vi "Run_old.vi"(8 "error in (no error)":errorcluster, 11 "Channel in":refnum<class "Channel.lvclass">) -> (0 "error out":errorcluster, 3 "Channel out":refnum<class "Channel.lvclass">)   [LabVIEW 2018, in "Channel.lvclass"]
uses:
  Channel.lvclass
  C:/Users/observer/Desktop/Sparc4GUI/SPARC4_GUI/Device/Device.lvclass
  Channel.lvclass/Channel.ctl
  Interface/Interface.lvclass/Interface.ctl
  Device/Device.lvclass/Device.ctl
  StateMachine/State Machine.lvclass
  Interface/Interface.lvclass
  Device/Device.lvclass
panel:
  out "resp RESUME":string
  out "resp PAUSE":string
  out "error out 2":errorcluster
  out "x = y?":T1
  out "resp ABORT":string
  out "resp STOP":string
  out "resposta do STATUS":string
  out "resp INIT":string
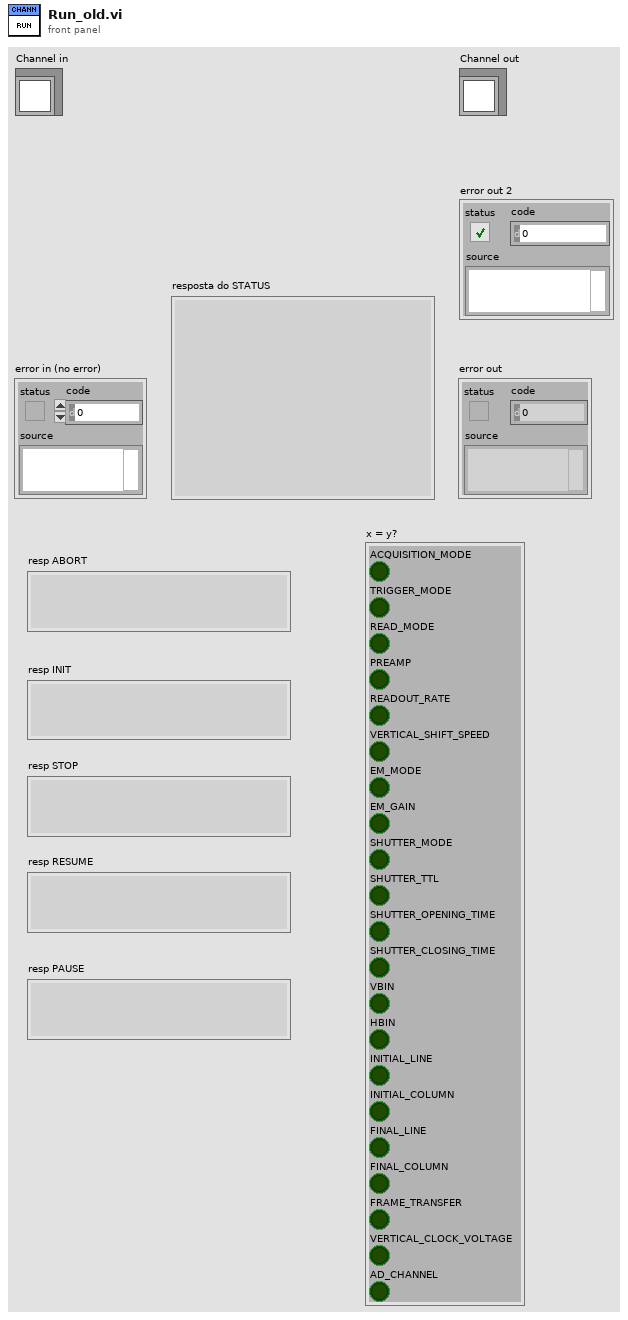
[diagram p1: front panel]
types:
  T1 = cluster{"ACQUISITION_MODE":bool, "TRIGGER_MODE":bool, "READ_MODE":bool, "PREAMP":bool, "READOUT_RATE":bool, "VERTICAL_SHIFT_SPEED":bool, "EM_MODE":bool, "EM_GAIN":bool, "SHUTTER_MODE":bool, "SHUTTER_TTL":bool, "SHUTTER_OPENING_TIME":bool, "SHUTTER_CLOSING_TIME":bool, "VBIN":bool, "HBIN":bool, "INITIAL_LINE":bool, "INITIAL_COLUMN":bool, "FINAL_LINE":bool, "FINAL_COLUMN":bool, "FRAME_TRANSFER":bool, "VERTICAL_CLOCK_VOLTAGE":bool, "AD_CHANNEL":bool}
  T2 = cluster{"ACQUISITION_MODE":u8, "TRIGGER_MODE":u8, "READ_MODE":u8, "PREAMP":u8, "READOUT_RATE":u8, "VERTICAL_SHIFT_SPEED":u8, "EM_MODE":u8, "EM_GAIN":u16, "SHUTTER_MODE":u8, "SHUTTER_TTL":u8, "SHUTTER_OPENING_TIME":u16, "SHUTTER_CLOSING_TIME":u16, "VBIN":u16, "HBIN":u16, "INITIAL_LINE":u16, "INITIAL_COLUMN":u16, "FINAL_LINE":u16, "FINAL_COLUMN":u16, "FRAME_TRANSFER":bool, "VERTICAL_CLOCK_VOLTAGE":u8, "AD_CHANNEL":u32}
  T3 = cluster{"Image Name":string, "Image Path":string, "#FRAMES":u32, "EXPTIME":dbl, "PREAMP":u8, "READOUT_RATE":u8, "VERTICAL_SHIFT_SPEED":u8, "ACQUISITION_MODE":u8, "READ_MODE":u8, "EM_MODE":u8, "EM_GAIN":u16, "SHUTTER_MODE":u8, "SHUTTER_TTL":u8, "SHUTTER_OPENNING_TIME":u16, "SHUTTER_CLOSING_TIME":u16, "VBIN":u16, "HBIN":u16, "INITIAL_LINE":u16, "INITIAL_COLUMN":u16, "FINAL_LINE":u16, "FINAL_COLUMN":u16, "Cooler ON/OFF":u16, "Set temperature":i8, "Exposições realizadas":u16, "Kinetic Serie Length":u32, "Number of Accumulations":u32, "Kinetic Cycle Time":u32, "FRAME_TRANSFER":bool, "VERTICAL_CLOCK_VOLTAGE":u8, "TRIGGER_MODE":u8, "Number of exp":u32, "AD_CHANNEL":u32}
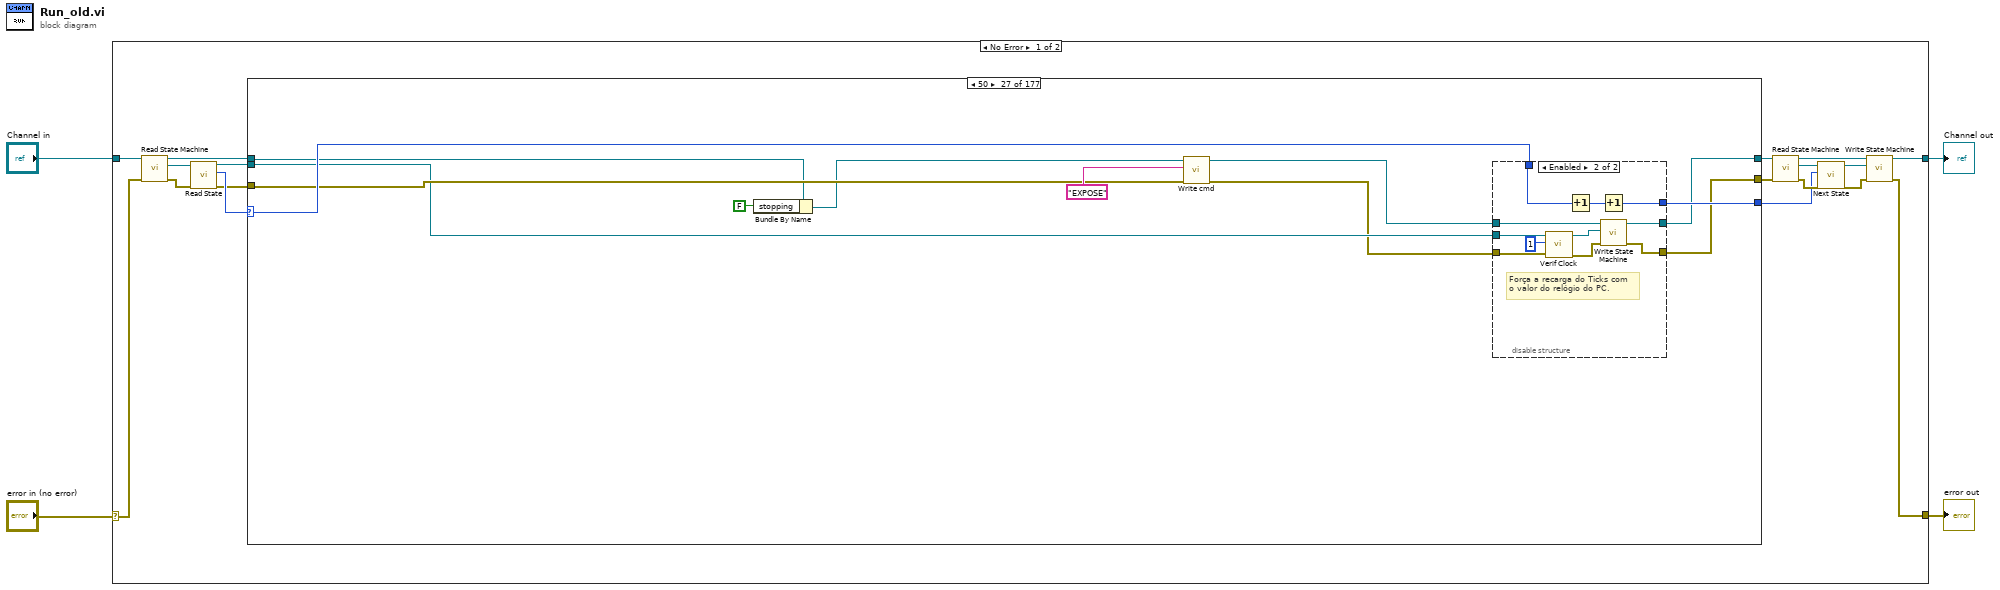
[diagram p0: block diagram]
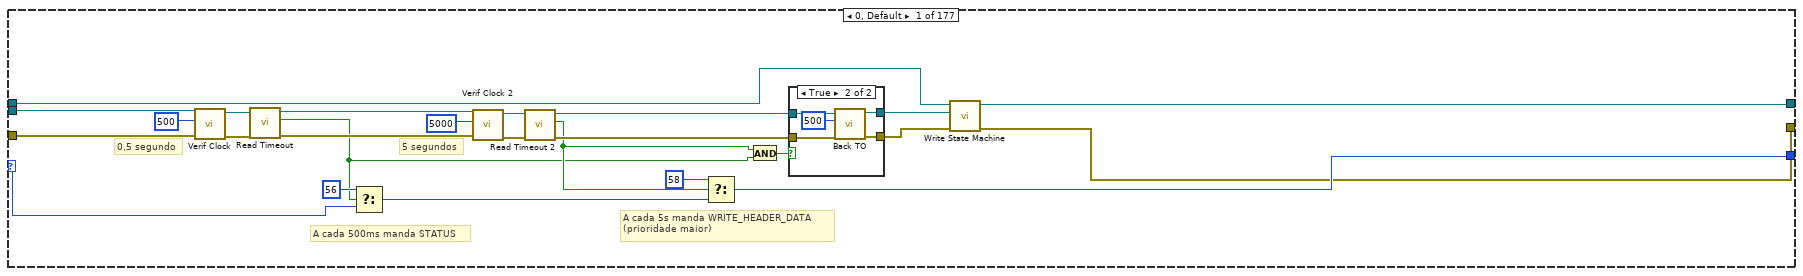
[diagram p2: hidden frame]
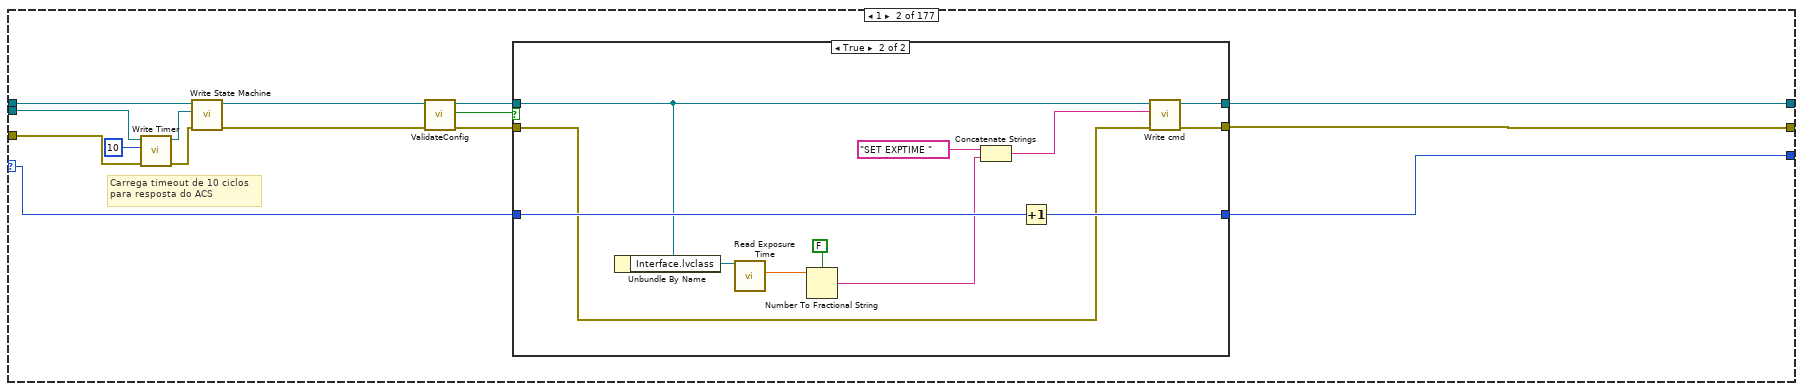
[diagram p4: hidden frame]
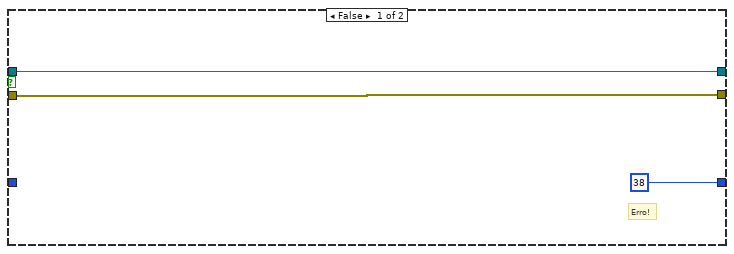
[diagram p5: hidden frame]
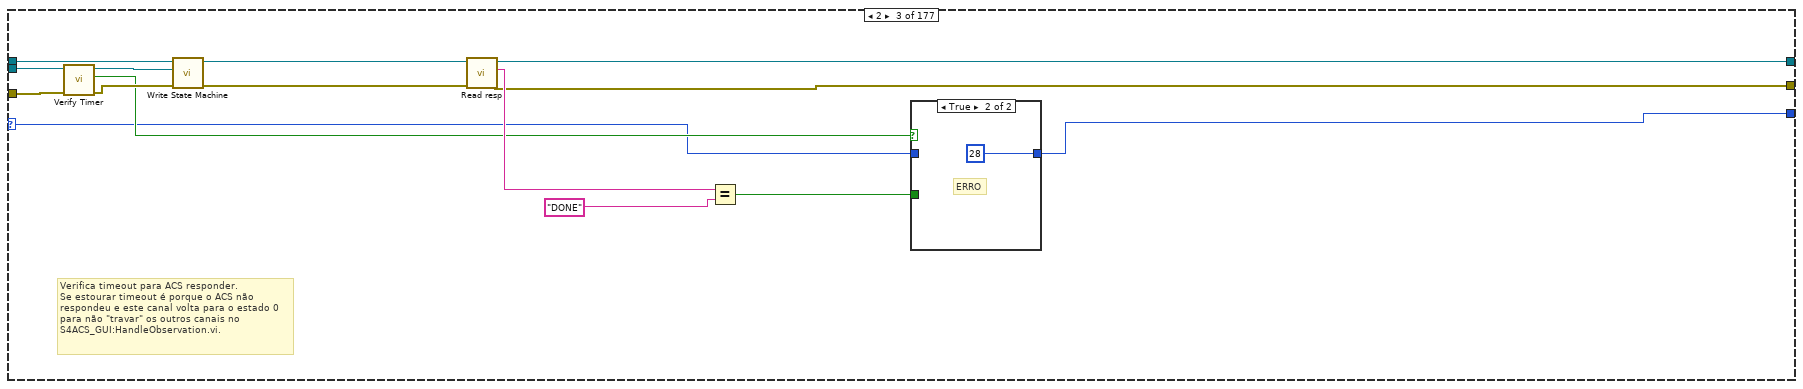
[diagram p6: hidden frame]
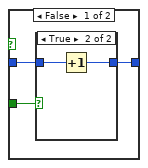
[diagram p7: hidden frame]
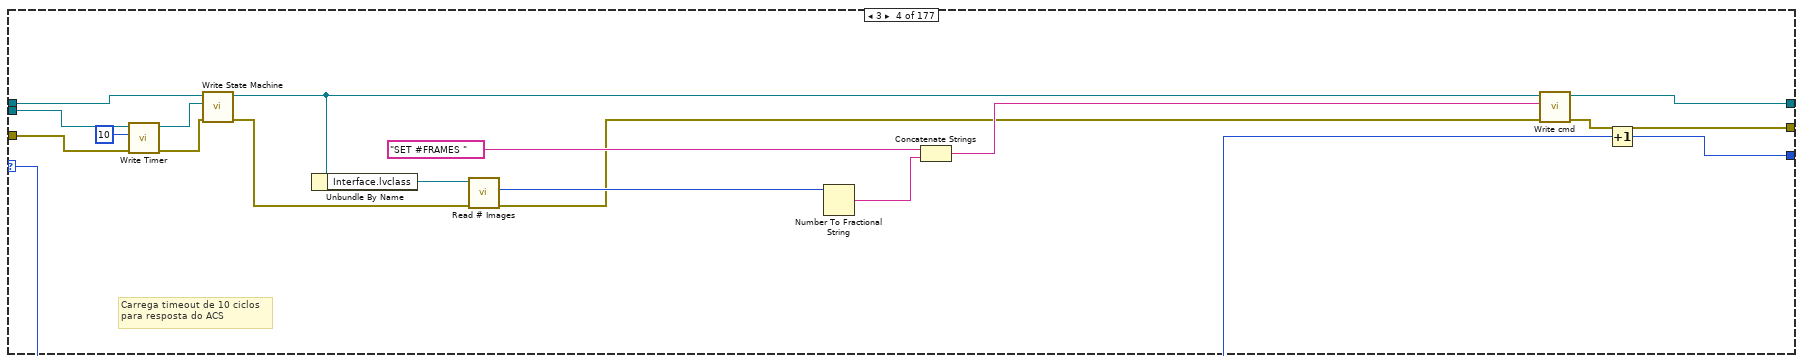
[diagram p9: hidden frame]
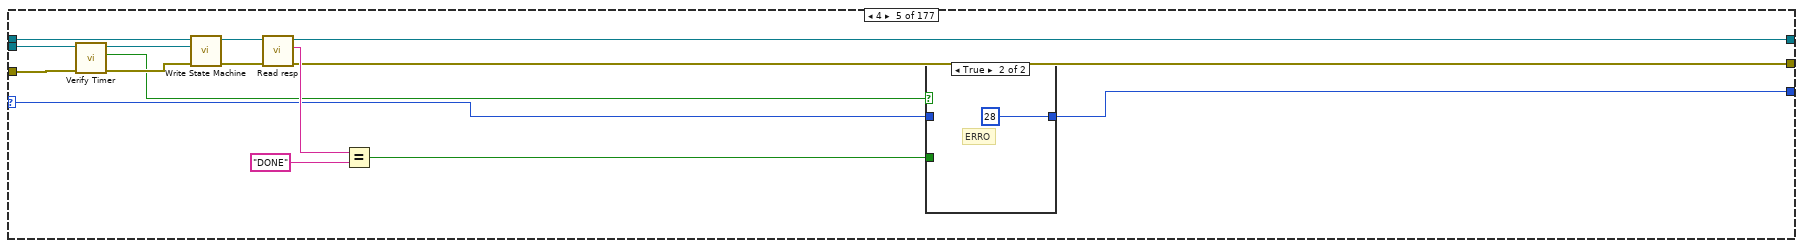
[diagram p10: hidden frame]
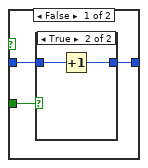
[diagram p11: hidden frame]
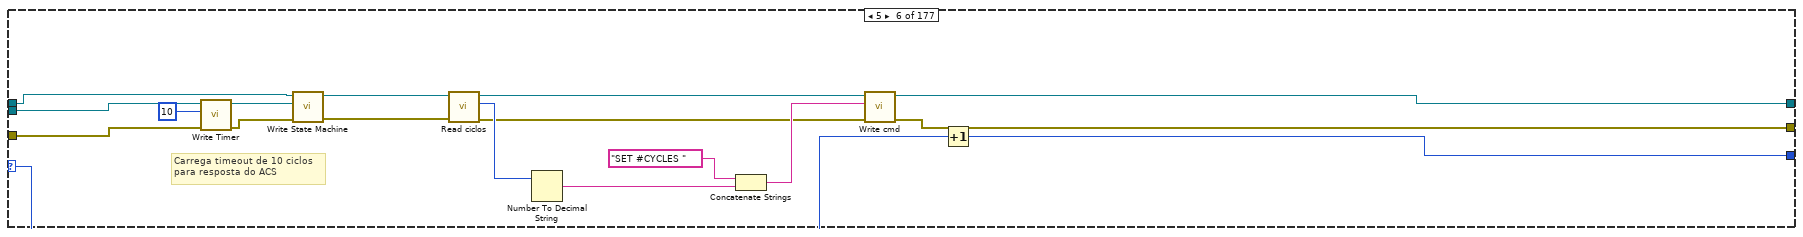
[diagram p13: hidden frame]
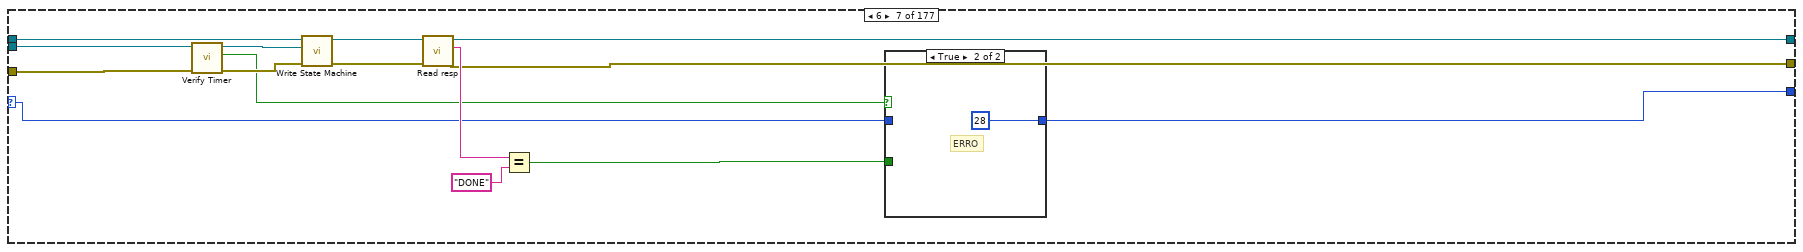
[diagram p14: hidden frame]
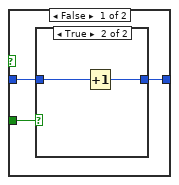
[diagram p15: hidden frame]
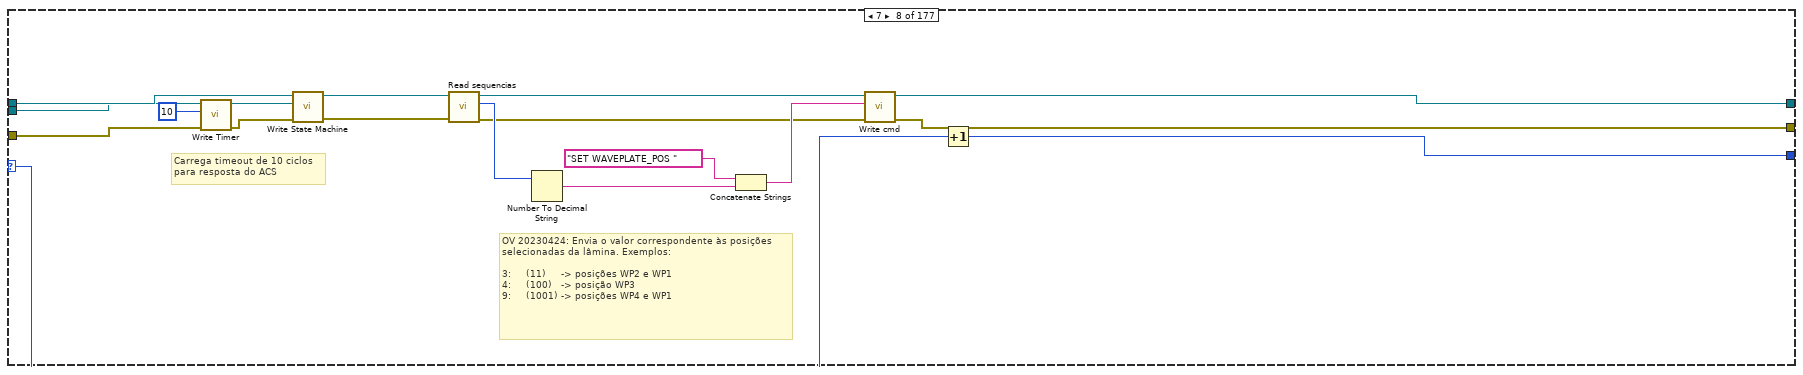
[diagram p17: hidden frame]
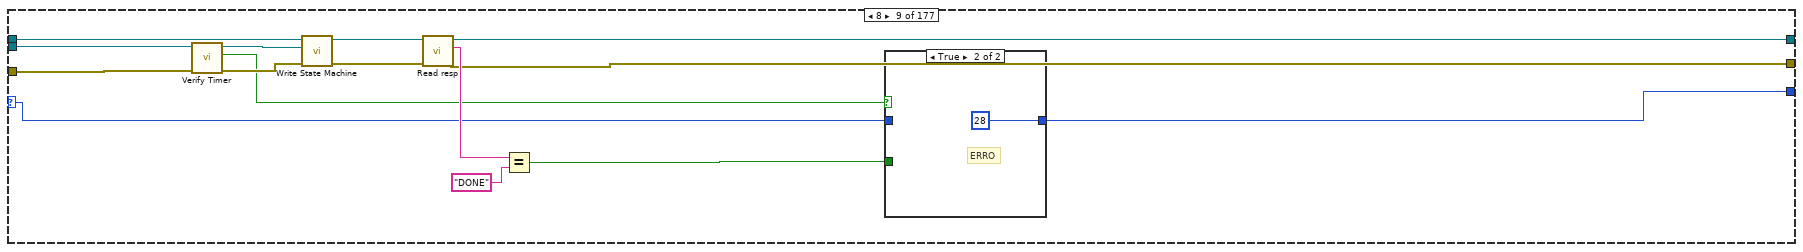
[diagram p18: hidden frame]
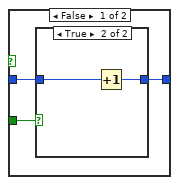
[diagram p19: hidden frame]
diagram:
  n1 = case shown="No Error" "error in (no error)" {
    selector: "error in (no error)" -> [w21 w2909]
    tunnel: [w6 w2909] -> w3
    tunnel: [w11 w2908] -> w1
    tunnel: "Channel in" -> [w22 w2908]
    frame No Error {
      n2 = call-dynamic "Read State Machine.vi"("error in (no error)"=w21, "Device in"=w22) -> ("error out"=w18:errorcluster, "State Machine.lvclass"=w20:refnum<class "State Machine.lvclass">, "Device out"=w16:refnum<class "Channel.lvclass">)  [unwired: 7 in]
      n3 = call-dynamic "Read State.vi"("error in (no error)"=w18, "State Machine in"=w20) -> ("error out"=w17:errorcluster, "State"=w19:i32, "State Machine out"=w5:refnum<class "State Machine.lvclass">)  [unwired: 7 in]
      n4 = case shown="50" w19 {
        selector: w19 -> [w43 w66 w86 w109 w126 w155 w167 w195 w207 w244 w252 w278 w290 w320 w334 w359 w365 w381 w397 w422 w435 w471 w490 _ w518 _ w555 w585 w597 w645 w665 w723 w789 w837 _ _ w928 w960 w989 w1001 w1015 w1020 w1080 w1102 w1140 w1146 w1160 w1168 w1182 w1189 w1200 _ w1215 w1226 w1246 w1266 w1286 w1306 w1326 w1346 w1366 w1386 _ w1406 w1414 w1427 w1440 w1456 w1464 w1477 w1491 w1503 w1511 w1524 w1537 w1549 w1557 w1570 w1583 w1595 w1603 w1616 w1629 w1641 w1649 w1662 w1675 w1687 w1695 w1708 w1721 w1733 w1741 w1754 w1767 w1779 w1787 w1800 w1813 w1829 w1837 w1850 w1863 w1875 w1883 w1896 w1909 w1921 w1929 w1942 w1955 w1967 w1975 w1988 w2001 w2013 w2021 w2034 w2047 w2059 w2067 w2080 w2093 w2105 w2113 w2126 w2139 w2151 w2159 w2172 w2185 w2197 w2205 w2218 w2231 w2243 w2251 w2264 w2277 w2289 w2297 w2310 w2323 w2339 w2347 w2360 w2373 w2385 w2395 w2408 w2421 w2435 w2443 w2456 w2469 w2487 w2502 w2526 w2534 w2565 w2573 w2604 w2612 w2643 w2651 w2682 w2690 w2725 w2738 w2767 w2773 w2799 w2811 w2836 w2848 w2873 w2885]
        tunnel: w17 -> [w41 w65 w92 w111 w130 w157 w169 w197 w209 w229 w254 w280 w292 w322 w336 w361 w363 w373 w396 w417 w429 w481 w489 w511 w520 w531 w552 w578 w594 w602 w662 w682 w781 w809 w871 w903 w936 w948 w983 w996 w1009 w1037 w1077 w1097 w1133 w1150 w1163 w1172 w1185 w1192 w1203 w1212 w1219 w1230 w1241 w1261 w1281 w1301 w1321 w1341 w1361 w1381 w1399 w1412 w1421 w1431 w1443 w1462 w1471 w1481 w1494 w1509 w1518 w1528 w1540 w1555 w1564 w1574 w1586 w1601 w1610 w1620 w1632 w1647 w1656 w1666 w1678 w1693 w1702 w1712 w1724 w1739 w1748 w1758 w1770 w1785 w1794 w1804 w1816 w1835 w1844 w1854 w1866 w1881 w1890 w1900 w1912 w1927 w1936 w1946 w1958 w1973 w1982 w1992 w2004 w2019 w2028 w2038 w2050 w2065 w2074 w2084 w2096 w2111 w2120 w2130 w2142 w2157 w2166 w2176 w2188 w2203 w2212 w2222 w2234 w2249 w2258 w2268 w2280 w2295 w2304 w2314 w2326 w2345 w2354 w2364 w2376 w2391 w2402 w2412 w2424 w2441 w2450 w2460 w2472 w2479 w2500 w2518 w2540 w2558 w2579 w2597 w2618 w2636 w2657 w2675 w2696 w2719 w2744 w2761 w2779 w2801 w2813 w2838 w2850 w2875 w2887]
        tunnel: [w23 w68 w96 w123 w136 w163 w176 w203 w216 w246 w261 w286 w299 w328 w343 w361 w363 w385 w398 w424 w437 w480 w491 w516 w520 w535 w547 w572 w599 w637 w667 w696 w776 w810 w883 w914 w935 w961 w991 w993 w1017 w1021 w1082 w1103 w1121 w1147 w1156 w1169 w1178 w1190 w1196 w1205 w1218 w1227 w1241 w1261 w1281 w1301 w1321 w1341 w1361 w1381 w1399 w1411 w1415 w1430 w1441 w1461 w1465 w1480 w1492 w1508 w1512 w1527 w1538 w1554 w1558 w1573 w1584 w1600 w1604 w1619 w1630 w1646 w1650 w1665 w1676 w1692 w1696 w1711 w1722 w1738 w1742 w1757 w1768 w1784 w1788 w1803 w1814 w1834 w1838 w1853 w1864 w1880 w1884 w1899 w1910 w1926 w1930 w1945 w1956 w1972 w1976 w1991 w2002 w2018 w2022 w2037 w2048 w2064 w2068 w2083 w2094 w2110 w2114 w2129 w2140 w2156 w2160 w2175 w2186 w2202 w2206 w2221 w2232 w2248 w2252 w2267 w2278 w2294 w2298 w2313 w2324 w2344 w2348 w2363 w2374 w2390 w2396 w2411 w2422 w2440 w2444 w2459 w2470 w2491 w2503 w2530 w2543 w2569 w2582 w2608 w2621 w2647 w2660 w2686 w2699 w2728 w2747 w2769 w2782 w2807 w2820 w2844 w2857 w2881 w2894] -> w7
        tunnel: w16 -> [w31 w63 w95 w112 w134 w158 w173 w198 w213 w231 w258 w281 w296 w323 w340 w360 w362 w376 w395 w419 w432 w479 w488 w514 w519 w532 w546 w584 w595 w617 w658 w695 w783 w803 w882 w913 w930 w952 w984 w997 w1010 w1038 w1076 w1100 w1134 w1151 w1162 w1173 w1184 w1193 w1202 w1213 w1217 w1231 w1239 w1259 w1279 w1299 w1319 w1339 w1359 w1379 w1401 w1410 w1422 w1429 w1444 w1460 w1472 w1479 w1495 w1507 w1519 w1526 w1541 w1553 w1565 w1572 w1587 w1599 w1611 w1618 w1633 w1645 w1657 w1664 w1679 w1691 w1703 w1710 w1725 w1737 w1749 w1756 w1771 w1783 w1795 w1802 w1817 w1833 w1845 w1852 w1867 w1879 w1891 w1898 w1913 w1925 w1937 w1944 w1959 w1971 w1983 w1990 w2005 w2017 w2029 w2036 w2051 w2063 w2075 w2082 w2097 w2109 w2121 w2128 w2143 w2155 w2167 w2174 w2189 w2201 w2213 w2220 w2235 w2247 w2259 w2266 w2281 w2293 w2305 w2312 w2327 w2343 w2355 w2362 w2377 w2389 w2403 w2410 w2425 w2439 w2451 w2458 w2473 w2481 w2499 w2520 w2541 w2560 w2580 w2599 w2619 w2638 w2658 w2677 w2697 w2721 w2745 w2763 w2780 w2802 w2817 w2839 w2854 w2876 w2891]
        tunnel: [w30 w69 w97 w124 w137 w164 w177 w204 w217 w247 w262 w287 w300 w329 w344 w360 w362 w386 w399 w425 w440 w472 w492 w517 w519 w536 w548 w573 w600 w644 w668 w722 w777 w836 w884 w915 w937 w962 w992 w994 w1018 w1033 w1083 w1104 w1127 w1148 w1155 w1170 w1177 w1191 w1195 w1211 w1220 w1223 w1243 w1263 w1283 w1303 w1323 w1343 w1363 w1383 w1401 w1413 w1416 w1432 w1439 w1463 w1466 w1482 w1490 w1510 w1513 w1529 w1536 w1556 w1559 w1575 w1582 w1602 w1605 w1621 w1628 w1648 w1651 w1667 w1674 w1694 w1697 w1713 w1720 w1740 w1743 w1759 w1766 w1786 w1789 w1805 w1812 w1836 w1839 w1855 w1862 w1882 w1885 w1901 w1908 w1928 w1931 w1947 w1954 w1974 w1977 w1993 w2000 w2020 w2023 w2039 w2046 w2066 w2069 w2085 w2092 w2112 w2115 w2131 w2138 w2158 w2161 w2177 w2184 w2204 w2207 w2223 w2230 w2250 w2253 w2269 w2276 w2296 w2299 w2315 w2322 w2346 w2349 w2365 w2372 w2392 w2397 w2413 w2420 w2442 w2445 w2461 w2468 w2492 w2504 w2531 w2544 w2570 w2583 w2609 w2622 w2648 w2661 w2687 w2700 w2729 w2748 w2770 w2783 w2808 w2821 w2845 w2858 w2882 w2895] -> w14
        tunnel: [w40 w67 w85 w118 w125 w162 w168 w202 w208 w245 w250 w285 w291 w327 w332 w359 w366 w382 w400 w423 w436 w473 w493 31 ("State") w518 0 ("State") w553 w586 w598 w646 w666 w724 w790 w838 0 ("State") 54 ("State") w927 w963 w990 w1002 w1016 w1019 w1081 w1105 w1141 w1149 w1161 w1171 w1183 w1189 w1201 w1204 w1216 w1228 w1238 w1258 w1278 w1298 w1318 w1338 w1358 w1378 u8 0 ("State") w1407 w1417 w1428 w1442 w1457 w1467 w1478 w1493 w1504 w1514 w1525 w1539 w1550 w1560 w1571 w1585 w1596 w1606 w1617 w1631 w1642 w1652 w1663 w1677 w1688 w1698 w1709 w1723 w1734 w1744 w1755 w1769 w1780 w1790 w1801 w1815 w1830 w1840 w1851 w1865 w1876 w1886 w1897 w1911 w1922 w1932 w1943 w1957 w1968 w1978 w1989 w2003 w2014 w2024 w2035 w2049 w2060 w2070 w2081 w2095 w2106 w2116 w2127 w2141 w2152 w2162 w2173 w2187 w2198 w2208 w2219 w2233 w2244 w2254 w2265 w2279 w2290 w2300 w2311 w2325 w2340 w2350 w2361 w2375 w2386 w2398 w2409 w2423 w2436 w2446 w2457 w2471 w2488 w2505 w2527 w2532 w2566 w2571 w2605 w2610 w2644 w2649 w2683 w2688 w2726 w2736 w2768 w2771 w2806 w2812 w2843 w2849 w2880 w2883] -> w8
        tunnel: w5 -> [w42 w64 w94 w113 w135 w156 w170 w196 w210 w227 w255 w279 w293 w321 w337 _ _ w375 w393 w418 w433 _ w486 w513 _ w533 w551 w582 _ w605 w663 w685 w785 w808 w872 w904 w932 w953 w986 w998 w1012 w1039 w1078 w1101 w1135 _ _ _ _ _ _ w1207 _ _ _ _ _ _ _ _ _ _ _ _ _ _ _ _ _ _ _ _ _ _ _ _ _ _ _ _ _ _ _ _ _ _ _ _ _ _ _ _ _ _ _ _ _ _ _ _ _ _ _ _ _ _ _ _ _ _ _ _ _ _ _ _ _ _ _ _ _ _ _ _ _ _ _ _ _ _ _ _ _ _ _ _ _ _ _ _ _ _ _ _ _ _ _ _ _ _ _ _ _ _ _ w2483 w2501 w2515 w2538 w2554 w2577 w2593 w2616 w2632 w2655 w2671 w2694 w2717 w2742 w2760 w2777 w2800 w2814 w2837 w2851 w2874 w2888]
        frame 0, Default {
          # "5 segundos"
          # "A cada 5s manda WRITE_HEADER_DATA\n(prioridade maior)"
          # "A cada 500ms manda STATUS"
          # "0,5 segundo"
          n5 = call-dynamic "Verif Clock.vi"("error in (no error)"=w41, "period (ms)"=u32 500 ("period"), "State Machine in"=w42) -> ("error out"=w46:errorcluster, "State Machine out"=w45:refnum<class "State Machine.lvclass">)  [unwired: 6 in, 1 out]
          n6 = call-dynamic "Read Timeout.vi"("error in (no error)"=w46, "State Machine in"=w45) -> ("error out"=w35:errorcluster, "Timeout"=w24:bool, "State Machine out"=w37:refnum<class "State Machine.lvclass">)  [unwired: 7 in]
          n7 = Select(t=56 ("State"), s=w24, f=w43) -> (s? t:f=w38:i32)
          n8 = call-dynamic "Verif Clock 2.vi"("error in (no error)"=w35, "period (ms)"=u32 5000 ("period"), "State Machine in"=w37) -> ("error out"=w34:errorcluster, "State Machine out"=w36:refnum<class "State Machine.lvclass">)  [unwired: 6 in, 1 out]
          n9 = call-dynamic "Read Timeout 2.vi"("error in (no error)"=w34, "State Machine in"=w36) -> ("error out"=w32:errorcluster, "Timeout 2"=w25:bool, "State Machine out"=w28:refnum<class "State Machine.lvclass">)  [unwired: 7 in]
          n10 = Select(t=58 ("f"), s=w25, f=w38) -> (s? t:f=w40:i32)
          n11 = And(x=w25, y=w24) -> (x .and. y?=w26:bool)
          n12 = case shown="True" w26 {
            tunnel: w32 -> [w48 w54]
            tunnel: [w48 w53] -> w29
            tunnel: w28 -> [w49 w52]
            tunnel: [w49 w51] -> w27
            frame False {
            }
            frame True {
              n13 = call-dynamic "Back TO.vi"("error in (no error)"=w54, "time back (ms)"=u32 500 ("time(ms)"), "State Machine in"=w52) -> ("error out"=w53:errorcluster, "State Machine out"=w51:refnum<class "State Machine.lvclass">)  [unwired: 7 in]
            }
          }
          n14 = call-dynamic "Write State Machine.vi"("error in (no error)"=w29, "State Machine.lvclass"=w27, "Device in"=w31) -> ("error out"=w23:errorcluster, "Device out"=w30:refnum<class "Channel.lvclass">)  [unwired: 7 in]
        }
        frame 1 {
          # "Carrega timeout de 10 ciclos\npara resposta do ACS"
          n15 = call-dynamic "Write Timer.vi"("error in (no error)"=w65, "Timer"=u32 10, "State Machine in"=w64) -> ("error out"=w60:errorcluster, "State Machine out"=w62:refnum<class "State Machine.lvclass">)  [unwired: 7 in]
          n16 = call-dynamic "Write State Machine.vi"("error in (no error)"=w60, "State Machine.lvclass"=w62, "Device in"=w63) -> ("error out"=w58:errorcluster, "Device out"=w59:refnum<class "Channel.lvclass">)  [unwired: 7 in]
          n17 = call-dynamic "ValidateConfig.vi"("error in (no error)"=w58, "Channel in"=w59) -> ("error out"=w56:errorcluster, "valid?"=w55:bool, "Channel out"=w57:refnum<class "Channel.lvclass">)  [unwired: 7 in]
          n18 = case shown="True" w55 {
            tunnel: [w72 w84] -> w69
            tunnel: [w71 w83] -> w68
            tunnel: [38 w82] -> w67
            tunnel: w66 -> [_ w81]
            tunnel: w57 -> [w72 w74]
            tunnel: w56 -> [w71 w73]
            frame False {
              # "Erro!"
            }
            frame True {
              n19 = Unbundle By Name(w74) -> ("Interface.lvclass"=w80:refnum<class "Interface.lvclass">)
              n20 = call "Read Exposure Time.vi"("Interface in"=w80) -> ("Exposure Time"=w79:dbl)  [unwired: 8 in, 2 out]
              n21 = Number To Fractional String(use system decimal point (T)=FALSE, number=w79) -> (F-format string=w78:string)  [unwired: 2 in]
              n22 = Concatenate Strings("SET EXPTIME " ("cmd"), w78) -> (w77:string)
              n23 = Increment(x=w81) -> (x+1=w82:i32)
              n24 = call-dynamic "Write cmd.vi"("error in (no error)"=w73, "cmd"=w77, "Device in"=w74) -> ("error out"=w83:errorcluster, "Device out"=w84:refnum<class "Channel.lvclass">)  [unwired: 7 in]
            }
          }
        }
        frame 2 {
          # "Verifica timeout para ACS responder.\nSe estourar timeout é porque o ACS não \nrespondeu e este canal volta para o estado 0\npara não \"travar\" os outros canais no \nS4ACS_GUI:HandleObservation.vi."
          n25 = call "Verify Timer.vi"("error in (no error)"=w92, "State Machine in"=w94) -> ("error out"=w91:errorcluster, "timeout"=w87:bool, "State Machine out"=w93:refnum<class "State Machine.lvclass">)  [unwired: 7 in]
          n26 = call-dynamic "Write State Machine.vi"("error in (no error)"=w91, "State Machine.lvclass"=w93, "Device in"=w95) -> ("error out"=w90:errorcluster, "Device out"=w89:refnum<class "Channel.lvclass">)  [unwired: 7 in]
          n27 = call-dynamic "Read resp.vi"("error in (no error)"=w90, "Device in"=w89) -> ("error out"=w96:errorcluster, "resp"=w99:string, "Device out"=w97:refnum<class "Channel.lvclass">)  [unwired: 7 in]
          n28 = Equal?(x=w99, y="DONE") -> (x = y?=w88:bool)
          n29 = case shown="True" w87 {
            tunnel: [w101 28] -> w85
            tunnel: w86 -> [w102 _]
            tunnel: w88 -> [w100 _]
            frame False {
              n30 = case shown="True" w100 {
                tunnel: [w103 w104] -> w101
                tunnel: w102 -> [w103 w105]
                frame False {
                }
                frame True {
                  n31 = Increment(x=w105) -> (x+1=w104:i32)
                }
              }
            }
            frame True {
              # "ERRO"
            }
          }
        }
        frame 3 {
          # "Carrega timeout de 10 ciclos\npara resposta do ACS"
          n32 = call-dynamic "Write Timer.vi"("error in (no error)"=w111, "Timer"=u32 10, "State Machine in"=w113) -> ("error out"=w114:errorcluster, "State Machine out"=w116:refnum<class "State Machine.lvclass">)  [unwired: 7 in]
          n33 = call-dynamic "Write State Machine.vi"("error in (no error)"=w114, "State Machine.lvclass"=w116, "Device in"=w112) -> ("error out"=w108:errorcluster, "Device out"=w110:refnum<class "Channel.lvclass">)  [unwired: 7 in]
          n34 = Unbundle By Name(w110) -> ("Interface.lvclass"=w122:refnum<class "Interface.lvclass">)
          n35 = call-dynamic "Read # Images.vi"("error in (no error)"=w108, "Interface in"=w122) -> ("error out"=w107:errorcluster, "# Images"=w121:u32)  [unwired: 7 in, 1 out]
          n36 = Number To Fractional String(number=w121) -> (F-format string=w120:string)  [unwired: 3 in]
          n37 = Concatenate Strings("SET #FRAMES " ("cmd"), w120) -> (w119:string)
          n38 = call-dynamic "Write cmd.vi"("error in (no error)"=w107, "cmd"=w119, "Device in"=w110) -> ("error out"=w123:errorcluster, "Device out"=w124:refnum<class "Channel.lvclass">)  [unwired: 7 in]
          n39 = Increment(x=w109) -> (x+1=w118:i32)
        }
        frame 4 {
          n40 = call "Verify Timer.vi"("error in (no error)"=w130, "State Machine in"=w135) -> ("error out"=w129:errorcluster, "timeout"=w128:bool, "State Machine out"=w131:refnum<class "State Machine.lvclass">)  [unwired: 7 in]
          n41 = call-dynamic "Write State Machine.vi"("error in (no error)"=w129, "State Machine.lvclass"=w131, "Device in"=w134) -> ("error out"=w132:errorcluster, "Device out"=w133:refnum<class "Channel.lvclass">)  [unwired: 7 in]
          n42 = call-dynamic "Read resp.vi"("error in (no error)"=w132, "Device in"=w133) -> ("error out"=w136:errorcluster, "resp"=w139:string, "Device out"=w137:refnum<class "Channel.lvclass">)  [unwired: 7 in]
          n43 = Equal?(x=w139, y="DONE") -> (x = y?=w127:bool)
          n44 = case shown="True" w128 {
            tunnel: [w141 28] -> w125
            tunnel: w126 -> [w142 _]
            tunnel: w127 -> [w140 _]
            frame False {
              n45 = case shown="True" w140 {
                tunnel: [w143 w144] -> w141
                tunnel: w142 -> [w143 w145]
                frame False {
                }
                frame True {
                  n46 = Increment(x=w145) -> (x+1=w144:i32)
                }
              }
            }
            frame True {
              # "ERRO"
            }
          }
        }
        frame 5 {
          # "Carrega timeout de 10 ciclos\npara resposta do ACS"
          n47 = call-dynamic "Write Timer.vi"("error in (no error)"=w157, "Timer"=u32 10, "State Machine in"=w156) -> ("error out"=w159:errorcluster, "State Machine out"=w161:refnum<class "State Machine.lvclass">)  [unwired: 7 in]
          n48 = call-dynamic "Write State Machine.vi"("error in (no error)"=w159, "State Machine.lvclass"=w161, "Device in"=w158) -> ("error out"=w153:errorcluster, "Device out"=w154:refnum<class "Channel.lvclass">)  [unwired: 7 in]
          n49 = call-dynamic "Read ciclos.vi"("error in (no error)"=w153, "Channel in"=w154) -> ("error out"=w147:errorcluster, "ciclos"=w151:u32, "Channel out"=w152:refnum<class "Channel.lvclass">)  [unwired: 7 in]
          n50 = Number To Decimal String(number=w151) -> (decimal integer string=w149:string)  [unwired: 1 in]
          n51 = Concatenate Strings("SET #CYCLES " ("cmd"), w149) -> (w148:string)
          n52 = call-dynamic "Write cmd.vi"("error in (no error)"=w147, "cmd"=w148, "Device in"=w152) -> ("error out"=w163:errorcluster, "Device out"=w164:refnum<class "Channel.lvclass">)  [unwired: 7 in]
          n53 = Increment(x=w155) -> (x+1=w162:i32)
        }
        frame 6 {
          n54 = call "Verify Timer.vi"("error in (no error)"=w169, "State Machine in"=w170) -> ("error out"=w174:errorcluster, "timeout"=w166:bool, "State Machine out"=w175:refnum<class "State Machine.lvclass">)  [unwired: 7 in]
          n55 = call-dynamic "Write State Machine.vi"("error in (no error)"=w174, "State Machine.lvclass"=w175, "Device in"=w173) -> ("error out"=w171:errorcluster, "Device out"=w172:refnum<class "Channel.lvclass">)  [unwired: 7 in]
          n56 = call-dynamic "Read resp.vi"("error in (no error)"=w171, "Device in"=w172) -> ("error out"=w176:errorcluster, "resp"=w179:string, "Device out"=w177:refnum<class "Channel.lvclass">)  [unwired: 7 in]
          n57 = Equal?(x=w179, y="DONE") -> (x = y?=w165:bool)
          n58 = case shown="True" w166 {
            tunnel: [w181 28] -> w168
            tunnel: w167 -> [w182 _]
            tunnel: w165 -> [w180 _]
            frame False {
              n59 = case shown="True" w180 {
                tunnel: [w183 w184] -> w181
                tunnel: w182 -> [w183 w185]
                frame False {
                }
                frame True {
                  n60 = Increment(x=w185) -> (x+1=w184:i32)
                }
              }
            }
            frame True {
              # "ERRO"
            }
          }
        }
        frame 7 {
          # "OV 20230424: Envia o valor correspondente às posições\nselecionadas da lâmina. Exemplos:\n\n3:     (11)     -> posições WP2 e WP1\n4:     (100)   -> posição WP3\n9:     (1001) -> posições WP4 e WP1"
          # "Carrega timeout de 10 ciclos\npara resposta do ACS"
          n61 = call-dynamic "Write Timer.vi"("error in (no error)"=w197, "Timer"=u32 10, "State Machine in"=w196) -> ("error out"=w199:errorcluster, "State Machine out"=w201:refnum<class "State Machine.lvclass">)  [unwired: 7 in]
          n62 = call-dynamic "Write State Machine.vi"("error in (no error)"=w199, "State Machine.lvclass"=w201, "Device in"=w198) -> ("error out"=w193:errorcluster, "Device out"=w194:refnum<class "Channel.lvclass">)  [unwired: 7 in]
          n63 = call-dynamic "Read sequencias.vi"("error in (no error)"=w193, "Channel in"=w194) -> ("error out"=w187:errorcluster, "sequencias"=w191:u32, "Channel out"=w192:refnum<class "Channel.lvclass">)  [unwired: 7 in]
          n64 = Number To Decimal String(number=w191) -> (decimal integer string=w189:string)  [unwired: 1 in]
          n65 = Concatenate Strings("SET WAVEPLATE_POS " ("cmd"), w189) -> (w188:string)
          n66 = call-dynamic "Write cmd.vi"("error in (no error)"=w187, "cmd"=w188, "Device in"=w192) -> ("error out"=w203:errorcluster, "Device out"=w204:refnum<class "Channel.lvclass">)  [unwired: 7 in]
          n67 = Increment(x=w195) -> (x+1=w202:i32)
        }
        frame 8 {
          n68 = call "Verify Timer.vi"("error in (no error)"=w209, "State Machine in"=w210) -> ("error out"=w214:errorcluster, "timeout"=w206:bool, "State Machine out"=w215:refnum<class "State Machine.lvclass">)  [unwired: 7 in]
          n69 = call-dynamic "Write State Machine.vi"("error in (no error)"=w214, "State Machine.lvclass"=w215, "Device in"=w213) -> ("error out"=w211:errorcluster, "Device out"=w212:refnum<class "Channel.lvclass">)  [unwired: 7 in]
          n70 = call-dynamic "Read resp.vi"("error in (no error)"=w211, "Device in"=w212) -> ("error out"=w216:errorcluster, "resp"=w219:string, "Device out"=w217:refnum<class "Channel.lvclass">)  [unwired: 7 in]
          n71 = Equal?(x=w219, y="DONE") -> (x = y?=w205:bool)
          n72 = case shown="True" w206 {
            tunnel: [w221 28] -> w208
            tunnel: w207 -> [w222 _]
            tunnel: w205 -> [w220 _]
            frame False {
              n73 = case shown="True" w220 {
                tunnel: [w223 w224] -> w221
                tunnel: w222 -> [w223 w225]
                frame False {
                }
                frame True {
                  n74 = Increment(x=w225) -> (x+1=w224:i32)
                }
              }
            }
            frame True {
              # "ERRO"
            }
          }
        }
        frame 9 {
          # "Verifica valor de ASEL:"
          n75 = call-dynamic "Write Timer.vi"("error in (no error)"=w229, "Timer"=u32 50, "State Machine in"=w227) -> ("error out"=w234:errorcluster, "State Machine out"=w232:refnum<class "State Machine.lvclass">)  [unwired: 7 in]
          n76 = call-dynamic "Write State Machine.vi"("error in (no error)"=w234, "State Machine.lvclass"=w232, "Device in"=w231) -> ("error out"=w228:errorcluster, "Device out"=w230:refnum<class "Channel.lvclass">)  [unwired: 7 in]
          n77 = Unbundle By Name(w230) -> ("TCS telemetry"=w243:string)
          n78 = Match Pattern(string=w243, regular expression="\"ASEL\":") -> (after substring=w241:string)  [unwired: 1 in, 3 out]
          n79 = Match Pattern(string=w241, regular expression=",\"CALW\"") -> (before substring=w239:string)  [unwired: 1 in, 3 out]
          n80 = call <vilib>:"Trim Whitespace.vi"("string"=w239) -> ("trimmed string"=w238:string)  [unwired: 1 in]
          n81 = case shown="\"true\"" w238 {
            tunnel: ["PHOT" ("regular expression") "POLAR" ("regular expression")] -> w236
            frame "false", Default {
            }
            frame "true" {
            }
          }
          n82 = Concatenate Strings("SET INSTMODE " ("cmd"), w236) -> (w235:string)
          n83 = call-dynamic "Write cmd.vi"("error in (no error)"=w228, "cmd"=w235, "Device in"=w230) -> ("error out"=w246:errorcluster, "Device out"=w247:refnum<class "Channel.lvclass">)  [unwired: 7 in]
          n84 = Increment(x=w244) -> (x+1=w245:i32)
        }
        frame 10 {
          n85 = call "Verify Timer.vi"("error in (no error)"=w254, "State Machine in"=w255) -> ("error out"=w259:errorcluster, "timeout"=w253:bool, "State Machine out"=w260:refnum<class "State Machine.lvclass">)  [unwired: 7 in]
          n86 = call-dynamic "Write State Machine.vi"("error in (no error)"=w259, "State Machine.lvclass"=w260, "Device in"=w258) -> ("error out"=w256:errorcluster, "Device out"=w257:refnum<class "Channel.lvclass">)  [unwired: 7 in]
          n87 = call-dynamic "Read resp.vi"("error in (no error)"=w256, "Device in"=w257) -> ("error out"=w261:errorcluster, "resp"=w264:string, "Device out"=w262:refnum<class "Channel.lvclass">)  [unwired: 7 in]
          n88 = Equal?(x=w264, y="DONE") -> (x = y?=w251:bool)
          n89 = case shown="False" w253 {
            tunnel: [w266 28] -> w250
            tunnel: w252 -> [w267 _]
            tunnel: w251 -> [w265 _]
            frame False {
              n90 = case shown="True" w265 {
                tunnel: [w268 w269] -> w266
                tunnel: w267 -> [w268 w270]
                frame False {
                }
                frame True {
                  n91 = Increment(x=w270) -> (x+1=w269:i32)
                }
              }
            }
            frame True {
              # "ERRO"
            }
          }
        }
        frame 11 {
          # "Carrega timeout de 50 ciclos\npara resposta do ACS"
          n92 = call-dynamic "Write Timer.vi"("error in (no error)"=w280, "Timer"=u32 50, "State Machine in"=w279) -> ("error out"=w282:errorcluster, "State Machine out"=w284:refnum<class "State Machine.lvclass">)  [unwired: 7 in]
          n93 = call-dynamic "Write State Machine.vi"("error in (no error)"=w282, "State Machine.lvclass"=w284, "Device in"=w281) -> ("error out"=w275:errorcluster, "Device out"=w274:refnum<class "Channel.lvclass">)  [unwired: 7 in]
          n94 = Unbundle By Name(w274) -> ("Channel Status"=w273:u32)
          n95 = Number To Decimal String(number=w273) -> (decimal integer string=w272:string)  [unwired: 1 in]
          n96 = Concatenate Strings("SET CHANNELSTATUS " ("cmd"), w272) -> (w276:string)
          n97 = call-dynamic "Write cmd.vi"("error in (no error)"=w275, "cmd"=w276, "Device in"=w274) -> ("error out"=w286:errorcluster, "Device out"=w287:refnum<class "Channel.lvclass">)  [unwired: 7 in]
          n98 = Increment(x=w278) -> (x+1=w285:i32)
        }
        frame 12 {
          n99 = call "Verify Timer.vi"("error in (no error)"=w292, "State Machine in"=w293) -> ("error out"=w297:errorcluster, "timeout"=w289:bool, "State Machine out"=w298:refnum<class "State Machine.lvclass">)  [unwired: 7 in]
          n100 = call-dynamic "Write State Machine.vi"("error in (no error)"=w297, "State Machine.lvclass"=w298, "Device in"=w296) -> ("error out"=w294:errorcluster, "Device out"=w295:refnum<class "Channel.lvclass">)  [unwired: 7 in]
          n101 = call-dynamic "Read resp.vi"("error in (no error)"=w294, "Device in"=w295) -> ("error out"=w299:errorcluster, "resp"=w302:string, "Device out"=w300:refnum<class "Channel.lvclass">)  [unwired: 7 in]
          n102 = Equal?(x=w302, y="DONE") -> (x = y?=w288:bool)
          n103 = case shown="False" w289 {
            tunnel: [w304 w310] -> w291
            tunnel: w290 -> [w305 w309]
            tunnel: w288 -> [w303 _]
            frame False {
              n104 = case shown="True" w303 {
                tunnel: [w306 w307] -> w304
                tunnel: w305 -> [w306 w308]
                frame False {
                }
                frame True {
                  n105 = Increment(x=w308) -> (x+1=w307:i32)
                }
              }
            }
            frame True {
              n106 = disable-structure shown="Enabled" {
                disable-tunnel: [28 w312] -> w310
                disable-tunnel: w309 -> [_ w313]
                frame Disabled {
                  # "ERRO"
                }
                frame Enabled {
                  # "Por enquanto, prossegue\nmesmo sem receber DONE."
                  n107 = Increment(x=w313) -> (x+1=w312:i32)
                }
              }
            }
          }
        }
        frame 13 {
          # "Carrega timeout de 50 ciclos\npara resposta do ACS"
          n108 = call-dynamic "Write Timer.vi"("error in (no error)"=w322, "Timer"=u32 50, "State Machine in"=w321) -> ("error out"=w324:errorcluster, "State Machine out"=w326:refnum<class "State Machine.lvclass">)  [unwired: 7 in]
          n109 = call-dynamic "Write State Machine.vi"("error in (no error)"=w324, "State Machine.lvclass"=w326, "Device in"=w323) -> ("error out"=w317:errorcluster, "Device out"=w316:refnum<class "Channel.lvclass">)  [unwired: 7 in]
          n110 = Unbundle By Name(w316) -> ("syncmode"=w315:bool)
          n111 = case shown="False" w315 {
            tunnel: ["0" "1"] -> w314
            frame False {
            }
            frame True {
            }
          }
          n112 = Concatenate Strings("SET SYNCMODE " ("cmd"), w314) -> (w318:string)
          n113 = call-dynamic "Write cmd.vi"("error in (no error)"=w317, "cmd"=w318, "Device in"=w316) -> ("error out"=w328:errorcluster, "Device out"=w329:refnum<class "Channel.lvclass">)  [unwired: 7 in]
          n114 = Increment(x=w320) -> (x+1=w327:i32)
        }
        frame 14 {
          n115 = call "Verify Timer.vi"("error in (no error)"=w336, "State Machine in"=w337) -> ("error out"=w341:errorcluster, "timeout"=w335:bool, "State Machine out"=w342:refnum<class "State Machine.lvclass">)  [unwired: 7 in]
          n116 = call-dynamic "Write State Machine.vi"("error in (no error)"=w341, "State Machine.lvclass"=w342, "Device in"=w340) -> ("error out"=w338:errorcluster, "Device out"=w339:refnum<class "Channel.lvclass">)  [unwired: 7 in]
          n117 = call-dynamic "Read resp.vi"("error in (no error)"=w338, "Device in"=w339) -> ("error out"=w343:errorcluster, "resp"=w346:string, "Device out"=w344:refnum<class "Channel.lvclass">)  [unwired: 7 in]
          n118 = Equal?(x=w346, y="DONE") -> (x = y?=w333:bool)
          n119 = case shown="True" w335 {
            tunnel: [w348 w356] -> w332
            tunnel: w334 -> [w349 _]
            tunnel: w333 -> [w347 _]
            frame False {
              n120 = case shown="True" w347 {
                tunnel: [w350 w351] -> w348
                tunnel: w349 -> [w350 w352]
                frame False {
                }
                frame True {
                  n121 = disable-structure shown="Enabled" {
                    disable-tunnel: w352 -> [w354 _]
                    disable-tunnel: [w353 29 ("State")] -> w351
                    frame Disabled {
                      n122 = Increment(x=w354) -> (x+1=w353:i32)
                    }
                    frame Enabled {
                    }
                  }
                }
              }
            }
            frame True {
              n123 = disable-structure shown="Enabled" {
                disable-tunnel: [28 29] -> w356
                frame Disabled {
                  # "ERRO"
                }
                frame Enabled {
                  # "Por enquanto, prossegue\nmesmo sem receber DONE."
                }
              }
            }
          }
        }
        frame 28 {
          # "ESTADO DE ERRO: Fica aqui até que S4GUI:HandleObservationSync.vi ou S4GUI:HandleObservationAsync.vi ou os botões START, STOP, ABORT mandem para outro estado."
        }
        frame 29 {
          n124 = Unbundle By Name(w362) -> ("expose"=w364:bool)
          n125 = case shown="True" w364 {
            tunnel: [u8 0 ("State") u8 50 ("State")] -> w366
            tunnel: w365 -> [_ _]
            frame False {
            }
            frame True {
            }
          }
        }
        frame 30 {
          n126 = call-dynamic "Write Timer.vi"("error in (no error)"=w373, "Timer"=u32 50, "State Machine in"=w375) -> ("error out"=w372:errorcluster, "State Machine out"=w374:refnum<class "State Machine.lvclass">)  [unwired: 7 in]
          n127 = call-dynamic "Write State Machine.vi"("error in (no error)"=w372, "State Machine.lvclass"=w374, "Device in"=w376) -> ("error out"=w370:errorcluster, "Device out"=w371:refnum<class "Channel.lvclass">)  [unwired: 7 in]
          n128 = Unbundle By Name(w371) -> ("Interface.lvclass"=w384:refnum<class "Interface.lvclass">)
          n129 = call-dynamic "Read Cooler ON_OFF.vi"("error in (no error)"=w370, "Interface in"=w384) -> ("error out"=w369:errorcluster, "Cooler ON/OFF"=w379:i16)  [unwired: 7 in, 1 out]
          n130 = case shown="0" w379 {
            tunnel: ["1" "0"] -> w378
            frame 0 {
              (unwired) "ON"
              # "Se COOLER desligado, manda ligar."
            }
            frame 1, Default {
              (unwired) "OFF"
              # "Se COOLER ligado, manda desligar."
            }
          }
          n131 = Concatenate Strings("SET COOLER_POWER_STATUS " ("cmd"), w378) -> (w383:string)
          n132 = call-dynamic "Write cmd.vi"("error in (no error)"=w369, "cmd"=w383, "Device in"=w371) -> ("error out"=w385:errorcluster, "Device out"=w386:refnum<class "Channel.lvclass">)  [unwired: 7 in]
          n133 = Increment(x=w381) -> (x+1=w382:i32)
        }
        frame 31 {
          n134 = call "Verify Timer.vi"("error in (no error)"=w396, "State Machine in"=w393) -> ("error out"=w391:errorcluster, "timeout"=w389:bool, "State Machine out"=w392:refnum<class "State Machine.lvclass">)  [unwired: 7 in]
          n135 = call-dynamic "Write State Machine.vi"("error in (no error)"=w391, "State Machine.lvclass"=w392, "Device in"=w395) -> ("error out"=w390:errorcluster, "Device out"=w394:refnum<class "Channel.lvclass">)  [unwired: 7 in]
          n136 = call-dynamic "Read resp.vi"("error in (no error)"=w390, "Device in"=w394) -> ("error out"=w398:errorcluster, "resp"=w403:string, "Device out"=w399:refnum<class "Channel.lvclass">)  [unwired: 7 in]
          n137 = Equal?(x=w403, y="DONE") -> (x = y?=w401:bool)
          n138 = case shown="True" w389 {
            tunnel: w401 -> [w406 _]
            tunnel: [w405 w410] -> w400
            tunnel: w397 -> [w404 _]
            frame False {
              n139 = case shown="True" w406 {
                tunnel: [w407 w408] -> w405
                tunnel: w404 -> [w407 w409]
                frame False {
                }
                frame True {
                  n140 = Increment(x=w409) -> (x+1=w408:i32)
                }
              }
            }
            frame True {
              n141 = disable-structure shown="Enabled" {
                disable-tunnel: [0 ("State") 300 ("State")] -> w410
                frame Disabled {
                }
                frame Enabled {
                  (unwired) 12 ("State")
                  # "300: configura os\nparametros por comando\nSET"
                }
              }
            }
          }
        }
        frame 32 {
          n142 = call-dynamic "Write Timer.vi"("error in (no error)"=w417, "Timer"=u32 50, "State Machine in"=w418) -> ("error out"=w420:errorcluster, "State Machine out"=w415:refnum<class "State Machine.lvclass">)  [unwired: 7 in]
          n143 = call-dynamic "Write State Machine.vi"("error in (no error)"=w420, "State Machine.lvclass"=w415, "Device in"=w419) -> ("error out"=w413:errorcluster, "Device out"=w414:refnum<class "Channel.lvclass">)  [unwired: 7 in]
          n144 = call-dynamic "Write cmd.vi"("error in (no error)"=w413, "cmd"="GET COOLER_POWER_STATUS ", "Device in"=w414) -> ("error out"=w424:errorcluster, "Device out"=w425:refnum<class "Channel.lvclass">)  [unwired: 7 in]
          n145 = Increment(x=w422) -> (x+1=w423:i32)
        }
        frame 33 {
          n146 = call "Verify Timer.vi"("error in (no error)"=w429, "State Machine in"=w433) -> ("error out"=w428:errorcluster, "timeout"=w427:bool, "State Machine out"=w430:refnum<class "State Machine.lvclass">)  [unwired: 7 in]
          n147 = call-dynamic "Write State Machine.vi"("error in (no error)"=w428, "State Machine.lvclass"=w430, "Device in"=w432) -> ("error out"=w426:errorcluster, "Device out"=w431:refnum<class "Channel.lvclass">)  [unwired: 7 in]
          n148 = call-dynamic "Read resp.vi"("error in (no error)"=w426, "Device in"=w431) -> ("error out"=w438:errorcluster, "resp"=w434:string, "Device out"=w439:refnum<class "Channel.lvclass">)  [unwired: 7 in]
          n149 = case shown="True" w427 {
            tunnel: [w447 w468] -> w440
            tunnel: w439 -> [w446 w468]
            tunnel: w438 -> [w445 w467]
            tunnel: [w444 w467] -> w437
            tunnel: [w443 w466] -> w436
            tunnel: w435 -> [w442 _]
            tunnel: w434 -> [w441 _]
            frame False {
              n150 = case shown="\"0\", \"1\"" w441 {
                selector: w441 -> [_ w459]
                tunnel: [w450 w455] -> w447
                tunnel: w446 -> [w450 w463]
                tunnel: w445 -> [w449 w461]
                tunnel: [w449 w453] -> w444
                tunnel: [w448 w460] -> w443
                tunnel: w442 -> [w448 _]
                frame Default {
                }
                frame "0", "1" {
                  n151 = Decimal String To Number(string=w459) -> (number=w458:i32)  [unwired: 2 in, 1 out]
                  n152 = Unbundle By Name(w463) -> ("Interface.lvclass"=w462:refnum<class "Interface.lvclass">)
                  n153 = To Word Integer(number=w458) -> (16bit integer=w457:i16)
                  n154 = call-dynamic "Write Cooler ON_OFF.vi"("error in (no error)"=w461, "Cooler ON/OFF"=w457, "Interface in"=w462) -> ("error out"=w454:errorcluster, "Interface out"=w452:refnum<class "Interface.lvclass">)  [unwired: 7 in]
                  n155 = Bundle By Name(cluster=w463, "Interface.lvclass"=w452) -> (w456:refnum<class "Channel.lvclass">)
                  n156 = disable-structure shown="Enabled" {
                    disable-tunnel: [0 ("State") 300 ("State")] -> w460
                    frame Disabled {
                    }
                    frame Enabled {
                      (unwired) 12 ("State")
                      # "300: configura os\nparametros por comando\nSET"
                    }
                  }
                  n157 = call-dynamic "Save Temp.vi"("error in (no error)"=w454, "temp file"="lasttemp.cfg", "Channel in"=w456) -> ("error out"=w453:errorcluster, "Channel out"=w455:refnum<class "Channel.lvclass">)  [unwired: 7 in]
                }
              }
            }
            frame True {
              n158 = disable-structure shown="Enabled" {
                disable-tunnel: [0 ("State") 300 ("State")] -> w466
                frame Disabled {
                }
                frame Enabled {
                  (unwired) 12 ("State")
                  # "300: configura os\nparametros por comando\nSET"
                }
              }
            }
          }
        }
        frame 35 {
          n159 = Unbundle By Name(w479) -> ("Interface.lvclass"=w478:refnum<class "Interface.lvclass">)
          n160 = call-dynamic "Read Temperature.vi"("Interface in"=w478) -> ("Temperature"=w475:i8)  [unwired: 8 in, 2 out]
          n161 = Number To Decimal String(number=w475) -> (decimal integer string=w474:string)  [unwired: 1 in]
          n162 = Concatenate Strings("SET TEMP " ("cmd"), w474) -> (w477:string)
          n163 = call-dynamic "Write cmd.vi"("error in (no error)"=w481, "cmd"=w477, "Device in"=w479) -> ("error out"=w480:errorcluster, "Device out"=w472:refnum<class "Channel.lvclass">)  [unwired: 7 in]
          n164 = Increment(x=w471) -> (x+1=w473:i32)
        }
        frame 36 {
          n165 = call "Verify Timer.vi"("error in (no error)"=w489, "State Machine in"=w486) -> ("error out"=w484:errorcluster, "timeout"=w482:bool, "State Machine out"=w485:refnum<class "State Machine.lvclass">)  [unwired: 7 in]
          n166 = call-dynamic "Write State Machine.vi"("error in (no error)"=w484, "State Machine.lvclass"=w485, "Device in"=w488) -> ("error out"=w483:errorcluster, "Device out"=w487:refnum<class "Channel.lvclass">)  [unwired: 7 in]
          n167 = call-dynamic "Read resp.vi"("error in (no error)"=w483, "Device in"=w487) -> ("error out"=w491:errorcluster, "resp"=w496:string, "Device out"=w492:refnum<class "Channel.lvclass">)  [unwired: 7 in]
          n168 = Equal?(x=w496, y="DONE") -> (x = y?=w494:bool)
          n169 = case shown="True" w482 {
            tunnel: w494 -> [w499 _]
            tunnel: [w498 w503] -> w493
            tunnel: w490 -> [w497 _]
            frame False {
              n170 = case shown="True" w499 {
                tunnel: [w500 w501] -> w498
                tunnel: w497 -> [w500 w502]
                frame False {
                }
                frame True {
                  # "OV 2022-11-16: Ao setar a temperatura, liga \nautomaticamente o COLLER."
                  n171 = Increment(x=w502) -> (x+1=w501:i32)
                }
              }
            }
            frame True {
              n172 = disable-structure shown="Enabled" {
                disable-tunnel: [0 ("State") 300 ("State")] -> w503
                frame Disabled {
                }
                frame Enabled {
                  (unwired) 12 ("State")
                  # "300: configura os\nparametros por comando\nSET"
                }
              }
            }
          }
        }
        frame 37 {
          # "Liga COOLER"
          n173 = call-dynamic "Write Timer.vi"("error in (no error)"=w511, "Timer"=u32 50, "State Machine in"=w513) -> ("error out"=w510:errorcluster, "State Machine out"=w512:refnum<class "State Machine.lvclass">)  [unwired: 7 in]
          n174 = call-dynamic "Write State Machine.vi"("error in (no error)"=w510, "State Machine.lvclass"=w512, "Device in"=w514) -> ("error out"=w508:errorcluster, "Device out"=w507:refnum<class "Channel.lvclass">)  [unwired: 7 in]
          n175 = call-dynamic "Write cmd.vi"("error in (no error)"=w508, "cmd"="SET COOLER_POWER_STATUS 1", "Device in"=w507) -> ("error out"=w516:errorcluster, "Device out"=w517:refnum<class "Channel.lvclass">)  [unwired: 7 in]
        }
        frame 38 {
          # "ESTADO DE ERRO: Texp incompativel com a configuração do CCD;\nFica aqui até que S4GUI:HandleObservationSync.vi ou S4GUI:HandleObservationAsync.vi ou os botões START, STOP, ABORT mandem para outro estado."
        }
        frame 40 {
          n176 = disable-structure shown="Disabled" {
            disable-tunnel: [w541 w543] -> w534
            disable-tunnel: w533 -> [w539 w543]
            disable-tunnel: w531 -> [w538 w542]
            disable-tunnel: [w537 w542] -> w530
            frame Disabled {
              # "Carrega timeout de 10 ciclos\npara resposta do ACS"
              n177 = call-dynamic "Write Timer.vi"("error in (no error)"=w538, "Timer"=u32 10, "State Machine in"=w539) -> ("error out"=w537:errorcluster, "State Machine out"=w541:refnum<class "State Machine.lvclass">)  [unwired: 7 in]
            }
            frame Enabled {
            }
          }
          n178 = call-dynamic "Write State Machine.vi"("error in (no error)"=w530, "State Machine.lvclass"=w534, "Device in"=w532) -> ("error out"=w529:errorcluster, "Device out"=w526:refnum<class "Channel.lvclass">)  [unwired: 7 in]
          n179 = Unbundle By Name(w526) -> ("wait_expose"=w525:bool)
          n180 = Select(t="ON", s=w525, f="OFF") -> (s? t:f=w522:string)
          n181 = Concatenate Strings("WAIT_EXPOSE_COMMAND " ("cmd"), w522) -> (w521:string)
          n182 = call-dynamic "Write cmd.vi"("error in (no error)"=w529, "cmd"=w521, "Device in"=w526) -> ("error out"=w535:errorcluster, "Device out"=w536:refnum<class "Channel.lvclass">)  [unwired: 7 in]
        }
        frame 50 {
          n183 = Bundle By Name(cluster=w546, "stopping"=FALSE) -> (w544:refnum<class "Channel.lvclass">)
          n184 = call-dynamic "Write cmd.vi"("error in (no error)"=w552, "cmd"="EXPOSE", "Device in"=w544) -> ("error out"=w549:errorcluster, "Device out"=w550:refnum<class "Channel.lvclass">)  [unwired: 7 in]
          n185 = disable-structure shown="Enabled" {
            disable-tunnel: w555 -> [w560 w571]
            disable-tunnel: [w558 w561] -> w553
            disable-tunnel: w551 -> [_ w568]
            disable-tunnel: w550 -> [w557 w566]
            disable-tunnel: w549 -> [w556 w564]
            disable-tunnel: [w557 w565] -> w548
            disable-tunnel: [w556 w562] -> w547
            frame Disabled {
              # "OV 2023-07-05:\nVai direto para o pedido\nde STATUS (sem a pausa \nde 200ms)"
              n186 = Increment(x=w560) -> (x+1=w559:i32)
              n187 = Increment(x=w559) -> (x+1=w558:i32)
            }
            frame Enabled {
              # "Força a recarga do Ticks com\no valor do relógio do PC."
              n188 = call-dynamic "Verif Clock.vi"("error in (no error)"=w564, "period (ms)"=u32 1 ("period"), "State Machine in"=w568) -> ("error out"=w563:errorcluster, "State Machine out"=w567:refnum<class "State Machine.lvclass">)  [unwired: 6 in, 1 out]
              n189 = Increment(x=w571) -> (x+1=w570:i32)
              n190 = call-dynamic "Write State Machine.vi"("error in (no error)"=w563, "State Machine.lvclass"=w567, "Device in"=w566) -> ("error out"=w562:errorcluster, "Device out"=w565:refnum<class "Channel.lvclass">)  [unwired: 7 in]
              n191 = Increment(x=w570) -> (x+1=w561:i32)
            }
          }
        }
        frame 51 {
          # "ESTADO OPCIONAL:\nEspera estourar o timeout (200ms) antes de verificar a resposta do ACS.\nApós o timeout vai para o próximo estado enviar STATUS para confirmar\nse o ACS  foi para ACTIVE."
          n192 = call-dynamic "Verif Clock.vi"("error in (no error)"=w578, "period (ms)"=u32 200 ("period"), "State Machine in"=w582) -> ("error out"=w577:errorcluster, "State Machine out"=w581:refnum<class "State Machine.lvclass">)  [unwired: 6 in, 1 out]
          n193 = call-dynamic "Read Timeout.vi"("error in (no error)"=w577, "State Machine in"=w581) -> ("error out"=w576:errorcluster, "Timeout"=w579:bool, "State Machine out"=w580:refnum<class "State Machine.lvclass">)  [unwired: 7 in]
          n194 = call-dynamic "Write State Machine.vi"("error in (no error)"=w576, "State Machine.lvclass"=w580, "Device in"=w584) -> ("error out"=w575:errorcluster, "Device out"=w574:refnum<class "Channel.lvclass">)  [unwired: 7 in]
          n195 = case shown="True" w579 {
            tunnel: [w589 w592] -> w586
            tunnel: w585 -> [w589 w593]
            tunnel: w575 -> [w587 w590]
            tunnel: w574 -> [w588 w591]
            tunnel: [w588 w591] -> w573
            tunnel: [w587 w590] -> w572
            frame False {
            }
            frame True {
              n196 = Increment(x=w593) -> (x+1=w592:i32)
            }
          }
        }
        frame 52 {
          n197 = call-dynamic "Write cmd.vi"("error in (no error)"=w594, "cmd"="STATUS", "Device in"=w595) -> ("error out"=w599:errorcluster, "Device out"=w600:refnum<class "Channel.lvclass">)  [unwired: 7 in]
          n198 = Increment(x=w597) -> (x+1=w598:i32)
        }
        frame 53 {
          # "Status.Texp = Current frame exptime\nlastStatus = cam status (acquiring, idle, writing, reading, ...)\nStatus.Nimages = frames done\nStatus.CubesDone = ciclos realizados pelo ACS\nStatus.SequesDone = sequencias realizadas pelo ACS."
          # "Verifica timeout para ACS iniciar exposição.\nSe estourar timeout é porque o ACS não \nrecebeu o EXPOSE e então volta para 50\npara enviar novo EXPOSE."
          # "Extrair todos os parametros da respsota de STATUS e\natualizar a informação na classe Channel."
          n199 = call-dynamic "Verif Clock.vi"("error in (no error)"=w602, "period (ms)"=u32 500 ("period"), "State Machine in"=w605) -> ("error out"=w603:errorcluster, "State Machine out"=w604:refnum<class "State Machine.lvclass">)  [unwired: 6 in, 1 out]
          n200 = call-dynamic "Read Timeout.vi"("error in (no error)"=w603, "State Machine in"=w604) -> ("error out"=w618:errorcluster, "Timeout"=w606:bool, "State Machine out"=w619:refnum<class "State Machine.lvclass">)  [unwired: 7 in]
          n201 = call-dynamic "Write State Machine.vi"("error in (no error)"=w618, "State Machine.lvclass"=w619, "Device in"=w617) -> ("error out"=w615:errorcluster, "Device out"=w616:refnum<class "Channel.lvclass">)  [unwired: 7 in]
          n202 = call-dynamic "Read resp.vi"("error in (no error)"=w615, "Device in"=w616) -> ("error out"=w639:errorcluster, "resp"=w640:string, "Device out"=w643:refnum<class "Channel.lvclass">)  [unwired: 7 in]
          "resposta do STATUS" <- w640
          n203 = call-dynamic "Read Interface.vi"("error in (no error)"=w639, "Channel in"=w643) -> ("error out"=w638:errorcluster, "Interface.lvclass"=w641:refnum<class "Interface.lvclass">, "Channel out"=w642:refnum<class "Channel.lvclass">)  [unwired: 7 in]
          n204 = call-dynamic "UpdateStatus.vi"("error in (no error)"=w638, "status"=w640, "Interface in"=w641) -> ("error out"=w625:errorcluster, "Interface out"=w628:refnum<class "Interface.lvclass">)  [unwired: 7 in]
          n205 = call-dynamic "Read Exposições realizadas.vi"("error in (no error)"=w625, "Interface in"=w628) -> ("error out"=w624:errorcluster, "Exposições realizadas"=w626:dbl, "Interface out"=w627:refnum<class "Interface.lvclass">)  [unwired: 7 in]
          n206 = call-dynamic "Read Cam_Status.vi"("error in (no error)"=w624, "Interface in"=w627) -> ("error out"=w634:errorcluster, "Cam_Status"=w620:string, "Interface out"=w635:refnum<class "Interface.lvclass">)  [unwired: 7 in]
          n207 = call-dynamic "Read %Acquired.vi"("error in (no error)"=w634, "Interface in"=w635) -> ("error out"=w613:errorcluster, "% Acquired"=w631:dbl, "Interface out"=w614:refnum<class "Interface.lvclass">)  [unwired: 7 in]
          n208 = call-dynamic "Read Number of Cycles.vi"("error in (no error)"=w613, "Interface in"=w614) -> ("error out"=w609:errorcluster, "Number of Cycles"=w612:u32, "Interface out"=w611:refnum<class "Interface.lvclass">)  [unwired: 7 in]
          n209 = call-dynamic "Read Number of Sequences.vi"("error in (no error)"=w609, "Interface in"=w611) -> ("error out"=w608:errorcluster, "Number of Sequences"=w607:u32, "Interface out"=w610:refnum<class "Interface.lvclass">)  [unwired: 7 in]
          n210 = call "Read Exposure Time.vi"("error in (no error)"=w608, "Interface in"=w610) -> ("error out"=w622:errorcluster, "Exposure Time"=w633:dbl, "Interface out"=w621:refnum<class "Interface.lvclass">)  [unwired: 7 in]
          n211 = call-dynamic "Write Interface.vi"("error in (no error)"=w622, "Interface.lvclass"=w621, "Channel in"=w642) -> ("error out"=w637:errorcluster, "Channel out"=w636:refnum<class "Channel.lvclass">)  [unwired: 7 in]
          n212 = case shown="\"ACTIVE\"" w620 {
            tunnel: [w647 w650] -> w646
            tunnel: w645 -> [w648 w651]
            tunnel: w606 -> [_ w649]
            frame "ACTIVE" {
              n213 = Increment(x=w648) -> (x+1=w647:i32)
            }
            frame Default {
              n214 = case shown="True" w649 {
                tunnel: w651 -> [w652 _]
                tunnel: [w652 0] -> w650
                frame False {
                }
                frame True {
                }
              }
            }
          }
          n215 = To Unsigned Long Integer(number=w626) -> (unsigned 32bit integer=w623:u32)
          n216 = Divide(x=w631, y=100.0) -> (x/y=w629:dbl)
          n217 = Multiply(x=w633, y=w629) -> (x*y=w632:dbl)
          n218 = Bundle By Name(cluster=w636, "Texp"=w632, "lastStatus"=w620, "Nimages"=w623, "CyclesDone"=w612, "SequesDone"=w607) -> (w644:refnum<class "Channel.lvclass">)
        }
        frame 54 {
          # "Verifica o timeout de 5s para enviar\ntelemetria para o ACS."
          n219 = call-dynamic "Verif Clock 2.vi"("error in (no error)"=w662, "period (ms)"=u32 5000 ("period"), "State Machine in"=w663) -> ("error out"=w660:errorcluster, "State Machine out"=w661:refnum<class "State Machine.lvclass">)  [unwired: 6 in, 1 out]
          n220 = call-dynamic "Read Timeout 2.vi"("error in (no error)"=w660, "State Machine in"=w661) -> ("error out"=w656:errorcluster, "Timeout 2"=w659:bool, "State Machine out"=w657:refnum<class "State Machine.lvclass">)  [unwired: 7 in]
          n221 = call-dynamic "Write State Machine.vi"("error in (no error)"=w656, "State Machine.lvclass"=w657, "Device in"=w658) -> ("error out"=w655:errorcluster, "Device out"=w654:refnum<class "Channel.lvclass">)  [unwired: 7 in]
          n222 = case shown="True" w659 {
            tunnel: [w675 w676] -> w668
            tunnel: [w674 w677] -> w667
            tunnel: [w673 59] -> w666
            tunnel: w665 -> [w672 _]
            tunnel: w654 -> [w670 w676]
            tunnel: w655 -> [w669 w677]
            frame False {
              n223 = call-dynamic "Write cmd.vi"("error in (no error)"=w669, "cmd"="STATUS", "Device in"=w670) -> ("error out"=w674:errorcluster, "Device out"=w675:refnum<class "Channel.lvclass">)  [unwired: 7 in]
              n224 = Increment(x=w672) -> (x+1=w673:i32)
            }
            frame True {
              # "Estourou timeout de 5s:\nDesvia para enviar dados de \nTELEMETRIA a cada 5s (estado 59)"
            }
          }
        }
        frame 55 {
          # "Status.Texp = Current frame exptime\nlastStatus = cam status (acquiring, idle, writing, reading, ...)\nStatus.Nimages = frames done\nStatus.CubesDone = ciclos realizados pelo ACS\nStatus.SequesDone = sequencias realizadas pelo ACS."
          # "Extrair todos os parametros da respsota de STATUS e\natualizar a informação na classe Channel."
          n225 = call-dynamic "Verif Clock.vi"("error in (no error)"=w682, "period (ms)"=u32 500 ("period"), "State Machine in"=w685) -> ("error out"=w681:errorcluster, "State Machine out"=w684:refnum<class "State Machine.lvclass">)  [unwired: 6 in, 1 out]
          n226 = call-dynamic "Read Timeout.vi"("error in (no error)"=w681, "State Machine in"=w684) -> ("error out"=w679:errorcluster, "Timeout"=w680:bool, "State Machine out"=w683:refnum<class "State Machine.lvclass">)  [unwired: 7 in]
          n227 = call-dynamic "Read resp.vi"("error in (no error)"=w679, "Device in"=w695) -> ("error out"=w717:errorcluster, "resp"=w718:string, "Device out"=w721:refnum<class "Channel.lvclass">)  [unwired: 7 in]
          n228 = call-dynamic "Read Interface.vi"("error in (no error)"=w717, "Channel in"=w721) -> ("error out"=w716:errorcluster, "Interface.lvclass"=w719:refnum<class "Interface.lvclass">, "Channel out"=w720:refnum<class "Channel.lvclass">)  [unwired: 7 in]
          n229 = call-dynamic "UpdateStatus.vi"("error in (no error)"=w716, "status"=w718, "Interface in"=w719) -> ("error out"=w703:errorcluster, "Interface out"=w706:refnum<class "Interface.lvclass">)  [unwired: 7 in]
          n230 = call-dynamic "Read Exposições realizadas.vi"("error in (no error)"=w703, "Interface in"=w706) -> ("error out"=w702:errorcluster, "Exposições realizadas"=w704:dbl, "Interface out"=w705:refnum<class "Interface.lvclass">)  [unwired: 7 in]
          n231 = call-dynamic "Read Cam_Status.vi"("error in (no error)"=w702, "Interface in"=w705) -> ("error out"=w713:errorcluster, "Cam_Status"=w700:string, "Interface out"=w715:refnum<class "Interface.lvclass">)  [unwired: 7 in]
          n232 = call-dynamic "Read %Acquired.vi"("error in (no error)"=w713, "Interface in"=w715) -> ("error out"=w712:errorcluster, "% Acquired"=w709:dbl, "Interface out"=w714:refnum<class "Interface.lvclass">)  [unwired: 7 in]
          n233 = call "Read Exposure Time.vi"("error in (no error)"=w712, "Interface in"=w714) -> ("error out"=w693:errorcluster, "Exposure Time"=w711:dbl, "Interface out"=w694:refnum<class "Interface.lvclass">)  [unwired: 7 in]
          n234 = call-dynamic "Read Number of Cycles.vi"("error in (no error)"=w693, "Interface in"=w694) -> ("error out"=w690:errorcluster, "Number of Cycles"=w692:u32, "Interface out"=w691:refnum<class "Interface.lvclass">)  [unwired: 7 in]
          n235 = call-dynamic "Read Number of Sequences.vi"("error in (no error)"=w690, "Interface in"=w691) -> ("error out"=w689:errorcluster, "Number of Sequences"=w687:u32, "Interface out"=w688:refnum<class "Interface.lvclass">)  [unwired: 7 in]
          n236 = call-dynamic "Write Interface.vi"("error in (no error)"=w689, "Interface.lvclass"=w688, "Channel in"=w720) -> ("error out"=w699:errorcluster, "Channel out"=w698:refnum<class "Channel.lvclass">)  [unwired: 7 in]
          n237 = case shown="\"ACQUISITION ABORTED\", \"IDLE\"" w700 {
            tunnel: [w733 w741 w748 w762] -> w724
            tunnel: w723 -> [_ w741 w749 w763]
            tunnel: w699 -> [w731 w737 w744 w760]
            tunnel: [w728 w739 w746 w757] -> w697
            tunnel: w698 -> [w729 w740 w747 w761]
            tunnel: [w725 w736 w743 w754] -> w696
            tunnel: w683 -> [w732 w738 w745 w759]
            tunnel: w680 -> [_ _ w742 w753]
            frame "ACQUISITION ABORTED", "IDLE" {
              # "250x20ms=5s"
              n238 = call-dynamic "Write Timer.vi"("error in (no error)"=w731, "Timer"=u32 250, "State Machine in"=w732) -> ("error out"=w726:errorcluster, "State Machine out"=w727:refnum<class "State Machine.lvclass">)  [unwired: 7 in]
              n239 = call-dynamic "Write State Machine.vi"("error in (no error)"=w726, "State Machine.lvclass"=w727, "Device in"=w729) -> ("error out"=w725:errorcluster, "Device out"=w728:refnum<class "Channel.lvclass">)  [unwired: 7 in]
              n240 = disable-structure shown="Enabled" {
                disable-tunnel: [32 ("State") 0 ("State")] -> w733
                frame Disabled {
                }
                frame Enabled {
                  # "OVJ 20230704"
                }
              }
            }
            frame Default {
              # "STATUS DETECTOR = desconhecido"
              n241 = call-dynamic "Write State Machine.vi"("error in (no error)"=w737, "State Machine.lvclass"=w738, "Device in"=w740) -> ("error out"=w736:errorcluster, "Device out"=w739:refnum<class "Channel.lvclass">)  [unwired: 7 in]
            }
            frame "ACTIVE", "WAITING EXPOSE COMMAND" {
              # "STATUS DETECTOR = ACTIVE or WAITING EXPOSE COMMAND"
              n242 = case shown="True" w742 {
                tunnel: w749 -> [w750 w752]
                tunnel: [w750 w751] -> w748
                frame False {
                }
                frame True {
                  n243 = Decrement(x=w752) -> (x-1=w751:i32)
                }
              }
              n244 = call-dynamic "Write State Machine.vi"("error in (no error)"=w744, "State Machine.lvclass"=w745, "Device in"=w747) -> ("error out"=w743:errorcluster, "Device out"=w746:refnum<class "Channel.lvclass">)  [unwired: 7 in]
            }
            frame "" {
              # "STATUS=\"\"\nACS parado"
              n245 = case shown="True" w753 {
                tunnel: w763 -> [w764 _]
                tunnel: [w764 0] -> w762
                tunnel: w761 -> [w767 w770]
                tunnel: [w767 w770] -> w758
                tunnel: w760 -> [w766 w771]
                tunnel: [w766 w768] -> w755
                tunnel: w759 -> [w765 w773]
                tunnel: [w765 w769] -> w756
                frame False {
                }
                frame True {
                  n246 = call-dynamic "Write Timer.vi"("error in (no error)"=w771, "Timer"=u32 250, "State Machine in"=w773) -> ("error out"=w768:errorcluster, "State Machine out"=w769:refnum<class "State Machine.lvclass">)  [unwired: 7 in]
                }
              }
              n247 = call-dynamic "Write State Machine.vi"("error in (no error)"=w755, "State Machine.lvclass"=w756, "Device in"=w758) -> ("error out"=w754:errorcluster, "Device out"=w757:refnum<class "Channel.lvclass">)  [unwired: 7 in]
            }
          }
          n248 = To Unsigned Long Integer(number=w704) -> (unsigned 32bit integer=w701:u32)
          n249 = Divide(x=w709, y=100.0) -> (x/y=w707:dbl)
          n250 = Multiply(x=w711, y=w707) -> (x*y=w710:dbl)
          n251 = Bundle By Name(cluster=w697, "Texp"=w710, "lastStatus"=w700, "Nimages"=w701, "CyclesDone"=w692, "SequesDone"=w687) -> (w722:refnum<class "Channel.lvclass">)
        }
        frame 56 {
          # "Pedido de STATUS para verificar conexão com ACS"
          # "Carrega timeout de 10 ciclos \n(20 x 20ms = 0.4s) \npara resposta do ACS"
          n252 = call-dynamic "Write Timer.vi"("error in (no error)"=w781, "Timer"=u32 20, "State Machine in"=w785) -> ("error out"=w786:errorcluster, "State Machine out"=w787:refnum<class "State Machine.lvclass">)  [unwired: 7 in]
          n253 = call-dynamic "Write State Machine.vi"("error in (no error)"=w786, "State Machine.lvclass"=w787, "Device in"=w783) -> ("error out"=w780:errorcluster, "Device out"=w782:refnum<class "Channel.lvclass">)  [unwired: 7 in]
          n254 = call-dynamic "Write cmd.vi"("error in (no error)"=w780, "cmd"="STATUS", "Device in"=w782) -> ("error out"=w778:errorcluster, "Device out"=w779:refnum<class "Channel.lvclass">)  [unwired: 7 in]
          n255 = Increment(x=w789) -> (x+1=w790:i32)
          n256 = call "Write connected.vi"("error in (no error)"=w778, "connected"=FALSE, "Device in"=w779) -> ("error out"=w776:errorcluster, "Device out"=w777:refnum<class "Channel.lvclass">)  [unwired: 7 in]
        }
        frame 57 {
          # "Status.Texp = Current frame exptime\nlastStatus = cam status (acquiring, idle, writing, reading, ...)\nStatus.Nimages = frames done\nStatus.CubesDone = ciclos realizados pelo ACS\nStatus.SequesDone = sequencias realizadas pelo ACS."
          # "Extrair todos os parametros da respsota de STATUS e\natualizar a informação na classe Channel."
          n257 = call "Verify Timer.vi"("error in (no error)"=w809, "State Machine in"=w808) -> ("error out"=w805:errorcluster, "State Machine out"=w807:refnum<class "State Machine.lvclass">)  [unwired: 7 in, 1 out]
          n258 = call-dynamic "Read Timeout.vi"("error in (no error)"=w805, "State Machine in"=w807) -> ("error out"=w800:errorcluster, "Timeout"=w804:bool, "State Machine out"=w806:refnum<class "State Machine.lvclass">)  [unwired: 7 in]
          n259 = call "Read connected.vi"("error in (no error)"=w800, "Device in"=w803) -> ("error out"=w801:errorcluster, "connected"=w799:bool, "Device out"=w802:refnum<class "Channel.lvclass">)  [unwired: 7 in]
          n260 = call-dynamic "Read resp.vi"("error in (no error)"=w801, "Device in"=w802) -> ("error out"=w831:errorcluster, "resp"=w832:string, "Device out"=w835:refnum<class "Channel.lvclass">)  [unwired: 7 in]
          n261 = call-dynamic "Read Interface.vi"("error in (no error)"=w831, "Channel in"=w835) -> ("error out"=w830:errorcluster, "Interface.lvclass"=w833:refnum<class "Interface.lvclass">, "Channel out"=w834:refnum<class "Channel.lvclass">)  [unwired: 7 in]
          n262 = call-dynamic "UpdateStatus.vi"("error in (no error)"=w830, "status"=w832, "Interface in"=w833) -> ("error out"=w817:errorcluster, "Interface out"=w820:refnum<class "Interface.lvclass">)  [unwired: 7 in]
          n263 = call-dynamic "Read Exposições realizadas.vi"("error in (no error)"=w817, "Interface in"=w820) -> ("error out"=w816:errorcluster, "Exposições realizadas"=w818:dbl, "Interface out"=w819:refnum<class "Interface.lvclass">)  [unwired: 7 in]
          n264 = call-dynamic "Read Cam_Status.vi"("error in (no error)"=w816, "Interface in"=w819) -> ("error out"=w827:errorcluster, "Cam_Status"=w814:string, "Interface out"=w829:refnum<class "Interface.lvclass">)  [unwired: 7 in]
          n265 = call-dynamic "Read %Acquired.vi"("error in (no error)"=w827, "Interface in"=w829) -> ("error out"=w826:errorcluster, "% Acquired"=w823:dbl, "Interface out"=w828:refnum<class "Interface.lvclass">)  [unwired: 7 in]
          n266 = call "Read Exposure Time.vi"("error in (no error)"=w826, "Interface in"=w828) -> ("error out"=w797:errorcluster, "Exposure Time"=w825:dbl, "Interface out"=w798:refnum<class "Interface.lvclass">)  [unwired: 7 in]
          n267 = call-dynamic "Read Number of Cycles.vi"("error in (no error)"=w797, "Interface in"=w798) -> ("error out"=w793:errorcluster, "Number of Cycles"=w796:u32, "Interface out"=w795:refnum<class "Interface.lvclass">)  [unwired: 7 in]
          n268 = call-dynamic "Read Number of Sequences.vi"("error in (no error)"=w793, "Interface in"=w795) -> ("error out"=w792:errorcluster, "Number of Sequences"=w791:u32, "Interface out"=w794:refnum<class "Interface.lvclass">)  [unwired: 7 in]
          n269 = call-dynamic "Write Interface.vi"("error in (no error)"=w792, "Interface.lvclass"=w794, "Channel in"=w834) -> ("error out"=w813:errorcluster, "Channel out"=w812:refnum<class "Channel.lvclass">)  [unwired: 7 in]
          n270 = case shown="False" w799 {
            tunnel: [w841 w858] -> w838
            tunnel: w837 -> [w842 w859]
            tunnel: w813 -> [w839 w856]
            tunnel: [w844 w853] -> w811
            tunnel: w812 -> [w845 w857]
            tunnel: [w843 w850] -> w810
            tunnel: w806 -> [w840 w855]
            tunnel: w804 -> [_ w849]
            frame True {
              # "Conneted=T\nACS respondeu"
              n271 = disable-structure shown="Enabled" {
                disable-tunnel: w842 -> [w847 _]
                disable-tunnel: [w846 0] -> w841
                frame Disabled {
                  n272 = Increment(x=w847) -> (x+1=w846:i32)
                }
                frame Enabled {
                }
              }
              n273 = call-dynamic "Write State Machine.vi"("error in (no error)"=w839, "State Machine.lvclass"=w840, "Device in"=w845) -> ("error out"=w843:errorcluster, "Device out"=w844:refnum<class "Channel.lvclass">)  [unwired: 7 in]
            }
            frame False {
              # "Conneted=F\nACS não resp."
              n274 = case shown="True" w849 {
                tunnel: w859 -> [w860 _]
                tunnel: [w860 0] -> w858
                tunnel: w857 -> [w863 w866]
                tunnel: [w863 w866] -> w854
                tunnel: w856 -> [w862 w867]
                tunnel: [w862 w864] -> w851
                tunnel: w855 -> [w861 w869]
                tunnel: [w861 w865] -> w852
                frame False {
                }
                frame True {
                  n275 = call-dynamic "Write Timer.vi"("error in (no error)"=w867, "Timer"=u32 250, "State Machine in"=w869) -> ("error out"=w864:errorcluster, "State Machine out"=w865:refnum<class "State Machine.lvclass">)  [unwired: 7 in]
                }
              }
              n276 = call-dynamic "Write State Machine.vi"("error in (no error)"=w851, "State Machine.lvclass"=w852, "Device in"=w854) -> ("error out"=w850:errorcluster, "Device out"=w853:refnum<class "Channel.lvclass">)  [unwired: 7 in]
            }
          }
          n277 = Divide(x=w823, y=100.0) -> (x/y=w821:dbl)
          n278 = To Unsigned Long Integer(number=w818) -> (unsigned 32bit integer=w815:u32)
          n279 = Multiply(x=w825, y=w821) -> (x*y=w824:dbl)
          n280 = Bundle By Name(cluster=w811, "Texp"=w824, "lastStatus"=w814, "Nimages"=w815, "CyclesDone"=w796, "SequesDone"=w791) -> (w836:refnum<class "Channel.lvclass">)
        }
        frame 58 {
          w875 = "}" ("regular expression")
          # "Passa valores da telemetria adquiridos do TCS"
          n281 = call-dynamic "Write State Machine.vi"("error in (no error)"=w871, "State Machine.lvclass"=w872, "Device in"=w882) -> ("error out"=w879:errorcluster, "Device out"=w881:refnum<class "Channel.lvclass">)  [unwired: 7 in]
          n282 = Unbundle By Name(w881) -> ("TCS telemetry"=w876:string, "Filter"=w878:u8)
          n283 = Match Pattern(string=w876, regular expression=w875) -> (before substring=w874:string, match substring=w873:string)  [unwired: 1 in, 2 out]
          n284 = Equal?(x=w873, y=w875) -> (x = y?=w877:bool)
          n285 = case shown="True" w877 {
            tunnel: [w886 w896] -> w884
            tunnel: [w885 w895] -> w883
            tunnel: w881 -> [w886 w894]
            tunnel: w879 -> [w885 w891]
            tunnel: w878 -> [_ w890]
            tunnel: w874 -> [_ w889]
            tunnel: w873 -> [_ w888]
            frame False {
            }
            frame True {
              (unwired) "\"CTRLINTE\":\"S4GUI\"}" ("string")
              (unwired) "\"FILTER\":\"" ("string")
              n286 = case shown="5" w890 {
                tunnel: ["CLEAR\"," ("string") "U\"," ("string") "B\"," ("string") "V\"," ("string") "R\"," ("string") "S\"," ("string")] -> _
                frame 0, Default {
                }
                frame 1 {
                }
                frame 2 {
                }
                frame 3 {
                }
                frame 4 {
                }
                frame 5 {
                }
              }
              n287 = Concatenate Strings(w889, w888) -> (w887:string)
              n288 = Concatenate Strings("WRITE_HEADER_DATA " ("cmd"), w887) -> (w892:string)
              n289 = call-dynamic "Write cmd.vi"("error in (no error)"=w891, "cmd"=w892, "Device in"=w894) -> ("error out"=w895:errorcluster, "Device out"=w896:refnum<class "Channel.lvclass">)  [unwired: 7 in]
            }
          }
        }
        frame 59 {
          w907 = "}" ("regular expression")
          # "Passa valores da telemetria adquiridos do TCS durante a aquisição do canal (estados 54 e 55)"
          n290 = call-dynamic "Write State Machine.vi"("error in (no error)"=w903, "State Machine.lvclass"=w904, "Device in"=w913) -> ("error out"=w910:errorcluster, "Device out"=w912:refnum<class "Channel.lvclass">)  [unwired: 7 in]
          n291 = Unbundle By Name(w912) -> ("TCS telemetry"=w908:string)
          n292 = Match Pattern(string=w908, regular expression=w907) -> (before substring=w906:string, match substring=w905:string)  [unwired: 1 in, 2 out]
          n293 = Equal?(x=w905, y=w907) -> (x = y?=w909:bool)
          n294 = case shown="True" w909 {
            tunnel: [w917 w926] -> w915
            tunnel: [w916 w925] -> w914
            tunnel: w912 -> [w917 w924]
            tunnel: w910 -> [w916 w921]
            tunnel: w906 -> [_ w920]
            tunnel: w905 -> [_ w919]
            frame False {
            }
            frame True {
              n295 = Concatenate Strings(w920, w919) -> (w918:string)
              n296 = Concatenate Strings("WRITE_HEADER_DATA " ("cmd"), w918) -> (w922:string)
              n297 = call-dynamic "Write cmd.vi"("error in (no error)"=w921, "cmd"=w922, "Device in"=w924) -> ("error out"=w925:errorcluster, "Device out"=w926:refnum<class "Channel.lvclass">)  [unwired: 7 in]
            }
          }
        }
        frame 60 {
          # "Carrega timeout de 5 ciclos\npara resposta do ACS"
          n298 = call-dynamic "Write Timer.vi"("Timer"=u32 5, "State Machine in"=w932) -> ("error out"=w933:errorcluster, "State Machine out"=w931:refnum<class "State Machine.lvclass">)  [unwired: 8 in]
          n299 = call-dynamic "Write State Machine.vi"("error in (no error)"=w933, "State Machine.lvclass"=w931, "Device in"=w930) -> ("Device out"=w929:refnum<class "Channel.lvclass">)  [unwired: 7 in, 1 out]
          n300 = disable-structure shown="Enabled" {
            disable-tunnel: [w944 w946] -> w937
            disable-tunnel: w936 -> [w943 w945]
            disable-tunnel: [w942 w945] -> w935
            disable-tunnel: w929 -> [w940 w946]
            disable-tunnel: w928 -> [w939 _]
            disable-tunnel: [w938 62] -> w927
            frame Disabled {
              n301 = Increment(x=w939) -> (x+1=w938:i32)
              n302 = call-dynamic "Write cmd.vi"("error in (no error)"=w943, "cmd"="INIT", "Device in"=w940) -> ("error out"=w942:errorcluster, "Device out"=w944:refnum<class "Channel.lvclass">)  [unwired: 7 in]
            }
            frame Enabled {
            }
          }
        }
        frame 61 {
          w957 = "INITIALIZATION"
          # "Verifica timeout para ACS responder.\nSe estourar timeout é porque o ACS não \nrespondeu e este canal volta para o estado 0\npara não \"travar\" os outros canais no \nS4ACS_GUI:HandleObservation.vi."
          n303 = call "Verify Timer.vi"("error in (no error)"=w948, "State Machine in"=w953) -> ("error out"=w954:errorcluster, "timeout"=w949:bool, "State Machine out"=w955:refnum<class "State Machine.lvclass">)  [unwired: 7 in]
          n304 = call-dynamic "Write State Machine.vi"("error in (no error)"=w954, "State Machine.lvclass"=w955, "Device in"=w952) -> ("error out"=w950:errorcluster, "Device out"=w951:refnum<class "Channel.lvclass">)  [unwired: 7 in]
          n305 = call-dynamic "Read resp.vi"("error in (no error)"=w950, "Device in"=w951) -> ("error out"=w961:errorcluster, "resp"=w959:string, "Device out"=w962:refnum<class "Channel.lvclass">)  [unwired: 7 in]
          "resp INIT" <- w959
          n306 = Match Pattern(string=w959, regular expression=w957) -> (match substring=w958:string)  [unwired: 1 in, 3 out]
          n307 = Equal?(x=w958, y=w957) -> (x = y?=w956:bool)
          n308 = case shown="True" w956 {
            tunnel: [w964 w969] -> w963
            tunnel: w960 -> [w965 w970]
            tunnel: w949 -> [w966 _]
            frame False {
              n309 = case shown="False" w966 {
                tunnel: [w967 0 ("State")] -> w964
                tunnel: w965 -> [w967 _]
                frame False {
                }
                frame True {
                }
              }
            }
            frame True {
              n310 = disable-structure shown="Enabled" {
                disable-tunnel: w970 -> [w972 _]
                disable-tunnel: [w971 54] -> w969
                frame Disabled {
                  n311 = Increment(x=w972) -> (x+1=w971:i32)
                }
                frame Enabled {
                  # "debug:\nNão deve enviar\n WRITE_SETUP para o \nACS antigo"
                }
              }
            }
          }
        }
        frame 62 {
          # "Carrega timeout de 50 ciclos\npara resposta do ACS"
          n312 = call-dynamic "Write Timer.vi"("error in (no error)"=w983, "Timer"=u32 50, "State Machine in"=w986) -> ("error out"=w987:errorcluster, "State Machine out"=w985:refnum<class "State Machine.lvclass">)  [unwired: 7 in]
          n313 = call-dynamic "Write State Machine.vi"("error in (no error)"=w987, "State Machine.lvclass"=w985, "Device in"=w984) -> ("error out"=w980:errorcluster, "Device out"=w982:refnum<class "Channel.lvclass">)  [unwired: 7 in]
          n314 = Unbundle By Name(w982) -> ("Interface.lvclass"=w981:refnum<class "Interface.lvclass">)
          n315 = call-dynamic "Get CCD_Config.vi"("error in (no error)"=w980, "Interface in"=w981) -> ("error out"=w975:errorcluster, "output cluster"=w977:T2)  [unwired: 7 in, 1 out]
          n316 = Flatten To JSON(anything=w977, error in (no error)=w975) -> (JSON string=w976:string, 11:w974:errorcluster)  [unwired: 1 in]
          n317 = Concatenate Strings("WRITE_SETUP " ("cmd"), w976) -> (w978:string)
          n318 = call-dynamic "Write cmd.vi"("error in (no error)"=w974, "cmd"=w978, "Device in"=w982) -> ("error out"=w991:errorcluster, "Device out"=w992:refnum<class "Channel.lvclass">)  [unwired: 7 in]
          n319 = Increment(x=w989) -> (x+1=w990:i32)
        }
        frame 63 {
          # "Não há resposta para o comando WRTITE_SETUP\nQuando estourar timeout vai para o estado 64 para \nobter o STATUS do ACS."
          n320 = call "Verify Timer.vi"("error in (no error)"=w996, "State Machine in"=w998) -> ("error out"=w999:errorcluster, "timeout"=w995:bool, "State Machine out"=w1000:refnum<class "State Machine.lvclass">)  [unwired: 7 in]
          n321 = call-dynamic "Write State Machine.vi"("error in (no error)"=w999, "State Machine.lvclass"=w1000, "Device in"=w997) -> ("error out"=w993:errorcluster, "Device out"=w994:refnum<class "Channel.lvclass">)  [unwired: 7 in]
          n322 = case shown="True" w995 {
            tunnel: [w1003 w1004] -> w1002
            tunnel: w1001 -> [w1003 w1005]
            frame False {
            }
            frame True {
              n323 = Increment(x=w1005) -> (x+1=w1004:i32)
            }
          }
        }
        frame 64 {
          # "Carrega timeout de 50 ciclos\npara resposta do ACS"
          n324 = call-dynamic "Write Timer.vi"("error in (no error)"=w1009, "Timer"=u32 50, "State Machine in"=w1012) -> ("error out"=w1013:errorcluster, "State Machine out"=w1011:refnum<class "State Machine.lvclass">)  [unwired: 7 in]
          n325 = call-dynamic "Write State Machine.vi"("error in (no error)"=w1013, "State Machine.lvclass"=w1011, "Device in"=w1010) -> ("error out"=w1006:errorcluster, "Device out"=w1008:refnum<class "Channel.lvclass">)  [unwired: 7 in]
          n326 = call-dynamic "Write cmd.vi"("error in (no error)"=w1006, "cmd"="READ_SETUP ", "Device in"=w1008) -> ("error out"=w1017:errorcluster, "Device out"=w1018:refnum<class "Channel.lvclass">)  [unwired: 7 in]
          n327 = Increment(x=w1015) -> (x+1=w1016:i32)
        }
        frame 65 {
          n328 = call "Verify Timer.vi"("error in (no error)"=w1037, "State Machine in"=w1039) -> ("error out"=w1040:errorcluster, "timeout"=w1023:bool, "State Machine out"=w1041:refnum<class "State Machine.lvclass">)  [unwired: 7 in]
          n329 = call-dynamic "Write State Machine.vi"("error in (no error)"=w1040, "State Machine.lvclass"=w1041, "Device in"=w1038) -> ("error out"=w1035:errorcluster, "Device out"=w1036:refnum<class "Channel.lvclass">)  [unwired: 7 in]
          n330 = call-dynamic "Read resp.vi"("error in (no error)"=w1035, "Device in"=w1036) -> ("error out"=w1029:errorcluster, "resp"=w1027:string, "Device out"=w1034:refnum<class "Channel.lvclass">)  [unwired: 7 in]
          n331 = Unbundle By Name(w1034) -> ("Interface.lvclass"=w1030:refnum<class "Interface.lvclass">)
          n332 = call-dynamic "Get CCD_Config.vi"("error in (no error)"=w1029, "Interface in"=w1030) -> ("error out"=w1031:errorcluster, "output cluster"=w1028:T2, "Interface out"=w1032:refnum<class "Interface.lvclass">)  [unwired: 7 in]
          n333 = case shown="True" w1023 {
            tunnel: w1032 -> [w1044 w1055]
            tunnel: w1031 -> [w1043 w1054]
            tunnel: w1028 -> [_ w1057]
            tunnel: w1027 -> [_ w1048]
            tunnel: [w1044 w1053] -> w1025
            tunnel: [w1043 w1052] -> w1026
            tunnel: [T1 {"ACQUISITION_MODE"=FALSE, "TRIGGER_MODE"=FALSE, "READ_MODE"=FALSE, "PREAMP"=FALSE, "READOUT_RATE"=FALSE, "VERTICAL_SHIFT_SPEED"=FALSE, "EM_MODE"=FALSE, "EM_GAIN"=FALSE, "SHUTTER_MODE"=FALSE, "SHUTTER_TTL"=FALSE, "SHUTTER_OPENING_TIME"=FALSE, "SHUTTER_CLOSING_TIME"=FALSE, "VBIN"=FALSE, "HBIN"=FALSE, "INITIAL_LINE"=FALSE, "INITIAL_COLUMN"=FALSE, "FINAL_LINE"=FALSE, "FINAL_COLUMN"=FALSE, "FRAME_TRANSFER"=FALSE, "VERTICAL_CLOCK_VOLTAGE"=FALSE, "AD_CHANNEL"=FALSE} ("x = y?") w1056] -> w1024
            tunnel: w1020 -> [w1042 w1047]
            tunnel: [w1042 w1046] -> w1019
            frame False {
            }
            frame True {
              w1049 = "\"HBIN\"" ("regular expression")
              n334 = Match Pattern(string=w1048, regular expression=w1049) -> (match substring=w1050:string)  [unwired: 1 in, 3 out]
              n335 = Equal?(x=w1049, y=w1050) -> (x = y?=w1051:bool)
              n336 = case shown="True" w1051 {
                tunnel: w1057 -> [_ w1069]
                tunnel: [T1 {"ACQUISITION_MODE"=FALSE, "TRIGGER_MODE"=FALSE, "READ_MODE"=FALSE, "PREAMP"=FALSE, "READOUT_RATE"=FALSE, "VERTICAL_SHIFT_SPEED"=FALSE, "EM_MODE"=FALSE, "EM_GAIN"=FALSE, "SHUTTER_MODE"=FALSE, "SHUTTER_TTL"=FALSE, "SHUTTER_OPENING_TIME"=FALSE, "SHUTTER_CLOSING_TIME"=FALSE, "VBIN"=FALSE, "HBIN"=FALSE, "INITIAL_LINE"=FALSE, "INITIAL_COLUMN"=FALSE, "FINAL_LINE"=FALSE, "FINAL_COLUMN"=FALSE, "FRAME_TRANSFER"=FALSE, "VERTICAL_CLOCK_VOLTAGE"=FALSE, "AD_CHANNEL"=FALSE} ("x = y?") w1068] -> w1056
                tunnel: w1055 -> [w1060 w1067]
                tunnel: w1054 -> [w1059 w1066]
                tunnel: [w1060 w1065] -> w1053
                tunnel: [w1059 w1064] -> w1052
                tunnel: w1048 -> [_ w1061]
                frame False {
                }
                frame True {
                  n337 = Unflatten From JSON(JSON string=w1061, type and defaults=w1069) -> (value=w1063:T2, error out=→"error out 2":errorcluster)  [unwired: 5 in]
                  n338 = call-dynamic "Set CCD_Config.vi"("error in (no error)"=w1066, "input cluster"=w1063, "Interface in"=w1067) -> ("error out"=w1064:errorcluster, "Interface out"=w1065:refnum<class "Interface.lvclass">)  [unwired: 7 in]
                  n339 = Equal?(x=w1063, y=w1069) -> (x = y?=w1068:T1)
                }
              }
              n340 = Increment(x=w1047) -> (x+1=w1046:i32)
            }
          }
          "x = y?" <- w1024
          n341 = call "Write Checked Params.vi"("error in (no error)"=w1026, "Checked Params"=w1024, "Interface in"=w1025) -> ("error out"=w1021:errorcluster, "Interface out"=w1022:refnum<class "Interface.lvclass">)  [unwired: 7 in]
          n342 = Bundle By Name(cluster=w1034, "Interface.lvclass"=w1022) -> (w1033:refnum<class "Channel.lvclass">)
        }
        frame 66 {
          # "O valor do COOLER aqui\nfoi carregado no Acquistion:Init.vi"
          # "Se COOLER=0\n        SET COLLERPOWER_STATUS 0\n        AVANÇA ESTADO\n        VAI PRA 0\nSe COOLER=1:\n      DESVIA PARA Estado 35"
          # "Carrega timeout de 50 ciclos\npara resposta do ACS"
          n343 = call-dynamic "Write Timer.vi"("error in (no error)"=w1077, "Timer"=u32 50, "State Machine in"=w1078) -> ("error out"=w1075:errorcluster, "State Machine out"=w1074:refnum<class "State Machine.lvclass">)  [unwired: 7 in]
          n344 = call-dynamic "Write State Machine.vi"("error in (no error)"=w1075, "State Machine.lvclass"=w1074, "Device in"=w1076) -> ("error out"=w1073:errorcluster, "Device out"=w1072:refnum<class "Channel.lvclass">)  [unwired: 7 in]
          n345 = Unbundle By Name(w1072) -> ("Interface.lvclass"=w1071:refnum<class "Interface.lvclass">)
          n346 = call-dynamic "Read Cooler ON_OFF.vi"("Interface in"=w1071) -> ("Cooler ON/OFF"=w1070:i16)  [unwired: 8 in, 2 out]
          n347 = case shown="1" w1070 {
            tunnel: [w1086 w1093] -> w1083
            tunnel: [w1085 w1092] -> w1082
            tunnel: [35 w1091] -> w1081
            tunnel: w1080 -> [_ w1090]
            tunnel: w1073 -> [w1085 w1088]
            tunnel: w1072 -> [w1086 w1087]
            frame 1 {
              # "Se COOLER foi carregado com 1 na inicialização.\ndesvia para 35 para setar a temperatura e ligar o COOLER."
            }
            frame 0, Default {
              n348 = Increment(x=w1090) -> (x+1=w1091:i32)
              n349 = call-dynamic "Write cmd.vi"("error in (no error)"=w1088, "cmd"="SET COOLER_POWER_STATUS 0", "Device in"=w1087) -> ("error out"=w1092:errorcluster, "Device out"=w1093:refnum<class "Channel.lvclass">)  [unwired: 7 in]
            }
          }
        }
        frame 67 {
          n350 = call "Verify Timer.vi"("error in (no error)"=w1097, "State Machine in"=w1101) -> ("error out"=w1096:errorcluster, "timeout"=w1094:bool, "State Machine out"=w1098:refnum<class "State Machine.lvclass">)  [unwired: 7 in]
          n351 = call-dynamic "Write State Machine.vi"("error in (no error)"=w1096, "State Machine.lvclass"=w1098, "Device in"=w1100) -> ("error out"=w1095:errorcluster, "Device out"=w1099:refnum<class "Channel.lvclass">)  [unwired: 7 in]
          n352 = call-dynamic "Read resp.vi"("error in (no error)"=w1095, "Device in"=w1099) -> ("error out"=w1103:errorcluster, "resp"=w1108:string, "Device out"=w1104:refnum<class "Channel.lvclass">)  [unwired: 7 in]
          n353 = Equal?(x=w1108, y="DONE") -> (x = y?=w1106:bool)
          n354 = case shown="True" w1106 {
            tunnel: [w1109 w1114] -> w1105
            tunnel: w1102 -> [w1110 _]
            tunnel: w1094 -> [w1111 _]
            frame False {
              n355 = case shown="True" w1111 {
                tunnel: [w1112 40 ("State")] -> w1109
                tunnel: w1110 -> [w1112 _]
                frame False {
                }
                frame True {
                  # "configura \nExp mode"
                }
              }
            }
            frame True {
              n356 = disable-structure shown="Enabled" {
                disable-tunnel: [54 ("State") 32 ("State")] -> w1114
                frame Disabled {
                }
                frame Enabled {
                  # "Lê COOLER e \nvai pra 0."
                }
              }
            }
          }
        }
        frame 70 {
          w1120 = "" ("resp")
          # "Carrega timeout de 5 ciclos\npara resposta do ACS"
          n357 = call-dynamic "Write Timer.vi"("error in (no error)"=w1133, "Timer"=u32 5, "State Machine in"=w1135) -> ("error out"=w1137:errorcluster, "State Machine out"=w1136:refnum<class "State Machine.lvclass">)  [unwired: 7 in]
          n358 = call-dynamic "Write State Machine.vi"("error in (no error)"=w1137, "State Machine.lvclass"=w1136, "Device in"=w1134) -> ("error out"=w1132:errorcluster, "Device out"=w1119:refnum<class "Channel.lvclass">)  [unwired: 7 in]
          n359 = Bundle By Name(cluster=w1119, "stopping"=TRUE) -> (w1117:refnum<class "Channel.lvclass">)
          n360 = call-dynamic "Write cmd.vi"("error in (no error)"=w1132, "cmd"="STOP_ACQUISITION", "Device in"=w1117) -> ("error out"=w1130:errorcluster, "Device out"=w1131:refnum<class "Channel.lvclass">)  [unwired: 7 in]
          n361 = call-dynamic "Write resp.vi"("error in (no error)"=w1130, "resp"=w1120, "Device in"=w1131) -> ("error out"=w1126:errorcluster, "Device out"=w1129:refnum<class "Channel.lvclass">)  [unwired: 7 in]
          n362 = call-dynamic "Read Interface.vi"("error in (no error)"=w1126, "Channel in"=w1129) -> ("error out"=w1125:errorcluster, "Interface.lvclass"=w1124:refnum<class "Interface.lvclass">, "Channel out"=w1128:refnum<class "Channel.lvclass">)  [unwired: 7 in]
          n363 = call-dynamic "UpdateStatus.vi"("error in (no error)"=w1125, "status"=w1120, "Interface in"=w1124) -> ("error out"=w1122:errorcluster, "Interface out"=w1123:refnum<class "Interface.lvclass">)  [unwired: 7 in]
          n364 = call-dynamic "Write Interface.vi"("error in (no error)"=w1122, "Interface.lvclass"=w1123, "Channel in"=w1128) -> ("error out"=w1121:errorcluster, "Channel out"=w1127:refnum<class "Channel.lvclass">)  [unwired: 7 in]
          n365 = Increment(x=w1140) -> (x+1=w1141:i32)
        }
        frame 71 {
          w1143 = "DONE"
          n366 = call-dynamic "Read resp.vi"("error in (no error)"=w1150, "Device in"=w1151) -> ("error out"=w1147:errorcluster, "resp"=w1145:string, "Device out"=w1148:refnum<class "Channel.lvclass">)  [unwired: 7 in]
          "resp STOP" <- w1145
          n367 = Match Pattern(string=w1145, regular expression=w1143) -> (match substring=w1144:string)  [unwired: 1 in, 3 out]
          n368 = Equal?(x=w1144, y=w1143) -> ()  [unwired: 1 out]
          n369 = case shown="True" TRUE {
            tunnel: [w1152 0 ("State")] -> w1149
            tunnel: w1146 -> [w1152 _]
            frame False {
            }
            frame True {
            }
          }
        }
        frame 80 {
          n370 = call-dynamic "Write cmd.vi"("error in (no error)"=w1163, "cmd"="ABORT_ACQUISITION", "Device in"=w1162) -> ("error out"=w1157:errorcluster, "Device out"=w1158:refnum<class "Channel.lvclass">)  [unwired: 7 in]
          n371 = call-dynamic "Write resp.vi"("error in (no error)"=w1157, "resp"="", "Device in"=w1158) -> ("error out"=w1156:errorcluster, "Device out"=w1155:refnum<class "Channel.lvclass">)  [unwired: 7 in]
          n372 = Increment(x=w1160) -> (x+1=w1161:i32)
        }
        frame 81 {
          w1165 = "DONE"
          n373 = call-dynamic "Read resp.vi"("error in (no error)"=w1172, "Device in"=w1173) -> ("error out"=w1169:errorcluster, "resp"=w1167:string, "Device out"=w1170:refnum<class "Channel.lvclass">)  [unwired: 7 in]
          "resp ABORT" <- w1167
          n374 = Match Pattern(string=w1167, regular expression=w1165) -> (match substring=w1166:string)  [unwired: 1 in, 3 out]
          n375 = Equal?(x=w1166, y=w1165) -> ()  [unwired: 1 out]
          n376 = case shown="True" TRUE {
            tunnel: [w1174 0 ("State")] -> w1171
            tunnel: w1168 -> [w1174 _]
            frame False {
            }
            frame True {
            }
          }
        }
        frame 90 {
          n377 = call-dynamic "Write cmd.vi"("error in (no error)"=w1185, "cmd"="PAUSE_ACQUISITION", "Device in"=w1184) -> ("error out"=w1179:errorcluster, "Device out"=w1180:refnum<class "Channel.lvclass">)  [unwired: 7 in]
          n378 = call-dynamic "Write resp.vi"("error in (no error)"=w1179, "resp"="", "Device in"=w1180) -> ("error out"=w1178:errorcluster, "Device out"=w1177:refnum<class "Channel.lvclass">)  [unwired: 7 in]
          n379 = Increment(x=w1182) -> (x+1=w1183:i32)
        }
        frame 91 {
          w1186 = "DONE"
          n380 = call-dynamic "Read resp.vi"("error in (no error)"=w1192, "Device in"=w1193) -> ("error out"=w1190:errorcluster, "resp"=w1188:string, "Device out"=w1191:refnum<class "Channel.lvclass">)  [unwired: 7 in]
          "resp PAUSE" <- w1188
          n381 = Match Pattern(string=w1188, regular expression=w1186) -> (match substring=w1187:string)  [unwired: 1 in, 3 out]
          n382 = Equal?(x=w1187, y=w1186) -> ()  [unwired: 1 out]
        }
        frame 96 {
          n383 = call-dynamic "Write cmd.vi"("error in (no error)"=w1203, "cmd"="RESUME_ACQUISITION", "Device in"=w1202) -> ("error out"=w1197:errorcluster, "Device out"=w1198:refnum<class "Channel.lvclass">)  [unwired: 7 in]
          n384 = call-dynamic "Write resp.vi"("error in (no error)"=w1197, "resp"="", "Device in"=w1198) -> ("error out"=w1196:errorcluster, "Device out"=w1195:refnum<class "Channel.lvclass">)  [unwired: 7 in]
          n385 = Increment(x=w1200) -> (x+1=w1201:i32)
        }
        frame 97 {
          w1208 = "DONE"
          n386 = call-dynamic "Read resp.vi"("error in (no error)"=w1212, "Device in"=w1213) -> ("error out"=w1206:errorcluster, "resp"=w1210:string, "Device out"=w1211:refnum<class "Channel.lvclass">)  [unwired: 7 in]
          "resp RESUME" <- w1210
          n387 = Match Pattern(string=w1210, regular expression=w1208) -> (match substring=w1209:string)  [unwired: 1 in, 3 out]
          n388 = Equal?(x=w1209, y=w1208) -> ()  [unwired: 1 out]
          n389 = call-dynamic "Read Return State.vi"("error in (no error)"=w1206, "State Machine in"=w1207) -> ("error out"=w1205:errorcluster, "Return State"=w1204:i32)  [unwired: 7 in, 1 out]
        }
        frame 100 {
          (unwired) "S4ACS C1/C2/C3/C4 NIMAGES " ("cmd")
          n390 = call-dynamic "Write cmd.vi"("error in (no error)"=w1219, "cmd"="INIT", "Device in"=w1217) -> ("error out"=w1218:errorcluster, "Device out"=w1220:refnum<class "Channel.lvclass">)  [unwired: 7 in]
          n391 = Increment(x=w1215) -> (x+1=w1216:i32)
        }
        frame 101 {
          w1222 = "\r\n"
          n392 = call-dynamic "Read resp.vi"("error in (no error)"=w1230, "Device in"=w1231) -> ("error out"=w1227:errorcluster, "resp"=w1221:string, "Device out"=w1224:refnum<class "Channel.lvclass">)  [unwired: 7 in]
          n393 = Match Pattern(string=w1221, regular expression=w1222) -> (match substring=w1225:string)  [unwired: 1 in, 3 out]
          n394 = Equal?(x=w1225, y=w1222) -> (x = y?=w1229:bool)
          n395 = case shown="False" w1229 {
            tunnel: [w1232 u8 0] -> w1228
            tunnel: w1226 -> [w1232 _]
            tunnel: w1224 -> [w1233 w1237]
            tunnel: [w1233 w1236] -> w1223
            tunnel: w1221 -> [_ w1235]
            frame False {
            }
            frame True {
              n396 = Bundle By Name(cluster=w1237, "lastStatus"=w1235) -> (w1236:refnum<class "Channel.lvclass">)
            }
          }
        }
        frame 102 {
          w1245 = "EXPTIME "
          n397 = Unbundle By Name(w1239) -> ("lastStatus"=w1240:string)
          n398 = Match Pattern(string=w1240, regular expression=w1245) -> (match substring=w1244:string, after substring=w1242:string)  [unwired: 1 in, 2 out]
          n399 = Equal?(x=w1244, y=w1245) -> (x = y?=w1248:bool)
          n400 = case shown="True" w1248 {
            tunnel: [w1249 w1251] -> w1247
            tunnel: w1246 -> [w1249 w1251]
            tunnel: w1239 -> [w1250 w1257]
            tunnel: [w1250 w1255] -> w1243
            tunnel: w1242 -> [_ w1253]
            frame False {
            }
            frame True {
              n401 = call <vilib>:"Space Constant.vi"() -> ("String"=w1254:string)
              n402 = Match Pattern(string=w1253, regular expression=w1254) -> (before substring=w1252:string)  [unwired: 1 in, 3 out]
              n403 = Fract/Exp String To Number(string=w1252) -> (number=w1256:dbl)  [unwired: 3 in, 1 out]
              n404 = Bundle By Name(cluster=w1257, "Texp"=w1256) -> (w1255:refnum<class "Channel.lvclass">)
            }
          }
          n405 = Increment(x=w1247) -> (x+1=w1238:i32)
        }
        frame 103 {
          w1265 = "NIMAGES "
          n406 = Unbundle By Name(w1259) -> ("lastStatus"=w1260:string)
          n407 = Match Pattern(string=w1260, regular expression=w1265) -> (match substring=w1264:string, after substring=w1262:string)  [unwired: 1 in, 2 out]
          n408 = Equal?(x=w1264, y=w1265) -> (x = y?=w1268:bool)
          n409 = case shown="True" w1268 {
            tunnel: [w1269 w1271] -> w1267
            tunnel: w1266 -> [w1269 w1271]
            tunnel: w1259 -> [w1270 w1277]
            tunnel: [w1270 w1275] -> w1263
            tunnel: w1262 -> [_ w1273]
            frame False {
            }
            frame True {
              n410 = call <vilib>:"Space Constant.vi"() -> ("String"=w1274:string)
              n411 = Match Pattern(string=w1273, regular expression=w1274) -> (before substring=w1272:string)  [unwired: 1 in, 3 out]
              n412 = Fract/Exp String To Number(string=w1272) -> (number=w1276:dbl)  [unwired: 3 in, 1 out]
              n413 = Bundle By Name(cluster=w1277, "Nimages"=w1276) -> (w1275:refnum<class "Channel.lvclass">)
            }
          }
          n414 = Increment(x=w1267) -> (x+1=w1258:i32)
        }
        frame 104 {
          w1285 = "INITIAL_LINE "
          n415 = Unbundle By Name(w1279) -> ("lastStatus"=w1280:string)
          n416 = Match Pattern(string=w1280, regular expression=w1285) -> (match substring=w1284:string, after substring=w1282:string)  [unwired: 1 in, 2 out]
          n417 = Equal?(x=w1284, y=w1285) -> (x = y?=w1288:bool)
          n418 = case shown="True" w1288 {
            tunnel: [w1289 w1291] -> w1287
            tunnel: w1286 -> [w1289 w1291]
            tunnel: w1279 -> [w1290 w1297]
            tunnel: [w1290 w1295] -> w1283
            tunnel: w1282 -> [_ w1293]
            frame False {
            }
            frame True {
              n419 = call <vilib>:"Space Constant.vi"() -> ("String"=w1294:string)
              n420 = Match Pattern(string=w1293, regular expression=w1294) -> (before substring=w1292:string)  [unwired: 1 in, 3 out]
              n421 = Fract/Exp String To Number(string=w1292) -> (number=w1296:dbl)  [unwired: 3 in, 1 out]
              n422 = Bundle By Name(cluster=w1297, "InitialLine"=w1296) -> (w1295:refnum<class "Channel.lvclass">)
            }
          }
          n423 = Increment(x=w1287) -> (x+1=w1278:i32)
        }
        frame 105 {
          w1305 = "FINAL_LINE "
          n424 = Unbundle By Name(w1299) -> ("lastStatus"=w1300:string)
          n425 = Match Pattern(string=w1300, regular expression=w1305) -> (match substring=w1304:string, after substring=w1302:string)  [unwired: 1 in, 2 out]
          n426 = Equal?(x=w1304, y=w1305) -> (x = y?=w1308:bool)
          n427 = case shown="True" w1308 {
            tunnel: [w1309 w1311] -> w1307
            tunnel: w1306 -> [w1309 w1311]
            tunnel: w1299 -> [w1310 w1317]
            tunnel: [w1310 w1315] -> w1303
            tunnel: w1302 -> [_ w1313]
            frame False {
            }
            frame True {
              n428 = call <vilib>:"Space Constant.vi"() -> ("String"=w1314:string)
              n429 = Match Pattern(string=w1313, regular expression=w1314) -> (before substring=w1312:string)  [unwired: 1 in, 3 out]
              n430 = Fract/Exp String To Number(string=w1312) -> (number=w1316:dbl)  [unwired: 3 in, 1 out]
              n431 = Bundle By Name(cluster=w1317, "FinalLine"=w1316) -> (w1315:refnum<class "Channel.lvclass">)
            }
          }
          n432 = Increment(x=w1307) -> (x+1=w1298:i32)
        }
        frame 106 {
          w1325 = "INITIAL_COLUMN "
          n433 = Unbundle By Name(w1319) -> ("lastStatus"=w1320:string)
          n434 = Match Pattern(string=w1320, regular expression=w1325) -> (match substring=w1324:string, after substring=w1322:string)  [unwired: 1 in, 2 out]
          n435 = Equal?(x=w1324, y=w1325) -> (x = y?=w1328:bool)
          n436 = case shown="True" w1328 {
            tunnel: [w1329 w1331] -> w1327
            tunnel: w1326 -> [w1329 w1331]
            tunnel: w1319 -> [w1330 w1337]
            tunnel: [w1330 w1335] -> w1323
            tunnel: w1322 -> [_ w1333]
            frame False {
            }
            frame True {
              n437 = call <vilib>:"Space Constant.vi"() -> ("String"=w1334:string)
              n438 = Match Pattern(string=w1333, regular expression=w1334) -> (before substring=w1332:string)  [unwired: 1 in, 3 out]
              n439 = Fract/Exp String To Number(string=w1332) -> (number=w1336:dbl)  [unwired: 3 in, 1 out]
              n440 = Bundle By Name(cluster=w1337, "InitialColumn"=w1336) -> (w1335:refnum<class "Channel.lvclass">)
            }
          }
          n441 = Increment(x=w1327) -> (x+1=w1318:i32)
        }
        frame 107 {
          w1345 = "FINAL_COLUMN "
          n442 = Unbundle By Name(w1339) -> ("lastStatus"=w1340:string)
          n443 = Match Pattern(string=w1340, regular expression=w1345) -> (match substring=w1344:string, after substring=w1342:string)  [unwired: 1 in, 2 out]
          n444 = Equal?(x=w1344, y=w1345) -> (x = y?=w1348:bool)
          n445 = case shown="True" w1348 {
            tunnel: [w1349 w1351] -> w1347
            tunnel: w1346 -> [w1349 w1351]
            tunnel: w1339 -> [w1350 w1357]
            tunnel: [w1350 w1355] -> w1343
            tunnel: w1342 -> [_ w1353]
            frame False {
            }
            frame True {
              n446 = call <vilib>:"Space Constant.vi"() -> ("String"=w1354:string)
              n447 = Match Pattern(string=w1353, regular expression=w1354) -> (before substring=w1352:string)  [unwired: 1 in, 3 out]
              n448 = Fract/Exp String To Number(string=w1352) -> (number=w1356:dbl)  [unwired: 3 in, 1 out]
              n449 = Bundle By Name(cluster=w1357, "FinalColumn"=w1356) -> (w1355:refnum<class "Channel.lvclass">)
            }
          }
          n450 = Increment(x=w1347) -> (x+1=w1338:i32)
        }
        frame 108 {
          w1365 = "EM_GAIN "
          n451 = Unbundle By Name(w1359) -> ("lastStatus"=w1360:string)
          n452 = Match Pattern(string=w1360, regular expression=w1365) -> (match substring=w1364:string, after substring=w1362:string)  [unwired: 1 in, 2 out]
          n453 = Equal?(x=w1364, y=w1365) -> (x = y?=w1368:bool)
          n454 = case shown="True" w1368 {
            tunnel: [w1369 w1371] -> w1367
            tunnel: w1366 -> [w1369 w1371]
            tunnel: w1359 -> [w1370 w1377]
            tunnel: [w1370 w1375] -> w1363
            tunnel: w1362 -> [_ w1373]
            frame False {
            }
            frame True {
              n455 = call <vilib>:"Space Constant.vi"() -> ("String"=w1374:string)
              n456 = Match Pattern(string=w1373, regular expression=w1374) -> (before substring=w1372:string)  [unwired: 1 in, 3 out]
              n457 = Fract/Exp String To Number(string=w1372) -> (number=w1376:dbl)  [unwired: 3 in, 1 out]
              n458 = Bundle By Name(cluster=w1377, "EmGain"=w1376) -> (w1375:refnum<class "Channel.lvclass">)
            }
          }
          n459 = Increment(x=w1367) -> (x+1=w1358:i32)
        }
        frame 109 {
          w1385 = "COOLER "
          n460 = Unbundle By Name(w1379) -> ("lastStatus"=w1380:string)
          n461 = Match Pattern(string=w1380, regular expression=w1385) -> (match substring=w1384:string, after substring=w1382:string)  [unwired: 1 in, 2 out]
          n462 = Equal?(x=w1384, y=w1385) -> (x = y?=w1388:bool)
          n463 = case shown="True" w1388 {
            tunnel: [w1389 w1391] -> w1387
            tunnel: w1386 -> [w1389 w1391]
            tunnel: w1379 -> [w1390 w1398]
            tunnel: [w1390 w1397] -> w1383
            tunnel: w1382 -> [_ w1395]
            frame False {
            }
            frame True {
              n464 = call <vilib>:"Space Constant.vi"() -> ("String"=w1396:string)
              n465 = Match Pattern(string=w1395, regular expression=w1396) -> (before substring=w1394:string)  [unwired: 1 in, 3 out]
              n466 = Equal?(x=w1394, y="ON") -> (x = y?=w1392:bool)
              n467 = Bundle By Name(cluster=w1398, "Cooler Off"=w1392) -> (w1397:refnum<class "Channel.lvclass">)
            }
          }
          n468 = Increment(x=w1387) -> (x+1=w1378:i32)
        }
        frame 110 {
        }
        frame 200 {
          n469 = Unbundle By Name(w1410) -> ("Interface.lvclass"=w1409:refnum<class "Interface.lvclass">)
          n470 = call "Read Camera Setup.vi"("Interface in"=w1409) -> ("Camera Setup"=w1403:T3)  [unwired: 8 in, 2 out]
          n471 = Unbundle By Name(w1403) -> ("EXPTIME"=w1402:dbl)
          n472 = Number To Fractional String(number=w1402) -> (F-format string=w1404:string)  [unwired: 3 in]
          n473 = Concatenate Strings("SET EXPTIME " ("cmd"), w1404) -> (w1408:string)
          n474 = call-dynamic "Write cmd.vi"("error in (no error)"=w1412, "cmd"=w1408, "Device in"=w1410) -> ("error out"=w1411:errorcluster, "Device out"=w1413:refnum<class "Channel.lvclass">)  [unwired: 7 in]
          n475 = Increment(x=w1406) -> (x+1=w1407:i32)
        }
        frame 201 {
          n476 = call-dynamic "Read resp.vi"("error in (no error)"=w1421, "Device in"=w1422) -> ("error out"=w1415:errorcluster, "resp"=w1420:string, "Device out"=w1416:refnum<class "Channel.lvclass">)  [unwired: 7 in]
          n477 = Equal?(x=w1420, y="DONE") -> (x = y?=w1418:bool)
          n478 = case shown="True" w1418 {
            tunnel: [w1423 w1424] -> w1417
            tunnel: w1414 -> [w1423 w1425]
            frame False {
            }
            frame True {
              n479 = Increment(x=w1425) -> (x+1=w1424:i32)
            }
          }
        }
        frame 202 {
          n480 = call-dynamic "Write cmd.vi"("error in (no error)"=w1431, "cmd"="GET EXPTIME", "Device in"=w1429) -> ("error out"=w1430:errorcluster, "Device out"=w1432:refnum<class "Channel.lvclass">)  [unwired: 7 in]
          n481 = Increment(x=w1427) -> (x+1=w1428:i32)
        }
        frame 203 {
          n482 = call-dynamic "Read resp.vi"("error in (no error)"=w1443, "Device in"=w1444) -> ("error out"=w1441:errorcluster, "resp"=w1436:string, "Device out"=w1439:refnum<class "Channel.lvclass">)  [unwired: 7 in]
          n483 = Fract/Exp String To Number(string=w1436) -> (number=w1433:dbl)  [unwired: 3 in, 1 out]
          n484 = Unbundle By Name(w1439) -> ("Interface.lvclass"=w1438:refnum<class "Interface.lvclass">)
          n485 = call "Read Camera Setup.vi"("Interface in"=w1438) -> ("Camera Setup"=w1437:T3)  [unwired: 8 in, 2 out]
          n486 = Unbundle By Name(w1437) -> ("EXPTIME"=w1434:dbl)
          n487 = Equal?(x=w1434, y=w1433) -> (x = y?=w1435:bool)
          n488 = disable-structure shown="Enabled" {
            disable-tunnel: [w1447 224 ("State")] -> w1442
            disable-tunnel: w1440 -> [w1446 _]
            disable-tunnel: w1435 -> [w1445 _]
            frame Disabled {
              n489 = case shown="True" w1445 {
                tunnel: [w1448 w1449] -> w1447
                tunnel: w1446 -> [w1448 w1450]
                frame False {
                }
                frame True {
                  n490 = Increment(x=w1450) -> (x+1=w1449:i32)
                }
              }
            }
            frame Enabled {
            }
          }
        }
        frame 204 {
          n491 = Unbundle By Name(w1460) -> ("Interface.lvclass"=w1459:refnum<class "Interface.lvclass">)
          n492 = call "Read Camera Setup.vi"("Interface in"=w1459) -> ("Camera Setup"=w1453:T3)  [unwired: 8 in, 2 out]
          n493 = Unbundle By Name(w1453) -> ("#FRAMES"=w1452:u32)
          n494 = Number To Fractional String(number=w1452) -> (F-format string=w1454:string)  [unwired: 3 in]
          n495 = Concatenate Strings("SET #FRAMES " ("cmd"), w1454) -> (w1458:string)
          n496 = call-dynamic "Write cmd.vi"("error in (no error)"=w1462, "cmd"=w1458, "Device in"=w1460) -> ("error out"=w1461:errorcluster, "Device out"=w1463:refnum<class "Channel.lvclass">)  [unwired: 7 in]
          n497 = Increment(x=w1456) -> (x+1=w1457:i32)
        }
        frame 205 {
          n498 = call-dynamic "Read resp.vi"("error in (no error)"=w1471, "Device in"=w1472) -> ("error out"=w1465:errorcluster, "resp"=w1470:string, "Device out"=w1466:refnum<class "Channel.lvclass">)  [unwired: 7 in]
          n499 = Equal?(x=w1470, y="DONE") -> (x = y?=w1468:bool)
          n500 = case shown="True" w1468 {
            tunnel: [w1473 w1474] -> w1467
            tunnel: w1464 -> [w1473 w1475]
            frame False {
            }
            frame True {
              n501 = Increment(x=w1475) -> (x+1=w1474:i32)
            }
          }
        }
        frame 206 {
          n502 = call-dynamic "Write cmd.vi"("error in (no error)"=w1481, "cmd"="GET #FRAMES", "Device in"=w1479) -> ("error out"=w1480:errorcluster, "Device out"=w1482:refnum<class "Channel.lvclass">)  [unwired: 7 in]
          n503 = Increment(x=w1477) -> (x+1=w1478:i32)
        }
        frame 207 {
          n504 = call-dynamic "Read resp.vi"("error in (no error)"=w1494, "Device in"=w1495) -> ("error out"=w1492:errorcluster, "resp"=w1487:string, "Device out"=w1490:refnum<class "Channel.lvclass">)  [unwired: 7 in]
          n505 = Decimal String To Number(string=w1487) -> (number=w1485:i32)  [unwired: 2 in, 1 out]
          n506 = Unbundle By Name(w1490) -> ("Interface.lvclass"=w1489:refnum<class "Interface.lvclass">)
          n507 = call "Read Camera Setup.vi"("Interface in"=w1489) -> ("Camera Setup"=w1488:T3)  [unwired: 8 in, 2 out]
          n508 = To Unsigned Long Integer(number=w1485) -> (unsigned 32bit integer=w1483:u32)
          n509 = Unbundle By Name(w1488) -> ("#FRAMES"=w1484:u32)
          n510 = Equal?(x=w1484, y=w1483) -> (x = y?=w1486:bool)
          n511 = case shown="True" w1486 {
            tunnel: [w1496 w1497] -> w1493
            tunnel: w1491 -> [w1496 w1498]
            frame False {
            }
            frame True {
              n512 = Increment(x=w1498) -> (x+1=w1497:i32)
            }
          }
        }
        frame 208 {
          n513 = Unbundle By Name(w1507) -> ("Interface.lvclass"=w1506:refnum<class "Interface.lvclass">)
          n514 = call "Read Camera Setup.vi"("Interface in"=w1506) -> ("Camera Setup"=w1500:T3)  [unwired: 8 in, 2 out]
          n515 = Unbundle By Name(w1500) -> ("TRIGGER_MODE"=w1499:u8)
          n516 = Number To Fractional String(number=w1499) -> (F-format string=w1501:string)  [unwired: 3 in]
          n517 = Concatenate Strings("SET TRIGGER_MODE " ("cmd"), w1501) -> (w1505:string)
          n518 = call-dynamic "Write cmd.vi"("error in (no error)"=w1509, "cmd"=w1505, "Device in"=w1507) -> ("error out"=w1508:errorcluster, "Device out"=w1510:refnum<class "Channel.lvclass">)  [unwired: 7 in]
          n519 = Increment(x=w1503) -> (x+1=w1504:i32)
        }
        frame 209 {
          n520 = call-dynamic "Read resp.vi"("error in (no error)"=w1518, "Device in"=w1519) -> ("error out"=w1512:errorcluster, "resp"=w1517:string, "Device out"=w1513:refnum<class "Channel.lvclass">)  [unwired: 7 in]
          n521 = Equal?(x=w1517, y="DONE") -> (x = y?=w1515:bool)
          n522 = case shown="True" w1515 {
            tunnel: [w1520 w1521] -> w1514
            tunnel: w1511 -> [w1520 w1522]
            frame False {
            }
            frame True {
              n523 = Increment(x=w1522) -> (x+1=w1521:i32)
            }
          }
        }
        frame 210 {
          n524 = call-dynamic "Write cmd.vi"("error in (no error)"=w1528, "cmd"="GET TRIGGER_MODE", "Device in"=w1526) -> ("error out"=w1527:errorcluster, "Device out"=w1529:refnum<class "Channel.lvclass">)  [unwired: 7 in]
          n525 = Increment(x=w1524) -> (x+1=w1525:i32)
        }
        frame 211 {
          n526 = call-dynamic "Read resp.vi"("error in (no error)"=w1540, "Device in"=w1541) -> ("error out"=w1538:errorcluster, "resp"=w1533:string, "Device out"=w1536:refnum<class "Channel.lvclass">)  [unwired: 7 in]
          n527 = Fract/Exp String To Number(string=w1533) -> (number=w1531:dbl)  [unwired: 3 in, 1 out]
          n528 = Unbundle By Name(w1536) -> ("Interface.lvclass"=w1535:refnum<class "Interface.lvclass">)
          n529 = call "Read Camera Setup.vi"("Interface in"=w1535) -> ("Camera Setup"=w1534:T3)  [unwired: 8 in, 2 out]
          n530 = Unbundle By Name(w1534) -> ("TRIGGER_MODE"=w1530:u8)
          n531 = Equal?(x=w1530, y=w1531) -> (x = y?=w1532:bool)
          n532 = case shown="False" w1532 {
            tunnel: [w1542 w1543] -> w1539
            tunnel: w1537 -> [w1542 w1544]
            frame False {
            }
            frame True {
              n533 = Increment(x=w1544) -> (x+1=w1543:i32)
            }
          }
        }
        frame 212 {
          n534 = Unbundle By Name(w1553) -> ("Interface.lvclass"=w1552:refnum<class "Interface.lvclass">)
          n535 = call "Read Camera Setup.vi"("Interface in"=w1552) -> ("Camera Setup"=w1546:T3)  [unwired: 8 in, 2 out]
          n536 = Unbundle By Name(w1546) -> ("READ_MODE"=w1545:u8)
          n537 = Number To Fractional String(number=w1545) -> (F-format string=w1547:string)  [unwired: 3 in]
          n538 = Concatenate Strings("SET READ_MODE " ("cmd"), w1547) -> (w1551:string)
          n539 = call-dynamic "Write cmd.vi"("error in (no error)"=w1555, "cmd"=w1551, "Device in"=w1553) -> ("error out"=w1554:errorcluster, "Device out"=w1556:refnum<class "Channel.lvclass">)  [unwired: 7 in]
          n540 = Increment(x=w1549) -> (x+1=w1550:i32)
        }
        frame 213 {
          n541 = call-dynamic "Read resp.vi"("error in (no error)"=w1564, "Device in"=w1565) -> ("error out"=w1558:errorcluster, "resp"=w1563:string, "Device out"=w1559:refnum<class "Channel.lvclass">)  [unwired: 7 in]
          n542 = Equal?(x=w1563, y="DONE") -> (x = y?=w1561:bool)
          n543 = case shown="True" w1561 {
            tunnel: [w1566 w1567] -> w1560
            tunnel: w1557 -> [w1566 w1568]
            frame False {
            }
            frame True {
              n544 = Increment(x=w1568) -> (x+1=w1567:i32)
            }
          }
        }
        frame 214 {
          n545 = call-dynamic "Write cmd.vi"("error in (no error)"=w1574, "cmd"="GET READ_MODE", "Device in"=w1572) -> ("error out"=w1573:errorcluster, "Device out"=w1575:refnum<class "Channel.lvclass">)  [unwired: 7 in]
          n546 = Increment(x=w1570) -> (x+1=w1571:i32)
        }
        frame 215 {
          n547 = call-dynamic "Read resp.vi"("error in (no error)"=w1586, "Device in"=w1587) -> ("error out"=w1584:errorcluster, "resp"=w1579:string, "Device out"=w1582:refnum<class "Channel.lvclass">)  [unwired: 7 in]
          n548 = Fract/Exp String To Number(string=w1579) -> (number=w1577:dbl)  [unwired: 3 in, 1 out]
          n549 = Unbundle By Name(w1582) -> ("Interface.lvclass"=w1581:refnum<class "Interface.lvclass">)
          n550 = call "Read Camera Setup.vi"("Interface in"=w1581) -> ("Camera Setup"=w1580:T3)  [unwired: 8 in, 2 out]
          n551 = Unbundle By Name(w1580) -> ("READ_MODE"=w1576:u8)
          n552 = Equal?(x=w1576, y=w1577) -> (x = y?=w1578:bool)
          n553 = case shown="True" w1578 {
            tunnel: [w1588 w1589] -> w1585
            tunnel: w1583 -> [w1588 w1590]
            frame False {
            }
            frame True {
              n554 = Increment(x=w1590) -> (x+1=w1589:i32)
            }
          }
        }
        frame 216 {
          n555 = Unbundle By Name(w1599) -> ("Interface.lvclass"=w1598:refnum<class "Interface.lvclass">)
          n556 = call "Read Camera Setup.vi"("Interface in"=w1598) -> ("Camera Setup"=w1592:T3)  [unwired: 8 in, 2 out]
          n557 = Unbundle By Name(w1592) -> ("READOUT_RATE"=w1591:u8)
          n558 = Number To Fractional String(number=w1591) -> (F-format string=w1593:string)  [unwired: 3 in]
          n559 = Concatenate Strings("SET READOUT_RATE " ("cmd"), w1593) -> (w1597:string)
          n560 = call-dynamic "Write cmd.vi"("error in (no error)"=w1601, "cmd"=w1597, "Device in"=w1599) -> ("error out"=w1600:errorcluster, "Device out"=w1602:refnum<class "Channel.lvclass">)  [unwired: 7 in]
          n561 = Increment(x=w1595) -> (x+1=w1596:i32)
        }
        frame 217 {
          n562 = call-dynamic "Read resp.vi"("error in (no error)"=w1610, "Device in"=w1611) -> ("error out"=w1604:errorcluster, "resp"=w1609:string, "Device out"=w1605:refnum<class "Channel.lvclass">)  [unwired: 7 in]
          n563 = Equal?(x=w1609, y="DONE") -> (x = y?=w1607:bool)
          n564 = case shown="True" w1607 {
            tunnel: [w1612 w1613] -> w1606
            tunnel: w1603 -> [w1612 w1614]
            frame False {
            }
            frame True {
              n565 = Increment(x=w1614) -> (x+1=w1613:i32)
            }
          }
        }
        frame 218 {
          n566 = call-dynamic "Write cmd.vi"("error in (no error)"=w1620, "cmd"="GET READOUT_RATE", "Device in"=w1618) -> ("error out"=w1619:errorcluster, "Device out"=w1621:refnum<class "Channel.lvclass">)  [unwired: 7 in]
          n567 = Increment(x=w1616) -> (x+1=w1617:i32)
        }
        frame 219 {
          n568 = call-dynamic "Read resp.vi"("error in (no error)"=w1632, "Device in"=w1633) -> ("error out"=w1630:errorcluster, "resp"=w1625:string, "Device out"=w1628:refnum<class "Channel.lvclass">)  [unwired: 7 in]
          n569 = Fract/Exp String To Number(string=w1625) -> (number=w1623:dbl)  [unwired: 3 in, 1 out]
          n570 = Unbundle By Name(w1628) -> ("Interface.lvclass"=w1627:refnum<class "Interface.lvclass">)
          n571 = call "Read Camera Setup.vi"("Interface in"=w1627) -> ("Camera Setup"=w1626:T3)  [unwired: 8 in, 2 out]
          n572 = Unbundle By Name(w1626) -> ("READOUT_RATE"=w1622:u8)
          n573 = Equal?(x=w1622, y=w1623) -> (x = y?=w1624:bool)
          n574 = case shown="True" w1624 {
            tunnel: [w1634 w1635] -> w1631
            tunnel: w1629 -> [w1634 w1636]
            frame False {
            }
            frame True {
              n575 = Increment(x=w1636) -> (x+1=w1635:i32)
            }
          }
        }
        frame 220 {
          n576 = Unbundle By Name(w1645) -> ("Interface.lvclass"=w1644:refnum<class "Interface.lvclass">)
          n577 = call "Read Camera Setup.vi"("Interface in"=w1644) -> ("Camera Setup"=w1638:T3)  [unwired: 8 in, 2 out]
          n578 = Unbundle By Name(w1638) -> ("VERTICAL_SHIFT_SPEED"=w1637:u8)
          n579 = Number To Fractional String(number=w1637) -> (F-format string=w1639:string)  [unwired: 3 in]
          n580 = Concatenate Strings("SET VERTICAL_SHIFT_SPEED " ("cmd"), w1639) -> (w1643:string)
          n581 = call-dynamic "Write cmd.vi"("error in (no error)"=w1647, "cmd"=w1643, "Device in"=w1645) -> ("error out"=w1646:errorcluster, "Device out"=w1648:refnum<class "Channel.lvclass">)  [unwired: 7 in]
          n582 = Increment(x=w1641) -> (x+1=w1642:i32)
        }
        frame 221 {
          n583 = call-dynamic "Read resp.vi"("error in (no error)"=w1656, "Device in"=w1657) -> ("error out"=w1650:errorcluster, "resp"=w1655:string, "Device out"=w1651:refnum<class "Channel.lvclass">)  [unwired: 7 in]
          n584 = Equal?(x=w1655, y="DONE") -> (x = y?=w1653:bool)
          n585 = case shown="True" w1653 {
            tunnel: [w1658 w1659] -> w1652
            tunnel: w1649 -> [w1658 w1660]
            frame False {
            }
            frame True {
              n586 = Increment(x=w1660) -> (x+1=w1659:i32)
            }
          }
        }
        frame 222 {
          n587 = call-dynamic "Write cmd.vi"("error in (no error)"=w1666, "cmd"="GET VERTICAL_SHIFT_SPEED", "Device in"=w1664) -> ("error out"=w1665:errorcluster, "Device out"=w1667:refnum<class "Channel.lvclass">)  [unwired: 7 in]
          n588 = Increment(x=w1662) -> (x+1=w1663:i32)
        }
        frame 223 {
          n589 = call-dynamic "Read resp.vi"("error in (no error)"=w1678, "Device in"=w1679) -> ("error out"=w1676:errorcluster, "resp"=w1671:string, "Device out"=w1674:refnum<class "Channel.lvclass">)  [unwired: 7 in]
          n590 = Fract/Exp String To Number(string=w1671) -> (number=w1669:dbl)  [unwired: 3 in, 1 out]
          n591 = Unbundle By Name(w1674) -> ("Interface.lvclass"=w1673:refnum<class "Interface.lvclass">)
          n592 = call "Read Camera Setup.vi"("Interface in"=w1673) -> ("Camera Setup"=w1672:T3)  [unwired: 8 in, 2 out]
          n593 = Unbundle By Name(w1672) -> ("VERTICAL_SHIFT_SPEED"=w1668:u8)
          n594 = Equal?(x=w1668, y=w1669) -> (x = y?=w1670:bool)
          n595 = case shown="True" w1670 {
            tunnel: [w1680 w1681] -> w1677
            tunnel: w1675 -> [w1680 w1682]
            frame False {
            }
            frame True {
              n596 = Increment(x=w1682) -> (x+1=w1681:i32)
            }
          }
        }
        frame 224 {
          n597 = Unbundle By Name(w1691) -> ("Interface.lvclass"=w1690:refnum<class "Interface.lvclass">)
          n598 = call "Read Camera Setup.vi"("Interface in"=w1690) -> ("Camera Setup"=w1684:T3)  [unwired: 8 in, 2 out]
          n599 = Unbundle By Name(w1684) -> ("PREAMP"=w1683:u8)
          n600 = Number To Fractional String(number=w1683) -> (F-format string=w1685:string)  [unwired: 3 in]
          n601 = Concatenate Strings("SET PREAMP " ("cmd"), w1685) -> (w1689:string)
          n602 = call-dynamic "Write cmd.vi"("error in (no error)"=w1693, "cmd"=w1689, "Device in"=w1691) -> ("error out"=w1692:errorcluster, "Device out"=w1694:refnum<class "Channel.lvclass">)  [unwired: 7 in]
          n603 = Increment(x=w1687) -> (x+1=w1688:i32)
        }
        frame 225 {
          n604 = call-dynamic "Read resp.vi"("error in (no error)"=w1702, "Device in"=w1703) -> ("error out"=w1696:errorcluster, "resp"=w1701:string, "Device out"=w1697:refnum<class "Channel.lvclass">)  [unwired: 7 in]
          n605 = Equal?(x=w1701, y="DONE") -> (x = y?=w1699:bool)
          n606 = case shown="True" w1699 {
            tunnel: [w1704 w1705] -> w1698
            tunnel: w1695 -> [w1704 w1706]
            frame False {
            }
            frame True {
              n607 = Increment(x=w1706) -> (x+1=w1705:i32)
            }
          }
        }
        frame 226 {
          n608 = call-dynamic "Write cmd.vi"("error in (no error)"=w1712, "cmd"="GET PREAMP", "Device in"=w1710) -> ("error out"=w1711:errorcluster, "Device out"=w1713:refnum<class "Channel.lvclass">)  [unwired: 7 in]
          n609 = Increment(x=w1708) -> (x+1=w1709:i32)
        }
        frame 227 {
          n610 = call-dynamic "Read resp.vi"("error in (no error)"=w1724, "Device in"=w1725) -> ("error out"=w1722:errorcluster, "resp"=w1717:string, "Device out"=w1720:refnum<class "Channel.lvclass">)  [unwired: 7 in]
          n611 = Fract/Exp String To Number(string=w1717) -> (number=w1715:dbl)  [unwired: 3 in, 1 out]
          n612 = Unbundle By Name(w1720) -> ("Interface.lvclass"=w1719:refnum<class "Interface.lvclass">)
          n613 = call "Read Camera Setup.vi"("Interface in"=w1719) -> ("Camera Setup"=w1718:T3)  [unwired: 8 in, 2 out]
          n614 = Unbundle By Name(w1718) -> ("PREAMP"=w1714:u8)
          n615 = Equal?(x=w1714, y=w1715) -> (x = y?=w1716:bool)
          n616 = case shown="True" w1716 {
            tunnel: [w1726 w1727] -> w1723
            tunnel: w1721 -> [w1726 w1728]
            frame False {
            }
            frame True {
              n617 = Increment(x=w1728) -> (x+1=w1727:i32)
            }
          }
        }
        frame 228 {
          n618 = Unbundle By Name(w1737) -> ("Interface.lvclass"=w1736:refnum<class "Interface.lvclass">)
          n619 = call "Read Camera Setup.vi"("Interface in"=w1736) -> ("Camera Setup"=w1730:T3)  [unwired: 8 in, 2 out]
          n620 = Unbundle By Name(w1730) -> ("EM_MODE"=w1729:u8)
          n621 = Number To Fractional String(number=w1729) -> (F-format string=w1731:string)  [unwired: 3 in]
          n622 = Concatenate Strings("SET EM_MODE " ("cmd"), w1731) -> (w1735:string)
          n623 = call-dynamic "Write cmd.vi"("error in (no error)"=w1739, "cmd"=w1735, "Device in"=w1737) -> ("error out"=w1738:errorcluster, "Device out"=w1740:refnum<class "Channel.lvclass">)  [unwired: 7 in]
          n624 = Increment(x=w1733) -> (x+1=w1734:i32)
        }
        frame 229 {
          n625 = call-dynamic "Read resp.vi"("error in (no error)"=w1748, "Device in"=w1749) -> ("error out"=w1742:errorcluster, "resp"=w1747:string, "Device out"=w1743:refnum<class "Channel.lvclass">)  [unwired: 7 in]
          n626 = Equal?(x=w1747, y="DONE") -> (x = y?=w1745:bool)
          n627 = case shown="True" w1745 {
            tunnel: [w1750 w1751] -> w1744
            tunnel: w1741 -> [w1750 w1752]
            frame False {
            }
            frame True {
              n628 = Increment(x=w1752) -> (x+1=w1751:i32)
            }
          }
        }
        frame 230 {
          n629 = call-dynamic "Write cmd.vi"("error in (no error)"=w1758, "cmd"="GET EM_MODE", "Device in"=w1756) -> ("error out"=w1757:errorcluster, "Device out"=w1759:refnum<class "Channel.lvclass">)  [unwired: 7 in]
          n630 = Increment(x=w1754) -> (x+1=w1755:i32)
        }
        frame 231 {
          n631 = call-dynamic "Read resp.vi"("error in (no error)"=w1770, "Device in"=w1771) -> ("error out"=w1768:errorcluster, "resp"=w1763:string, "Device out"=w1766:refnum<class "Channel.lvclass">)  [unwired: 7 in]
          n632 = Fract/Exp String To Number(string=w1763) -> (number=w1761:dbl)  [unwired: 3 in, 1 out]
          n633 = Unbundle By Name(w1766) -> ("Interface.lvclass"=w1765:refnum<class "Interface.lvclass">)
          n634 = call "Read Camera Setup.vi"("Interface in"=w1765) -> ("Camera Setup"=w1764:T3)  [unwired: 8 in, 2 out]
          n635 = Unbundle By Name(w1764) -> ("EM_MODE"=w1760:u8)
          n636 = Equal?(x=w1760, y=w1761) -> (x = y?=w1762:bool)
          n637 = case shown="True" w1762 {
            tunnel: [w1772 w1773] -> w1769
            tunnel: w1767 -> [w1772 w1774]
            frame False {
            }
            frame True {
              n638 = Increment(x=w1774) -> (x+1=w1773:i32)
            }
          }
        }
        frame 232 {
          n639 = Unbundle By Name(w1783) -> ("Interface.lvclass"=w1782:refnum<class "Interface.lvclass">)
          n640 = call "Read Camera Setup.vi"("Interface in"=w1782) -> ("Camera Setup"=w1776:T3)  [unwired: 8 in, 2 out]
          n641 = Unbundle By Name(w1776) -> ("EM_GAIN"=w1775:u16)
          n642 = Number To Fractional String(number=w1775) -> (F-format string=w1777:string)  [unwired: 3 in]
          n643 = Concatenate Strings("SET EM_GAIN " ("cmd"), w1777) -> (w1781:string)
          n644 = call-dynamic "Write cmd.vi"("error in (no error)"=w1785, "cmd"=w1781, "Device in"=w1783) -> ("error out"=w1784:errorcluster, "Device out"=w1786:refnum<class "Channel.lvclass">)  [unwired: 7 in]
          n645 = Increment(x=w1779) -> (x+1=w1780:i32)
        }
        frame 233 {
          n646 = call-dynamic "Read resp.vi"("error in (no error)"=w1794, "Device in"=w1795) -> ("error out"=w1788:errorcluster, "resp"=w1793:string, "Device out"=w1789:refnum<class "Channel.lvclass">)  [unwired: 7 in]
          n647 = Equal?(x=w1793, y="DONE") -> (x = y?=w1791:bool)
          n648 = case shown="True" w1791 {
            tunnel: [w1796 w1797] -> w1790
            tunnel: w1787 -> [w1796 w1798]
            frame False {
            }
            frame True {
              n649 = Increment(x=w1798) -> (x+1=w1797:i32)
            }
          }
        }
        frame 234 {
          n650 = call-dynamic "Write cmd.vi"("error in (no error)"=w1804, "cmd"="GET EM_GAIN", "Device in"=w1802) -> ("error out"=w1803:errorcluster, "Device out"=w1805:refnum<class "Channel.lvclass">)  [unwired: 7 in]
          n651 = Increment(x=w1800) -> (x+1=w1801:i32)
        }
        frame 235 {
          n652 = call-dynamic "Read resp.vi"("error in (no error)"=w1816, "Device in"=w1817) -> ("error out"=w1814:errorcluster, "resp"=w1809:string, "Device out"=w1812:refnum<class "Channel.lvclass">)  [unwired: 7 in]
          n653 = Fract/Exp String To Number(string=w1809) -> (number=w1807:dbl)  [unwired: 3 in, 1 out]
          n654 = Unbundle By Name(w1812) -> ("Interface.lvclass"=w1811:refnum<class "Interface.lvclass">)
          n655 = call "Read Camera Setup.vi"("Interface in"=w1811) -> ("Camera Setup"=w1810:T3)  [unwired: 8 in, 2 out]
          n656 = Unbundle By Name(w1810) -> ("EM_GAIN"=w1806:u16)
          n657 = Equal?(x=w1806, y=w1807) -> (x = y?=w1808:bool)
          n658 = disable-structure shown="Enabled" {
            disable-tunnel: [w1820 264 ("State")] -> w1815
            disable-tunnel: w1813 -> [w1819 _]
            disable-tunnel: w1808 -> [w1818 _]
            frame Disabled {
              n659 = case shown="True" w1818 {
                tunnel: [w1821 w1822] -> w1820
                tunnel: w1819 -> [w1821 w1823]
                frame False {
                }
                frame True {
                  n660 = Increment(x=w1823) -> (x+1=w1822:i32)
                }
              }
            }
            frame Enabled {
            }
          }
        }
        frame 236 {
          n661 = Unbundle By Name(w1833) -> ("Interface.lvclass"=w1832:refnum<class "Interface.lvclass">)
          n662 = call "Read Camera Setup.vi"("Interface in"=w1832) -> ("Camera Setup"=w1826:T3)  [unwired: 8 in, 2 out]
          n663 = Unbundle By Name(w1826) -> ("ACQUISITION_MODE"=w1825:u8)
          n664 = Number To Fractional String(number=w1825) -> (F-format string=w1827:string)  [unwired: 3 in]
          n665 = Concatenate Strings("SET ACQUISITION_MODE " ("cmd"), w1827) -> (w1831:string)
          n666 = call-dynamic "Write cmd.vi"("error in (no error)"=w1835, "cmd"=w1831, "Device in"=w1833) -> ("error out"=w1834:errorcluster, "Device out"=w1836:refnum<class "Channel.lvclass">)  [unwired: 7 in]
          n667 = Increment(x=w1829) -> (x+1=w1830:i32)
        }
        frame 237 {
          n668 = call-dynamic "Read resp.vi"("error in (no error)"=w1844, "Device in"=w1845) -> ("error out"=w1838:errorcluster, "resp"=w1843:string, "Device out"=w1839:refnum<class "Channel.lvclass">)  [unwired: 7 in]
          n669 = Equal?(x=w1843, y="DONE") -> (x = y?=w1841:bool)
          n670 = case shown="True" w1841 {
            tunnel: [w1846 w1847] -> w1840
            tunnel: w1837 -> [w1846 w1848]
            frame False {
            }
            frame True {
              n671 = Increment(x=w1848) -> (x+1=w1847:i32)
            }
          }
        }
        frame 238 {
          n672 = call-dynamic "Write cmd.vi"("error in (no error)"=w1854, "cmd"="GET ACQUISITION_MODE", "Device in"=w1852) -> ("error out"=w1853:errorcluster, "Device out"=w1855:refnum<class "Channel.lvclass">)  [unwired: 7 in]
          n673 = Increment(x=w1850) -> (x+1=w1851:i32)
        }
        frame 239 {
          n674 = call-dynamic "Read resp.vi"("error in (no error)"=w1866, "Device in"=w1867) -> ("error out"=w1864:errorcluster, "resp"=w1859:string, "Device out"=w1862:refnum<class "Channel.lvclass">)  [unwired: 7 in]
          n675 = Fract/Exp String To Number(string=w1859) -> (number=w1857:dbl)  [unwired: 3 in, 1 out]
          n676 = Unbundle By Name(w1862) -> ("Interface.lvclass"=w1861:refnum<class "Interface.lvclass">)
          n677 = call "Read Camera Setup.vi"("Interface in"=w1861) -> ("Camera Setup"=w1860:T3)  [unwired: 8 in, 2 out]
          n678 = Unbundle By Name(w1860) -> ("ACQUISITION_MODE"=w1856:u8)
          n679 = Equal?(x=w1856, y=w1857) -> (x = y?=w1858:bool)
          n680 = case shown="True" w1858 {
            tunnel: [w1868 w1869] -> w1865
            tunnel: w1863 -> [w1868 w1870]
            frame False {
            }
            frame True {
              n681 = Increment(x=w1870) -> (x+1=w1869:i32)
            }
          }
        }
        frame 240 {
          n682 = Unbundle By Name(w1879) -> ("Interface.lvclass"=w1878:refnum<class "Interface.lvclass">)
          n683 = call "Read Camera Setup.vi"("Interface in"=w1878) -> ("Camera Setup"=w1872:T3)  [unwired: 8 in, 2 out]
          n684 = Unbundle By Name(w1872) -> ("SHUTTER_MODE"=w1871:u8)
          n685 = Number To Fractional String(number=w1871) -> (F-format string=w1873:string)  [unwired: 3 in]
          n686 = Concatenate Strings("SET SHUTTER_MODE " ("cmd"), w1873) -> (w1877:string)
          n687 = call-dynamic "Write cmd.vi"("error in (no error)"=w1881, "cmd"=w1877, "Device in"=w1879) -> ("error out"=w1880:errorcluster, "Device out"=w1882:refnum<class "Channel.lvclass">)  [unwired: 7 in]
          n688 = Increment(x=w1875) -> (x+1=w1876:i32)
        }
        frame 241 {
          n689 = call-dynamic "Read resp.vi"("error in (no error)"=w1890, "Device in"=w1891) -> ("error out"=w1884:errorcluster, "resp"=w1889:string, "Device out"=w1885:refnum<class "Channel.lvclass">)  [unwired: 7 in]
          n690 = Equal?(x=w1889, y="DONE") -> (x = y?=w1887:bool)
          n691 = case shown="True" w1887 {
            tunnel: [w1892 w1893] -> w1886
            tunnel: w1883 -> [w1892 w1894]
            frame False {
            }
            frame True {
              n692 = Increment(x=w1894) -> (x+1=w1893:i32)
            }
          }
        }
        frame 242 {
          n693 = call-dynamic "Write cmd.vi"("error in (no error)"=w1900, "cmd"="GET SHUTTER_MODE", "Device in"=w1898) -> ("error out"=w1899:errorcluster, "Device out"=w1901:refnum<class "Channel.lvclass">)  [unwired: 7 in]
          n694 = Increment(x=w1896) -> (x+1=w1897:i32)
        }
        frame 243 {
          n695 = call-dynamic "Read resp.vi"("error in (no error)"=w1912, "Device in"=w1913) -> ("error out"=w1910:errorcluster, "resp"=w1905:string, "Device out"=w1908:refnum<class "Channel.lvclass">)  [unwired: 7 in]
          n696 = Fract/Exp String To Number(string=w1905) -> (number=w1903:dbl)  [unwired: 3 in, 1 out]
          n697 = Unbundle By Name(w1908) -> ("Interface.lvclass"=w1907:refnum<class "Interface.lvclass">)
          n698 = call "Read Camera Setup.vi"("Interface in"=w1907) -> ("Camera Setup"=w1906:T3)  [unwired: 8 in, 2 out]
          n699 = Unbundle By Name(w1906) -> ("SHUTTER_MODE"=w1902:u8)
          n700 = Equal?(x=w1902, y=w1903) -> (x = y?=w1904:bool)
          n701 = case shown="True" w1904 {
            tunnel: [w1914 w1915] -> w1911
            tunnel: w1909 -> [w1914 w1916]
            frame False {
            }
            frame True {
              n702 = Increment(x=w1916) -> (x+1=w1915:i32)
            }
          }
        }
        frame 244 {
          n703 = Unbundle By Name(w1925) -> ("Interface.lvclass"=w1924:refnum<class "Interface.lvclass">)
          n704 = call "Read Camera Setup.vi"("Interface in"=w1924) -> ("Camera Setup"=w1918:T3)  [unwired: 8 in, 2 out]
          n705 = Unbundle By Name(w1918) -> ("SHUTTER_TTL"=w1917:u8)
          n706 = Number To Fractional String(number=w1917) -> (F-format string=w1919:string)  [unwired: 3 in]
          n707 = Concatenate Strings("SET SHUTTER_TTL " ("cmd"), w1919) -> (w1923:string)
          n708 = call-dynamic "Write cmd.vi"("error in (no error)"=w1927, "cmd"=w1923, "Device in"=w1925) -> ("error out"=w1926:errorcluster, "Device out"=w1928:refnum<class "Channel.lvclass">)  [unwired: 7 in]
          n709 = Increment(x=w1921) -> (x+1=w1922:i32)
        }
        frame 245 {
          n710 = call-dynamic "Read resp.vi"("error in (no error)"=w1936, "Device in"=w1937) -> ("error out"=w1930:errorcluster, "resp"=w1935:string, "Device out"=w1931:refnum<class "Channel.lvclass">)  [unwired: 7 in]
          n711 = Equal?(x=w1935, y="DONE") -> (x = y?=w1933:bool)
          n712 = case shown="True" w1933 {
            tunnel: [w1938 w1939] -> w1932
            tunnel: w1929 -> [w1938 w1940]
            frame False {
            }
            frame True {
              n713 = Increment(x=w1940) -> (x+1=w1939:i32)
            }
          }
        }
        frame 246 {
          n714 = call-dynamic "Write cmd.vi"("error in (no error)"=w1946, "cmd"="GET SHUTTER_TTL", "Device in"=w1944) -> ("error out"=w1945:errorcluster, "Device out"=w1947:refnum<class "Channel.lvclass">)  [unwired: 7 in]
          n715 = Increment(x=w1942) -> (x+1=w1943:i32)
        }
        frame 247 {
          n716 = call-dynamic "Read resp.vi"("error in (no error)"=w1958, "Device in"=w1959) -> ("error out"=w1956:errorcluster, "resp"=w1951:string, "Device out"=w1954:refnum<class "Channel.lvclass">)  [unwired: 7 in]
          n717 = Fract/Exp String To Number(string=w1951) -> (number=w1949:dbl)  [unwired: 3 in, 1 out]
          n718 = Unbundle By Name(w1954) -> ("Interface.lvclass"=w1953:refnum<class "Interface.lvclass">)
          n719 = call "Read Camera Setup.vi"("Interface in"=w1953) -> ("Camera Setup"=w1952:T3)  [unwired: 8 in, 2 out]
          n720 = Unbundle By Name(w1952) -> ("SHUTTER_TTL"=w1948:u8)
          n721 = Equal?(x=w1948, y=w1949) -> (x = y?=w1950:bool)
          n722 = case shown="True" w1950 {
            tunnel: [w1960 w1961] -> w1957
            tunnel: w1955 -> [w1960 w1962]
            frame False {
            }
            frame True {
              n723 = Increment(x=w1962) -> (x+1=w1961:i32)
            }
          }
        }
        frame 248 {
          n724 = Unbundle By Name(w1971) -> ("Interface.lvclass"=w1970:refnum<class "Interface.lvclass">)
          n725 = call "Read Camera Setup.vi"("Interface in"=w1970) -> ("Camera Setup"=w1964:T3)  [unwired: 8 in, 2 out]
          n726 = Unbundle By Name(w1964) -> ("SHUTTER_OPENNING_TIME"=w1963:u16)
          n727 = Number To Fractional String(number=w1963) -> (F-format string=w1965:string)  [unwired: 3 in]
          n728 = Concatenate Strings("SET SHUTTER_OPENNING_TIME " ("cmd"), w1965) -> (w1969:string)
          n729 = call-dynamic "Write cmd.vi"("error in (no error)"=w1973, "cmd"=w1969, "Device in"=w1971) -> ("error out"=w1972:errorcluster, "Device out"=w1974:refnum<class "Channel.lvclass">)  [unwired: 7 in]
          n730 = Increment(x=w1967) -> (x+1=w1968:i32)
        }
        frame 249 {
          n731 = call-dynamic "Read resp.vi"("error in (no error)"=w1982, "Device in"=w1983) -> ("error out"=w1976:errorcluster, "resp"=w1981:string, "Device out"=w1977:refnum<class "Channel.lvclass">)  [unwired: 7 in]
          n732 = Equal?(x=w1981, y="DONE") -> (x = y?=w1979:bool)
          n733 = case shown="True" w1979 {
            tunnel: [w1984 w1985] -> w1978
            tunnel: w1975 -> [w1984 w1986]
            frame False {
            }
            frame True {
              n734 = Increment(x=w1986) -> (x+1=w1985:i32)
            }
          }
        }
        frame 250 {
          n735 = call-dynamic "Write cmd.vi"("error in (no error)"=w1992, "cmd"="GET SHUTTER_OPENNING_TIME", "Device in"=w1990) -> ("error out"=w1991:errorcluster, "Device out"=w1993:refnum<class "Channel.lvclass">)  [unwired: 7 in]
          n736 = Increment(x=w1988) -> (x+1=w1989:i32)
        }
        frame 251 {
          n737 = call-dynamic "Read resp.vi"("error in (no error)"=w2004, "Device in"=w2005) -> ("error out"=w2002:errorcluster, "resp"=w1997:string, "Device out"=w2000:refnum<class "Channel.lvclass">)  [unwired: 7 in]
          n738 = Fract/Exp String To Number(string=w1997) -> (number=w1995:dbl)  [unwired: 3 in, 1 out]
          n739 = Unbundle By Name(w2000) -> ("Interface.lvclass"=w1999:refnum<class "Interface.lvclass">)
          n740 = call "Read Camera Setup.vi"("Interface in"=w1999) -> ("Camera Setup"=w1998:T3)  [unwired: 8 in, 2 out]
          n741 = Unbundle By Name(w1998) -> ("SHUTTER_OPENNING_TIME"=w1994:u16)
          n742 = Equal?(x=w1994, y=w1995) -> (x = y?=w1996:bool)
          n743 = case shown="True" w1996 {
            tunnel: [w2006 w2007] -> w2003
            tunnel: w2001 -> [w2006 w2008]
            frame False {
            }
            frame True {
              n744 = Increment(x=w2008) -> (x+1=w2007:i32)
            }
          }
        }
        frame 252 {
          n745 = Unbundle By Name(w2017) -> ("Interface.lvclass"=w2016:refnum<class "Interface.lvclass">)
          n746 = call "Read Camera Setup.vi"("Interface in"=w2016) -> ("Camera Setup"=w2010:T3)  [unwired: 8 in, 2 out]
          n747 = Unbundle By Name(w2010) -> ("SHUTTER_CLOSING_TIME"=w2009:u16)
          n748 = Number To Fractional String(number=w2009) -> (F-format string=w2011:string)  [unwired: 3 in]
          n749 = Concatenate Strings("SET SHUTTER_CLOSING_TIME " ("cmd"), w2011) -> (w2015:string)
          n750 = call-dynamic "Write cmd.vi"("error in (no error)"=w2019, "cmd"=w2015, "Device in"=w2017) -> ("error out"=w2018:errorcluster, "Device out"=w2020:refnum<class "Channel.lvclass">)  [unwired: 7 in]
          n751 = Increment(x=w2013) -> (x+1=w2014:i32)
        }
        frame 253 {
          n752 = call-dynamic "Read resp.vi"("error in (no error)"=w2028, "Device in"=w2029) -> ("error out"=w2022:errorcluster, "resp"=w2027:string, "Device out"=w2023:refnum<class "Channel.lvclass">)  [unwired: 7 in]
          n753 = Equal?(x=w2027, y="DONE") -> (x = y?=w2025:bool)
          n754 = case shown="True" w2025 {
            tunnel: [w2030 w2031] -> w2024
            tunnel: w2021 -> [w2030 w2032]
            frame False {
            }
            frame True {
              n755 = Increment(x=w2032) -> (x+1=w2031:i32)
            }
          }
        }
        frame 254 {
          n756 = call-dynamic "Write cmd.vi"("error in (no error)"=w2038, "cmd"="GET SHUTTER_CLOSING_TIME", "Device in"=w2036) -> ("error out"=w2037:errorcluster, "Device out"=w2039:refnum<class "Channel.lvclass">)  [unwired: 7 in]
          n757 = Increment(x=w2034) -> (x+1=w2035:i32)
        }
        frame 255 {
          n758 = call-dynamic "Read resp.vi"("error in (no error)"=w2050, "Device in"=w2051) -> ("error out"=w2048:errorcluster, "resp"=w2043:string, "Device out"=w2046:refnum<class "Channel.lvclass">)  [unwired: 7 in]
          n759 = Fract/Exp String To Number(string=w2043) -> (number=w2041:dbl)  [unwired: 3 in, 1 out]
          n760 = Unbundle By Name(w2046) -> ("Interface.lvclass"=w2045:refnum<class "Interface.lvclass">)
          n761 = call "Read Camera Setup.vi"("Interface in"=w2045) -> ("Camera Setup"=w2044:T3)  [unwired: 8 in, 2 out]
          n762 = Unbundle By Name(w2044) -> ("SHUTTER_CLOSING_TIME"=w2040:u16)
          n763 = Equal?(x=w2040, y=w2041) -> (x = y?=w2042:bool)
          n764 = case shown="True" w2042 {
            tunnel: [w2052 w2053] -> w2049
            tunnel: w2047 -> [w2052 w2054]
            frame False {
            }
            frame True {
              n765 = Increment(x=w2054) -> (x+1=w2053:i32)
            }
          }
        }
        frame 256 {
          n766 = Unbundle By Name(w2063) -> ("Interface.lvclass"=w2062:refnum<class "Interface.lvclass">)
          n767 = call "Read Camera Setup.vi"("Interface in"=w2062) -> ("Camera Setup"=w2056:T3)  [unwired: 8 in, 2 out]
          n768 = Unbundle By Name(w2056) -> ("HBIN"=w2055:u16)
          n769 = Number To Fractional String(number=w2055) -> (F-format string=w2057:string)  [unwired: 3 in]
          n770 = Concatenate Strings("SET HBIN " ("cmd"), w2057) -> (w2061:string)
          n771 = call-dynamic "Write cmd.vi"("error in (no error)"=w2065, "cmd"=w2061, "Device in"=w2063) -> ("error out"=w2064:errorcluster, "Device out"=w2066:refnum<class "Channel.lvclass">)  [unwired: 7 in]
          n772 = Increment(x=w2059) -> (x+1=w2060:i32)
        }
        frame 257 {
          n773 = call-dynamic "Read resp.vi"("error in (no error)"=w2074, "Device in"=w2075) -> ("error out"=w2068:errorcluster, "resp"=w2073:string, "Device out"=w2069:refnum<class "Channel.lvclass">)  [unwired: 7 in]
          n774 = Equal?(x=w2073, y="DONE") -> (x = y?=w2071:bool)
          n775 = case shown="True" w2071 {
            tunnel: [w2076 w2077] -> w2070
            tunnel: w2067 -> [w2076 w2078]
            frame False {
            }
            frame True {
              n776 = Increment(x=w2078) -> (x+1=w2077:i32)
            }
          }
        }
        frame 258 {
          n777 = call-dynamic "Write cmd.vi"("error in (no error)"=w2084, "cmd"="GET HBIN", "Device in"=w2082) -> ("error out"=w2083:errorcluster, "Device out"=w2085:refnum<class "Channel.lvclass">)  [unwired: 7 in]
          n778 = Increment(x=w2080) -> (x+1=w2081:i32)
        }
        frame 259 {
          n779 = call-dynamic "Read resp.vi"("error in (no error)"=w2096, "Device in"=w2097) -> ("error out"=w2094:errorcluster, "resp"=w2089:string, "Device out"=w2092:refnum<class "Channel.lvclass">)  [unwired: 7 in]
          n780 = Fract/Exp String To Number(string=w2089) -> (number=w2087:dbl)  [unwired: 3 in, 1 out]
          n781 = Unbundle By Name(w2092) -> ("Interface.lvclass"=w2091:refnum<class "Interface.lvclass">)
          n782 = call "Read Camera Setup.vi"("Interface in"=w2091) -> ("Camera Setup"=w2090:T3)  [unwired: 8 in, 2 out]
          n783 = Unbundle By Name(w2090) -> ("HBIN"=w2086:u16)
          n784 = Equal?(x=w2086, y=w2087) -> (x = y?=w2088:bool)
          n785 = case shown="True" w2088 {
            tunnel: [w2098 w2099] -> w2095
            tunnel: w2093 -> [w2098 w2100]
            frame False {
            }
            frame True {
              n786 = Increment(x=w2100) -> (x+1=w2099:i32)
            }
          }
        }
        frame 260 {
          n787 = Unbundle By Name(w2109) -> ("Interface.lvclass"=w2108:refnum<class "Interface.lvclass">)
          n788 = call "Read Camera Setup.vi"("Interface in"=w2108) -> ("Camera Setup"=w2102:T3)  [unwired: 8 in, 2 out]
          n789 = Unbundle By Name(w2102) -> ("VBIN"=w2101:u16)
          n790 = Number To Fractional String(number=w2101) -> (F-format string=w2103:string)  [unwired: 3 in]
          n791 = Concatenate Strings("SET VBIN " ("cmd"), w2103) -> (w2107:string)
          n792 = call-dynamic "Write cmd.vi"("error in (no error)"=w2111, "cmd"=w2107, "Device in"=w2109) -> ("error out"=w2110:errorcluster, "Device out"=w2112:refnum<class "Channel.lvclass">)  [unwired: 7 in]
          n793 = Increment(x=w2105) -> (x+1=w2106:i32)
        }
        frame 261 {
          n794 = call-dynamic "Read resp.vi"("error in (no error)"=w2120, "Device in"=w2121) -> ("error out"=w2114:errorcluster, "resp"=w2119:string, "Device out"=w2115:refnum<class "Channel.lvclass">)  [unwired: 7 in]
          n795 = Equal?(x=w2119, y="DONE") -> (x = y?=w2117:bool)
          n796 = case shown="True" w2117 {
            tunnel: [w2122 w2123] -> w2116
            tunnel: w2113 -> [w2122 w2124]
            frame False {
            }
            frame True {
              n797 = Increment(x=w2124) -> (x+1=w2123:i32)
            }
          }
        }
        frame 262 {
          n798 = call-dynamic "Write cmd.vi"("error in (no error)"=w2130, "cmd"="GET VBIN", "Device in"=w2128) -> ("error out"=w2129:errorcluster, "Device out"=w2131:refnum<class "Channel.lvclass">)  [unwired: 7 in]
          n799 = Increment(x=w2126) -> (x+1=w2127:i32)
        }
        frame 263 {
          n800 = call-dynamic "Read resp.vi"("error in (no error)"=w2142, "Device in"=w2143) -> ("error out"=w2140:errorcluster, "resp"=w2135:string, "Device out"=w2138:refnum<class "Channel.lvclass">)  [unwired: 7 in]
          n801 = Fract/Exp String To Number(string=w2135) -> (number=w2133:dbl)  [unwired: 3 in, 1 out]
          n802 = Unbundle By Name(w2138) -> ("Interface.lvclass"=w2137:refnum<class "Interface.lvclass">)
          n803 = call "Read Camera Setup.vi"("Interface in"=w2137) -> ("Camera Setup"=w2136:T3)  [unwired: 8 in, 2 out]
          n804 = Unbundle By Name(w2136) -> ("VBIN"=w2132:u16)
          n805 = Equal?(x=w2132, y=w2133) -> (x = y?=w2134:bool)
          n806 = case shown="True" w2134 {
            tunnel: [w2144 w2145] -> w2141
            tunnel: w2139 -> [w2144 w2146]
            frame False {
            }
            frame True {
              n807 = Increment(x=w2146) -> (x+1=w2145:i32)
            }
          }
        }
        frame 264 {
          n808 = Unbundle By Name(w2155) -> ("Interface.lvclass"=w2154:refnum<class "Interface.lvclass">)
          n809 = call "Read Camera Setup.vi"("Interface in"=w2154) -> ("Camera Setup"=w2148:T3)  [unwired: 8 in, 2 out]
          n810 = Unbundle By Name(w2148) -> ("INITIAL_LINE"=w2147:u16)
          n811 = Number To Fractional String(number=w2147) -> (F-format string=w2149:string)  [unwired: 3 in]
          n812 = Concatenate Strings("SET INITIAL_LINE " ("cmd"), w2149) -> (w2153:string)
          n813 = call-dynamic "Write cmd.vi"("error in (no error)"=w2157, "cmd"=w2153, "Device in"=w2155) -> ("error out"=w2156:errorcluster, "Device out"=w2158:refnum<class "Channel.lvclass">)  [unwired: 7 in]
          n814 = Increment(x=w2151) -> (x+1=w2152:i32)
        }
        frame 265 {
          n815 = call-dynamic "Read resp.vi"("error in (no error)"=w2166, "Device in"=w2167) -> ("error out"=w2160:errorcluster, "resp"=w2165:string, "Device out"=w2161:refnum<class "Channel.lvclass">)  [unwired: 7 in]
          n816 = Equal?(x=w2165, y="DONE") -> (x = y?=w2163:bool)
          n817 = case shown="True" w2163 {
            tunnel: [w2168 w2169] -> w2162
            tunnel: w2159 -> [w2168 w2170]
            frame False {
            }
            frame True {
              n818 = Increment(x=w2170) -> (x+1=w2169:i32)
            }
          }
        }
        frame 266 {
          n819 = call-dynamic "Write cmd.vi"("error in (no error)"=w2176, "cmd"="GET INITIAL_LINE", "Device in"=w2174) -> ("error out"=w2175:errorcluster, "Device out"=w2177:refnum<class "Channel.lvclass">)  [unwired: 7 in]
          n820 = Increment(x=w2172) -> (x+1=w2173:i32)
        }
        frame 267 {
          n821 = call-dynamic "Read resp.vi"("error in (no error)"=w2188, "Device in"=w2189) -> ("error out"=w2186:errorcluster, "resp"=w2181:string, "Device out"=w2184:refnum<class "Channel.lvclass">)  [unwired: 7 in]
          n822 = Fract/Exp String To Number(string=w2181) -> (number=w2179:dbl)  [unwired: 3 in, 1 out]
          n823 = Unbundle By Name(w2184) -> ("Interface.lvclass"=w2183:refnum<class "Interface.lvclass">)
          n824 = call "Read Camera Setup.vi"("Interface in"=w2183) -> ("Camera Setup"=w2182:T3)  [unwired: 8 in, 2 out]
          n825 = Unbundle By Name(w2182) -> ("INITIAL_LINE"=w2178:u16)
          n826 = Equal?(x=w2178, y=w2179) -> (x = y?=w2180:bool)
          n827 = case shown="True" w2180 {
            tunnel: [w2190 w2191] -> w2187
            tunnel: w2185 -> [w2190 w2192]
            frame False {
            }
            frame True {
              n828 = Increment(x=w2192) -> (x+1=w2191:i32)
            }
          }
        }
        frame 268 {
          n829 = Unbundle By Name(w2201) -> ("Interface.lvclass"=w2200:refnum<class "Interface.lvclass">)
          n830 = call "Read Camera Setup.vi"("Interface in"=w2200) -> ("Camera Setup"=w2194:T3)  [unwired: 8 in, 2 out]
          n831 = Unbundle By Name(w2194) -> ("INITIAL_COLUMN"=w2193:u16)
          n832 = Number To Fractional String(number=w2193) -> (F-format string=w2195:string)  [unwired: 3 in]
          n833 = Concatenate Strings("SET INITIAL_COLUMN " ("cmd"), w2195) -> (w2199:string)
          n834 = call-dynamic "Write cmd.vi"("error in (no error)"=w2203, "cmd"=w2199, "Device in"=w2201) -> ("error out"=w2202:errorcluster, "Device out"=w2204:refnum<class "Channel.lvclass">)  [unwired: 7 in]
          n835 = Increment(x=w2197) -> (x+1=w2198:i32)
        }
        frame 269 {
          n836 = call-dynamic "Read resp.vi"("error in (no error)"=w2212, "Device in"=w2213) -> ("error out"=w2206:errorcluster, "resp"=w2211:string, "Device out"=w2207:refnum<class "Channel.lvclass">)  [unwired: 7 in]
          n837 = Equal?(x=w2211, y="DONE") -> (x = y?=w2209:bool)
          n838 = case shown="True" w2209 {
            tunnel: [w2214 w2215] -> w2208
            tunnel: w2205 -> [w2214 w2216]
            frame False {
            }
            frame True {
              n839 = Increment(x=w2216) -> (x+1=w2215:i32)
            }
          }
        }
        frame 270 {
          n840 = call-dynamic "Write cmd.vi"("error in (no error)"=w2222, "cmd"="GET INITIAL_COLUMN", "Device in"=w2220) -> ("error out"=w2221:errorcluster, "Device out"=w2223:refnum<class "Channel.lvclass">)  [unwired: 7 in]
          n841 = Increment(x=w2218) -> (x+1=w2219:i32)
        }
        frame 271 {
          n842 = call-dynamic "Read resp.vi"("error in (no error)"=w2234, "Device in"=w2235) -> ("error out"=w2232:errorcluster, "resp"=w2227:string, "Device out"=w2230:refnum<class "Channel.lvclass">)  [unwired: 7 in]
          n843 = Fract/Exp String To Number(string=w2227) -> (number=w2225:dbl)  [unwired: 3 in, 1 out]
          n844 = Unbundle By Name(w2230) -> ("Interface.lvclass"=w2229:refnum<class "Interface.lvclass">)
          n845 = call "Read Camera Setup.vi"("Interface in"=w2229) -> ("Camera Setup"=w2228:T3)  [unwired: 8 in, 2 out]
          n846 = Unbundle By Name(w2228) -> ("INITIAL_COLUMN"=w2224:u16)
          n847 = Equal?(x=w2224, y=w2225) -> (x = y?=w2226:bool)
          n848 = case shown="True" w2226 {
            tunnel: [w2236 w2237] -> w2233
            tunnel: w2231 -> [w2236 w2238]
            frame False {
            }
            frame True {
              n849 = Increment(x=w2238) -> (x+1=w2237:i32)
            }
          }
        }
        frame 272 {
          n850 = Unbundle By Name(w2247) -> ("Interface.lvclass"=w2246:refnum<class "Interface.lvclass">)
          n851 = call "Read Camera Setup.vi"("Interface in"=w2246) -> ("Camera Setup"=w2240:T3)  [unwired: 8 in, 2 out]
          n852 = Unbundle By Name(w2240) -> ("FINAL_LINE"=w2239:u16)
          n853 = Number To Fractional String(number=w2239) -> (F-format string=w2241:string)  [unwired: 3 in]
          n854 = Concatenate Strings("SET FINAL_LINE " ("cmd"), w2241) -> (w2245:string)
          n855 = call-dynamic "Write cmd.vi"("error in (no error)"=w2249, "cmd"=w2245, "Device in"=w2247) -> ("error out"=w2248:errorcluster, "Device out"=w2250:refnum<class "Channel.lvclass">)  [unwired: 7 in]
          n856 = Increment(x=w2243) -> (x+1=w2244:i32)
        }
        frame 273 {
          n857 = call-dynamic "Read resp.vi"("error in (no error)"=w2258, "Device in"=w2259) -> ("error out"=w2252:errorcluster, "resp"=w2257:string, "Device out"=w2253:refnum<class "Channel.lvclass">)  [unwired: 7 in]
          n858 = Equal?(x=w2257, y="DONE") -> (x = y?=w2255:bool)
          n859 = case shown="True" w2255 {
            tunnel: [w2260 w2261] -> w2254
            tunnel: w2251 -> [w2260 w2262]
            frame False {
            }
            frame True {
              n860 = Increment(x=w2262) -> (x+1=w2261:i32)
            }
          }
        }
        frame 274 {
          n861 = call-dynamic "Write cmd.vi"("error in (no error)"=w2268, "cmd"="GET FINAL_LINE", "Device in"=w2266) -> ("error out"=w2267:errorcluster, "Device out"=w2269:refnum<class "Channel.lvclass">)  [unwired: 7 in]
          n862 = Increment(x=w2264) -> (x+1=w2265:i32)
        }
        frame 275 {
          n863 = call-dynamic "Read resp.vi"("error in (no error)"=w2280, "Device in"=w2281) -> ("error out"=w2278:errorcluster, "resp"=w2273:string, "Device out"=w2276:refnum<class "Channel.lvclass">)  [unwired: 7 in]
          n864 = Fract/Exp String To Number(string=w2273) -> (number=w2271:dbl)  [unwired: 3 in, 1 out]
          n865 = Unbundle By Name(w2276) -> ("Interface.lvclass"=w2275:refnum<class "Interface.lvclass">)
          n866 = call "Read Camera Setup.vi"("Interface in"=w2275) -> ("Camera Setup"=w2274:T3)  [unwired: 8 in, 2 out]
          n867 = Unbundle By Name(w2274) -> ("FINAL_LINE"=w2270:u16)
          n868 = Equal?(x=w2270, y=w2271) -> (x = y?=w2272:bool)
          n869 = case shown="True" w2272 {
            tunnel: [w2282 w2283] -> w2279
            tunnel: w2277 -> [w2282 w2284]
            frame False {
            }
            frame True {
              n870 = Increment(x=w2284) -> (x+1=w2283:i32)
            }
          }
        }
        frame 276 {
          n871 = Unbundle By Name(w2293) -> ("Interface.lvclass"=w2292:refnum<class "Interface.lvclass">)
          n872 = call "Read Camera Setup.vi"("Interface in"=w2292) -> ("Camera Setup"=w2286:T3)  [unwired: 8 in, 2 out]
          n873 = Unbundle By Name(w2286) -> ("FINAL_COLUMN"=w2285:u16)
          n874 = Number To Fractional String(number=w2285) -> (F-format string=w2287:string)  [unwired: 3 in]
          n875 = Concatenate Strings("SET FINAL_COLUMN " ("cmd"), w2287) -> (w2291:string)
          n876 = call-dynamic "Write cmd.vi"("error in (no error)"=w2295, "cmd"=w2291, "Device in"=w2293) -> ("error out"=w2294:errorcluster, "Device out"=w2296:refnum<class "Channel.lvclass">)  [unwired: 7 in]
          n877 = Increment(x=w2289) -> (x+1=w2290:i32)
        }
        frame 277 {
          n878 = call-dynamic "Read resp.vi"("error in (no error)"=w2304, "Device in"=w2305) -> ("error out"=w2298:errorcluster, "resp"=w2303:string, "Device out"=w2299:refnum<class "Channel.lvclass">)  [unwired: 7 in]
          n879 = Equal?(x=w2303, y="DONE") -> (x = y?=w2301:bool)
          n880 = case shown="True" w2301 {
            tunnel: [w2306 w2307] -> w2300
            tunnel: w2297 -> [w2306 w2308]
            frame False {
            }
            frame True {
              n881 = Increment(x=w2308) -> (x+1=w2307:i32)
            }
          }
        }
        frame 278 {
          n882 = call-dynamic "Write cmd.vi"("error in (no error)"=w2314, "cmd"="GET FINAL_COLUMN", "Device in"=w2312) -> ("error out"=w2313:errorcluster, "Device out"=w2315:refnum<class "Channel.lvclass">)  [unwired: 7 in]
          n883 = Increment(x=w2310) -> (x+1=w2311:i32)
        }
        frame 279 {
          n884 = call-dynamic "Read resp.vi"("error in (no error)"=w2326, "Device in"=w2327) -> ("error out"=w2324:errorcluster, "resp"=w2319:string, "Device out"=w2322:refnum<class "Channel.lvclass">)  [unwired: 7 in]
          n885 = Fract/Exp String To Number(string=w2319) -> (number=w2317:dbl)  [unwired: 3 in, 1 out]
          n886 = Unbundle By Name(w2322) -> ("Interface.lvclass"=w2321:refnum<class "Interface.lvclass">)
          n887 = call "Read Camera Setup.vi"("Interface in"=w2321) -> ("Camera Setup"=w2320:T3)  [unwired: 8 in, 2 out]
          n888 = Unbundle By Name(w2320) -> ("FINAL_COLUMN"=w2316:u16)
          n889 = Equal?(x=w2316, y=w2317) -> (x = y?=w2318:bool)
          n890 = disable-structure shown="Enabled" {
            disable-tunnel: [w2330 0 ("State")] -> w2325
            disable-tunnel: w2323 -> [w2329 _]
            disable-tunnel: w2318 -> [w2328 _]
            frame Disabled {
              n891 = case shown="True" w2328 {
                tunnel: [w2331 w2332] -> w2330
                tunnel: w2329 -> [w2331 w2333]
                frame False {
                }
                frame True {
                  n892 = Increment(x=w2333) -> (x+1=w2332:i32)
                }
              }
            }
            frame Enabled {
            }
          }
        }
        frame 280 {
          n893 = Unbundle By Name(w2343) -> ("Interface.lvclass"=w2342:refnum<class "Interface.lvclass">)
          n894 = call "Read Camera Setup.vi"("Interface in"=w2342) -> ("Camera Setup"=w2336:T3)  [unwired: 8 in, 2 out]
          n895 = Unbundle By Name(w2336) -> ("VERTICAL_CLOCK_VOLTAGE"=w2335:u8)
          n896 = Number To Fractional String(number=w2335) -> (F-format string=w2337:string)  [unwired: 3 in]
          n897 = Concatenate Strings("SET VERTICAL_CLOCK_VOLTAGE " ("cmd"), w2337) -> (w2341:string)
          n898 = call-dynamic "Write cmd.vi"("error in (no error)"=w2345, "cmd"=w2341, "Device in"=w2343) -> ("error out"=w2344:errorcluster, "Device out"=w2346:refnum<class "Channel.lvclass">)  [unwired: 7 in]
          n899 = Increment(x=w2339) -> (x+1=w2340:i32)
        }
        frame 281 {
          n900 = call-dynamic "Read resp.vi"("error in (no error)"=w2354, "Device in"=w2355) -> ("error out"=w2348:errorcluster, "resp"=w2353:string, "Device out"=w2349:refnum<class "Channel.lvclass">)  [unwired: 7 in]
          n901 = Equal?(x=w2353, y="DONE") -> (x = y?=w2351:bool)
          n902 = case shown="True" w2351 {
            tunnel: [w2356 w2357] -> w2350
            tunnel: w2347 -> [w2356 w2358]
            frame False {
            }
            frame True {
              n903 = Increment(x=w2358) -> (x+1=w2357:i32)
            }
          }
        }
        frame 282 {
          n904 = call-dynamic "Write cmd.vi"("error in (no error)"=w2364, "cmd"="GET VERTICAL_CLOCK_VOLTAGE", "Device in"=w2362) -> ("error out"=w2363:errorcluster, "Device out"=w2365:refnum<class "Channel.lvclass">)  [unwired: 7 in]
          n905 = Increment(x=w2360) -> (x+1=w2361:i32)
        }
        frame 283 {
          n906 = call-dynamic "Read resp.vi"("error in (no error)"=w2376, "Device in"=w2377) -> ("error out"=w2374:errorcluster, "resp"=w2369:string, "Device out"=w2372:refnum<class "Channel.lvclass">)  [unwired: 7 in]
          n907 = Fract/Exp String To Number(string=w2369) -> (number=w2367:dbl)  [unwired: 3 in, 1 out]
          n908 = Unbundle By Name(w2372) -> ("Interface.lvclass"=w2371:refnum<class "Interface.lvclass">)
          n909 = call "Read Camera Setup.vi"("Interface in"=w2371) -> ("Camera Setup"=w2370:T3)  [unwired: 8 in, 2 out]
          n910 = Unbundle By Name(w2370) -> ("VERTICAL_CLOCK_VOLTAGE"=w2366:u8)
          n911 = Equal?(x=w2366, y=w2367) -> (x = y?=w2368:bool)
          n912 = case shown="True" w2368 {
            tunnel: [w2378 w2379] -> w2375
            tunnel: w2373 -> [w2378 w2380]
            frame False {
            }
            frame True {
              n913 = Increment(x=w2380) -> (x+1=w2379:i32)
            }
          }
        }
        frame 284 {
          n914 = Unbundle By Name(w2389) -> ("Interface.lvclass"=w2388:refnum<class "Interface.lvclass">)
          n915 = call "Read Camera Setup.vi"("Interface in"=w2388) -> ("Camera Setup"=w2383:T3)  [unwired: 8 in, 2 out]
          n916 = Unbundle By Name(w2383) -> ("FRAME_TRANSFER"=w2382:bool)
          n917 = case shown="True" w2382 {
            tunnel: ["T" ("cmd") "F" ("cmd")] -> w2381
            frame True {
            }
            frame False {
            }
          }
          n918 = Concatenate Strings("SET FRAME_TRANSFER " ("cmd"), w2381) -> (w2387:string)
          n919 = call-dynamic "Write cmd.vi"("error in (no error)"=w2391, "cmd"=w2387, "Device in"=w2389) -> ("error out"=w2390:errorcluster, "Device out"=w2392:refnum<class "Channel.lvclass">)  [unwired: 7 in]
          n920 = Increment(x=w2385) -> (x+1=w2386:i32)
        }
        frame 285 {
          n921 = call-dynamic "Read resp.vi"("error in (no error)"=w2402, "Device in"=w2403) -> ("error out"=w2396:errorcluster, "resp"=w2401:string, "Device out"=w2397:refnum<class "Channel.lvclass">)  [unwired: 7 in]
          n922 = Equal?(x=w2401, y="DONE") -> (x = y?=w2399:bool)
          n923 = case shown="True" w2399 {
            tunnel: [w2404 w2405] -> w2398
            tunnel: w2395 -> [w2404 w2406]
            frame False {
            }
            frame True {
              n924 = Increment(x=w2406) -> (x+1=w2405:i32)
            }
          }
        }
        frame 286 {
          n925 = call-dynamic "Write cmd.vi"("error in (no error)"=w2412, "cmd"="GET FRAME_TRANSFER", "Device in"=w2410) -> ("error out"=w2411:errorcluster, "Device out"=w2413:refnum<class "Channel.lvclass">)  [unwired: 7 in]
          n926 = Increment(x=w2408) -> (x+1=w2409:i32)
        }
        frame 287 {
          n927 = call-dynamic "Read resp.vi"("error in (no error)"=w2424, "Device in"=w2425) -> ("error out"=w2422:errorcluster, "resp"=w2416:string, "Device out"=w2420:refnum<class "Channel.lvclass">)  [unwired: 7 in]
          n928 = Unbundle By Name(w2420) -> ("Interface.lvclass"=w2419:refnum<class "Interface.lvclass">)
          n929 = call "Read Camera Setup.vi"("Interface in"=w2419) -> ("Camera Setup"=w2418:T3)  [unwired: 8 in, 2 out]
          n930 = Unbundle By Name(w2418) -> ("FRAME_TRANSFER"=w2415:bool)
          n931 = case shown="True" w2415 {
            tunnel: ["T" "F"] -> w2414
            frame True {
            }
            frame False {
            }
          }
          n932 = Equal?(x=w2414, y=w2416) -> (x = y?=w2417:bool)
          n933 = case shown="True" w2417 {
            tunnel: [w2428 w2429] -> w2423
            tunnel: w2421 -> [w2428 w2430]
            frame False {
            }
            frame True {
              n934 = Increment(x=w2430) -> (x+1=w2429:i32)
            }
          }
        }
        frame 288 {
          n935 = Unbundle By Name(w2439) -> ("Interface.lvclass"=w2438:refnum<class "Interface.lvclass">)
          n936 = call "Read Camera Setup.vi"("Interface in"=w2438) -> ("Camera Setup"=w2432:T3)  [unwired: 8 in, 2 out]
          n937 = Unbundle By Name(w2432) -> ("AD_CHANNEL"=w2431:u32)
          n938 = Number To Fractional String(number=w2431) -> (F-format string=w2433:string)  [unwired: 3 in]
          n939 = Concatenate Strings("SET AD_CHANNEL " ("cmd"), w2433) -> (w2437:string)
          n940 = call-dynamic "Write cmd.vi"("error in (no error)"=w2441, "cmd"=w2437, "Device in"=w2439) -> ("error out"=w2440:errorcluster, "Device out"=w2442:refnum<class "Channel.lvclass">)  [unwired: 7 in]
          n941 = Increment(x=w2435) -> (x+1=w2436:i32)
        }
        frame 289 {
          n942 = call-dynamic "Read resp.vi"("error in (no error)"=w2450, "Device in"=w2451) -> ("error out"=w2444:errorcluster, "resp"=w2449:string, "Device out"=w2445:refnum<class "Channel.lvclass">)  [unwired: 7 in]
          n943 = Equal?(x=w2449, y="DONE") -> (x = y?=w2447:bool)
          n944 = case shown="True" w2447 {
            tunnel: [w2452 w2453] -> w2446
            tunnel: w2443 -> [w2452 w2454]
            frame False {
            }
            frame True {
              n945 = Increment(x=w2454) -> (x+1=w2453:i32)
            }
          }
        }
        frame 290 {
          n946 = call-dynamic "Write cmd.vi"("error in (no error)"=w2460, "cmd"="GET AD_CHANNEL", "Device in"=w2458) -> ("error out"=w2459:errorcluster, "Device out"=w2461:refnum<class "Channel.lvclass">)  [unwired: 7 in]
          n947 = Increment(x=w2456) -> (x+1=w2457:i32)
        }
        frame 291 {
          n948 = call-dynamic "Read resp.vi"("error in (no error)"=w2472, "Device in"=w2473) -> ("error out"=w2470:errorcluster, "resp"=w2465:string, "Device out"=w2468:refnum<class "Channel.lvclass">)  [unwired: 7 in]
          n949 = Fract/Exp String To Number(string=w2465) -> (number=w2463:dbl)  [unwired: 3 in, 1 out]
          n950 = Unbundle By Name(w2468) -> ("Interface.lvclass"=w2467:refnum<class "Interface.lvclass">)
          n951 = call "Read Camera Setup.vi"("Interface in"=w2467) -> ("Camera Setup"=w2466:T3)  [unwired: 8 in, 2 out]
          n952 = Unbundle By Name(w2466) -> ("AD_CHANNEL"=w2462:u32)
          n953 = Equal?(x=w2462, y=w2463) -> (x = y?=w2464:bool)
          n954 = case shown="True" w2464 {
            tunnel: [w2474 w2475] -> w2471
            tunnel: w2469 -> [w2474 w2476]
            frame False {
            }
            frame True {
              n955 = Increment(x=w2476) -> (x+1=w2475:i32)
            }
          }
        }
        frame 300 {
          # "suffix"
          n956 = call-dynamic "Write Timer.vi"("error in (no error)"=w2479, "Timer"=u32 50, "State Machine in"=w2483) -> ("error out"=w2484:errorcluster, "State Machine out"=w2477:refnum<class "State Machine.lvclass">)  [unwired: 7 in]
          n957 = call-dynamic "Write State Machine.vi"("error in (no error)"=w2484, "State Machine.lvclass"=w2477, "Device in"=w2481) -> ("error out"=w2478:errorcluster, "Device out"=w2480:refnum<class "Channel.lvclass">)  [unwired: 7 in]
          n958 = Unbundle By Name(w2480) -> ("Interface.lvclass"=w2490:refnum<class "Interface.lvclass">)
          n959 = call-dynamic "Read Suffix.vi"("Interface in"=w2490) -> ("Suffix"=w2485:string)  [unwired: 8 in, 2 out]
          n960 = Concatenate Strings("SET SUFFIX " ("cmd"), w2485) -> (w2489:string)
          n961 = call-dynamic "Write cmd.vi"("error in (no error)"=w2478, "cmd"=w2489, "Device in"=w2480) -> ("error out"=w2491:errorcluster, "Device out"=w2492:refnum<class "Channel.lvclass">)  [unwired: 7 in]
          n962 = Increment(x=w2487) -> (x+1=w2488:i32)
        }
        frame 301 {
          n963 = call "Verify Timer.vi"("error in (no error)"=w2500, "State Machine in"=w2501) -> ("error out"=w2497:errorcluster, "timeout"=w2494:bool, "State Machine out"=w2498:refnum<class "State Machine.lvclass">)  [unwired: 7 in]
          n964 = call-dynamic "Write State Machine.vi"("error in (no error)"=w2497, "State Machine.lvclass"=w2498, "Device in"=w2499) -> ("error out"=w2496:errorcluster, "Device out"=w2495:refnum<class "Channel.lvclass">)  [unwired: 7 in]
          n965 = call-dynamic "Read resp.vi"("error in (no error)"=w2496, "Device in"=w2495) -> ("error out"=w2503:errorcluster, "resp"=w2507:string, "Device out"=w2504:refnum<class "Channel.lvclass">)  [unwired: 7 in]
          n966 = Equal?(x=w2507, y="DONE") -> (x = y?=w2493:bool)
          n967 = case shown="False" w2494 {
            tunnel: [w2509 0] -> w2505
            tunnel: w2502 -> [w2510 _]
            tunnel: w2493 -> [w2508 _]
            frame False {
              n968 = case shown="True" w2508 {
                tunnel: w2510 -> [w2511 w2513]
                tunnel: [w2511 w2512] -> w2509
                frame False {
                }
                frame True {
                  n969 = Increment(x=w2513) -> (x+1=w2512:i32)
                }
              }
            }
            frame True {
            }
          }
        }
        frame 302 {
          # "obstype"
          n970 = call-dynamic "Write Timer.vi"("error in (no error)"=w2518, "Timer"=u32 50, "State Machine in"=w2515) -> ("error out"=w2523:errorcluster, "State Machine out"=w2521:refnum<class "State Machine.lvclass">)  [unwired: 7 in]
          n971 = call-dynamic "Write State Machine.vi"("error in (no error)"=w2523, "State Machine.lvclass"=w2521, "Device in"=w2520) -> ("error out"=w2517:errorcluster, "Device out"=w2519:refnum<class "Channel.lvclass">)  [unwired: 7 in]
          n972 = Unbundle By Name(w2519) -> ("Interface.lvclass"=w2529:refnum<class "Interface.lvclass">)
          n973 = call-dynamic "Read ObsType.vi"("error in (no error)"=w2517, "Interface in"=w2529) -> ("error out"=w2516:errorcluster, "ObsType"=w2524:string)  [unwired: 7 in, 1 out]
          n974 = Concatenate Strings("SET OBSTYPE " ("cmd"), w2524) -> (w2528:string)
          n975 = call-dynamic "Write cmd.vi"("error in (no error)"=w2516, "cmd"=w2528, "Device in"=w2519) -> ("error out"=w2530:errorcluster, "Device out"=w2531:refnum<class "Channel.lvclass">)  [unwired: 7 in]
          n976 = Increment(x=w2526) -> (x+1=w2527:i32)
        }
        frame 303 {
          n977 = call "Verify Timer.vi"("error in (no error)"=w2540, "State Machine in"=w2538) -> ("error out"=w2539:errorcluster, "timeout"=w2535:bool, "State Machine out"=w2542:refnum<class "State Machine.lvclass">)  [unwired: 7 in]
          n978 = call-dynamic "Write State Machine.vi"("error in (no error)"=w2539, "State Machine.lvclass"=w2542, "Device in"=w2541) -> ("error out"=w2536:errorcluster, "Device out"=w2537:refnum<class "Channel.lvclass">)  [unwired: 7 in]
          n979 = call-dynamic "Read resp.vi"("error in (no error)"=w2536, "Device in"=w2537) -> ("error out"=w2543:errorcluster, "resp"=w2546:string, "Device out"=w2544:refnum<class "Channel.lvclass">)  [unwired: 7 in]
          n980 = Equal?(x=w2546, y="DONE") -> (x = y?=w2533:bool)
          n981 = case shown="False" w2535 {
            tunnel: [w2548 0] -> w2532
            tunnel: w2534 -> [w2549 _]
            tunnel: w2533 -> [w2547 _]
            frame False {
              n982 = case shown="True" w2547 {
                tunnel: w2549 -> [w2550 w2552]
                tunnel: [w2550 w2551] -> w2548
                frame False {
                }
                frame True {
                  n983 = Increment(x=w2552) -> (x+1=w2551:i32)
                }
              }
            }
            frame True {
            }
          }
        }
        frame 304 {
          # "observer"
          n984 = call-dynamic "Write Timer.vi"("error in (no error)"=w2558, "Timer"=u32 50, "State Machine in"=w2554) -> ("error out"=w2563:errorcluster, "State Machine out"=w2561:refnum<class "State Machine.lvclass">)  [unwired: 7 in]
          n985 = call-dynamic "Write State Machine.vi"("error in (no error)"=w2563, "State Machine.lvclass"=w2561, "Device in"=w2560) -> ("error out"=w2557:errorcluster, "Device out"=w2559:refnum<class "Channel.lvclass">)  [unwired: 7 in]
          n986 = Unbundle By Name(w2559) -> ("Interface.lvclass"=w2568:refnum<class "Interface.lvclass">)
          n987 = call-dynamic "Read Observer.vi"("error in (no error)"=w2557, "Interface in"=w2568) -> ("error out"=w2556:errorcluster, "Observer"=w2564:string)  [unwired: 7 in, 1 out]
          n988 = Concatenate Strings("SET OBSERVER " ("cmd"), w2564) -> (w2567:string)
          n989 = call-dynamic "Write cmd.vi"("error in (no error)"=w2556, "cmd"=w2567, "Device in"=w2559) -> ("error out"=w2569:errorcluster, "Device out"=w2570:refnum<class "Channel.lvclass">)  [unwired: 7 in]
          n990 = Increment(x=w2565) -> (x+1=w2566:i32)
        }
        frame 305 {
          n991 = call "Verify Timer.vi"("error in (no error)"=w2579, "State Machine in"=w2577) -> ("error out"=w2578:errorcluster, "timeout"=w2574:bool, "State Machine out"=w2581:refnum<class "State Machine.lvclass">)  [unwired: 7 in]
          n992 = call-dynamic "Write State Machine.vi"("error in (no error)"=w2578, "State Machine.lvclass"=w2581, "Device in"=w2580) -> ("error out"=w2575:errorcluster, "Device out"=w2576:refnum<class "Channel.lvclass">)  [unwired: 7 in]
          n993 = call-dynamic "Read resp.vi"("error in (no error)"=w2575, "Device in"=w2576) -> ("error out"=w2582:errorcluster, "resp"=w2585:string, "Device out"=w2583:refnum<class "Channel.lvclass">)  [unwired: 7 in]
          n994 = Equal?(x=w2585, y="DONE") -> (x = y?=w2572:bool)
          n995 = case shown="False" w2574 {
            tunnel: [w2587 0] -> w2571
            tunnel: w2573 -> [w2588 _]
            tunnel: w2572 -> [w2586 _]
            frame False {
              n996 = case shown="True" w2586 {
                tunnel: w2588 -> [w2589 w2591]
                tunnel: [w2589 w2590] -> w2587
                frame False {
                }
                frame True {
                  n997 = Increment(x=w2591) -> (x+1=w2590:i32)
                }
              }
            }
            frame True {
            }
          }
        }
        frame 306 {
          # "comment"
          n998 = call-dynamic "Write Timer.vi"("error in (no error)"=w2597, "Timer"=u32 50, "State Machine in"=w2593) -> ("error out"=w2602:errorcluster, "State Machine out"=w2600:refnum<class "State Machine.lvclass">)  [unwired: 7 in]
          n999 = call-dynamic "Write State Machine.vi"("error in (no error)"=w2602, "State Machine.lvclass"=w2600, "Device in"=w2599) -> ("error out"=w2596:errorcluster, "Device out"=w2598:refnum<class "Channel.lvclass">)  [unwired: 7 in]
          n1000 = Unbundle By Name(w2598) -> ("Interface.lvclass"=w2607:refnum<class "Interface.lvclass">)
          n1001 = call-dynamic "Read Comments.vi"("error in (no error)"=w2596, "Interface in"=w2607) -> ("error out"=w2595:errorcluster, "Comments"=w2603:string)  [unwired: 7 in, 1 out]
          n1002 = Concatenate Strings("SET COMMENT " ("cmd"), w2603) -> (w2606:string)
          n1003 = call-dynamic "Write cmd.vi"("error in (no error)"=w2595, "cmd"=w2606, "Device in"=w2598) -> ("error out"=w2608:errorcluster, "Device out"=w2609:refnum<class "Channel.lvclass">)  [unwired: 7 in]
          n1004 = Increment(x=w2604) -> (x+1=w2605:i32)
        }
        frame 307 {
          n1005 = call "Verify Timer.vi"("error in (no error)"=w2618, "State Machine in"=w2616) -> ("error out"=w2617:errorcluster, "timeout"=w2613:bool, "State Machine out"=w2620:refnum<class "State Machine.lvclass">)  [unwired: 7 in]
          n1006 = call-dynamic "Write State Machine.vi"("error in (no error)"=w2617, "State Machine.lvclass"=w2620, "Device in"=w2619) -> ("error out"=w2614:errorcluster, "Device out"=w2615:refnum<class "Channel.lvclass">)  [unwired: 7 in]
          n1007 = call-dynamic "Read resp.vi"("error in (no error)"=w2614, "Device in"=w2615) -> ("error out"=w2621:errorcluster, "resp"=w2624:string, "Device out"=w2622:refnum<class "Channel.lvclass">)  [unwired: 7 in]
          n1008 = Equal?(x=w2624, y="DONE") -> (x = y?=w2611:bool)
          n1009 = case shown="False" w2613 {
            tunnel: [w2626 0] -> w2610
            tunnel: w2612 -> [w2627 _]
            tunnel: w2611 -> [w2625 _]
            frame False {
              n1010 = case shown="True" w2625 {
                tunnel: w2627 -> [w2628 w2630]
                tunnel: [w2628 w2629] -> w2626
                frame False {
                }
                frame True {
                  n1011 = Increment(x=w2630) -> (x+1=w2629:i32)
                }
              }
            }
            frame True {
            }
          }
        }
        frame 308 {
          # "object"
          n1012 = call-dynamic "Write Timer.vi"("error in (no error)"=w2636, "Timer"=u32 50, "State Machine in"=w2632) -> ("error out"=w2641:errorcluster, "State Machine out"=w2639:refnum<class "State Machine.lvclass">)  [unwired: 7 in]
          n1013 = call-dynamic "Write State Machine.vi"("error in (no error)"=w2641, "State Machine.lvclass"=w2639, "Device in"=w2638) -> ("error out"=w2635:errorcluster, "Device out"=w2637:refnum<class "Channel.lvclass">)  [unwired: 7 in]
          n1014 = Unbundle By Name(w2637) -> ("Interface.lvclass"=w2646:refnum<class "Interface.lvclass">)
          n1015 = call-dynamic "Read Object.vi"("error in (no error)"=w2635, "Interface in"=w2646) -> ("error out"=w2634:errorcluster, "Object"=w2642:string)  [unwired: 7 in, 1 out]
          n1016 = Concatenate Strings("SET OBJECT " ("cmd"), w2642) -> (w2645:string)
          n1017 = call-dynamic "Write cmd.vi"("error in (no error)"=w2634, "cmd"=w2645, "Device in"=w2637) -> ("error out"=w2647:errorcluster, "Device out"=w2648:refnum<class "Channel.lvclass">)  [unwired: 7 in]
          n1018 = Increment(x=w2643) -> (x+1=w2644:i32)
        }
        frame 309 {
          n1019 = call "Verify Timer.vi"("error in (no error)"=w2657, "State Machine in"=w2655) -> ("error out"=w2656:errorcluster, "timeout"=w2652:bool, "State Machine out"=w2659:refnum<class "State Machine.lvclass">)  [unwired: 7 in]
          n1020 = call-dynamic "Write State Machine.vi"("error in (no error)"=w2656, "State Machine.lvclass"=w2659, "Device in"=w2658) -> ("error out"=w2653:errorcluster, "Device out"=w2654:refnum<class "Channel.lvclass">)  [unwired: 7 in]
          n1021 = call-dynamic "Read resp.vi"("error in (no error)"=w2653, "Device in"=w2654) -> ("error out"=w2660:errorcluster, "resp"=w2663:string, "Device out"=w2661:refnum<class "Channel.lvclass">)  [unwired: 7 in]
          n1022 = Equal?(x=w2663, y="DONE") -> (x = y?=w2650:bool)
          n1023 = case shown="False" w2652 {
            tunnel: [w2665 0] -> w2649
            tunnel: w2651 -> [w2666 _]
            tunnel: w2650 -> [w2664 _]
            frame False {
              n1024 = case shown="True" w2664 {
                tunnel: w2666 -> [w2667 w2669]
                tunnel: [w2667 w2668] -> w2665
                frame False {
                }
                frame True {
                  n1025 = Increment(x=w2669) -> (x+1=w2668:i32)
                }
              }
            }
            frame True {
            }
          }
        }
        frame 310 {
          # "project id"
          n1026 = call-dynamic "Write Timer.vi"("error in (no error)"=w2675, "Timer"=u32 50, "State Machine in"=w2671) -> ("error out"=w2680:errorcluster, "State Machine out"=w2678:refnum<class "State Machine.lvclass">)  [unwired: 7 in]
          n1027 = call-dynamic "Write State Machine.vi"("error in (no error)"=w2680, "State Machine.lvclass"=w2678, "Device in"=w2677) -> ("error out"=w2674:errorcluster, "Device out"=w2676:refnum<class "Channel.lvclass">)  [unwired: 7 in]
          n1028 = Unbundle By Name(w2676) -> ("Interface.lvclass"=w2685:refnum<class "Interface.lvclass">)
          n1029 = call-dynamic "Read Project ID.vi"("error in (no error)"=w2674, "Interface in"=w2685) -> ("error out"=w2673:errorcluster, "Project ID"=w2681:string)  [unwired: 7 in, 1 out]
          n1030 = Concatenate Strings("SET PROJECTID " ("cmd"), w2681) -> (w2684:string)
          n1031 = call-dynamic "Write cmd.vi"("error in (no error)"=w2673, "cmd"=w2684, "Device in"=w2676) -> ("error out"=w2686:errorcluster, "Device out"=w2687:refnum<class "Channel.lvclass">)  [unwired: 7 in]
          n1032 = Increment(x=w2682) -> (x+1=w2683:i32)
        }
        frame 311 {
          n1033 = call "Verify Timer.vi"("error in (no error)"=w2696, "State Machine in"=w2694) -> ("error out"=w2695:errorcluster, "timeout"=w2691:bool, "State Machine out"=w2698:refnum<class "State Machine.lvclass">)  [unwired: 7 in]
          n1034 = call-dynamic "Write State Machine.vi"("error in (no error)"=w2695, "State Machine.lvclass"=w2698, "Device in"=w2697) -> ("error out"=w2692:errorcluster, "Device out"=w2693:refnum<class "Channel.lvclass">)  [unwired: 7 in]
          n1035 = call-dynamic "Read resp.vi"("error in (no error)"=w2692, "Device in"=w2693) -> ("error out"=w2699:errorcluster, "resp"=w2702:string, "Device out"=w2700:refnum<class "Channel.lvclass">)  [unwired: 7 in]
          n1036 = Equal?(x=w2702, y="DONE") -> (x = y?=w2689:bool)
          n1037 = case shown="True" w2691 {
            tunnel: [w2704 w2710] -> w2688
            tunnel: w2690 -> [w2705 w2709]
            tunnel: w2689 -> [w2703 _]
            frame False {
              n1038 = case shown="True" w2703 {
                tunnel: w2705 -> [w2706 w2708]
                tunnel: [w2706 w2707] -> w2704
                frame False {
                }
                frame True {
                  n1039 = Increment(x=w2708) -> (x+1=w2707:i32)
                }
              }
            }
            frame True {
              # "Por enquanto, prossegue\nmesmo sem receber DONE."
              n1040 = disable-structure shown="Enabled" {
                disable-tunnel: [0 w2712] -> w2710
                disable-tunnel: w2709 -> [_ w2713]
                frame Disabled {
                }
                frame Enabled {
                  n1041 = Increment(x=w2713) -> (x+1=w2712:i32)
                }
              }
            }
          }
        }
        frame 312 {
          # "filter"
          n1042 = call-dynamic "Write Timer.vi"("error in (no error)"=w2719, "Timer"=u32 50, "State Machine in"=w2717) -> ("error out"=w2724:errorcluster, "State Machine out"=w2722:refnum<class "State Machine.lvclass">)  [unwired: 7 in]
          n1043 = call-dynamic "Write State Machine.vi"("error in (no error)"=w2724, "State Machine.lvclass"=w2722, "Device in"=w2721) -> ("error out"=w2714:errorcluster, "Device out"=w2720:refnum<class "Channel.lvclass">)  [unwired: 7 in]
          n1044 = Unbundle By Name(w2720) -> ("Filter"=w2716:u8)
          n1045 = case shown="0, Default" w2716 {
            tunnel: ["U" ("cmd") "B" ("cmd") "V" ("cmd") "R" ("cmd") "I" ("cmd") "CLEAR" ("cmd")] -> w2715
            frame 1 {
            }
            frame 2 {
            }
            frame 3 {
            }
            frame 4 {
            }
            frame 5 {
            }
            frame 0, Default {
            }
          }
          n1046 = Concatenate Strings("SET FILTER " ("cmd"), w2715) -> (w2727:string)
          n1047 = call-dynamic "Write cmd.vi"("error in (no error)"=w2714, "cmd"=w2727, "Device in"=w2720) -> ("error out"=w2728:errorcluster, "Device out"=w2729:refnum<class "Channel.lvclass">)  [unwired: 7 in]
          n1048 = Increment(x=w2725) -> (x+1=w2726:i32)
        }
        frame 313 {
          n1049 = call "Verify Timer.vi"("error in (no error)"=w2744, "State Machine in"=w2742) -> ("error out"=w2743:errorcluster, "timeout"=w2739:bool, "State Machine out"=w2746:refnum<class "State Machine.lvclass">)  [unwired: 7 in]
          n1050 = call-dynamic "Write State Machine.vi"("error in (no error)"=w2743, "State Machine.lvclass"=w2746, "Device in"=w2745) -> ("error out"=w2740:errorcluster, "Device out"=w2741:refnum<class "Channel.lvclass">)  [unwired: 7 in]
          n1051 = call-dynamic "Read resp.vi"("error in (no error)"=w2740, "Device in"=w2741) -> ("error out"=w2747:errorcluster, "resp"=w2750:string, "Device out"=w2748:refnum<class "Channel.lvclass">)  [unwired: 7 in]
          n1052 = Equal?(x=w2750, y="DONE") -> (x = y?=w2737:bool)
          n1053 = case shown="False" w2739 {
            tunnel: [w2752 0] -> w2736
            tunnel: w2738 -> [w2753 _]
            tunnel: w2737 -> [w2751 _]
            frame False {
              n1054 = case shown="True" w2751 {
                tunnel: w2753 -> [w2754 w2756]
                tunnel: [w2754 w2755] -> w2752
                frame False {
                }
                frame True {
                  n1055 = Increment(x=w2756) -> (x+1=w2755:i32)
                }
              }
            }
            frame True {
            }
          }
        }
        frame 314 {
          n1056 = call-dynamic "Write Timer.vi"("error in (no error)"=w2761, "Timer"=u32 50, "State Machine in"=w2760) -> ("error out"=w2766:errorcluster, "State Machine out"=w2764:refnum<class "State Machine.lvclass">)  [unwired: 7 in]
          n1057 = call-dynamic "Write State Machine.vi"("error in (no error)"=w2766, "State Machine.lvclass"=w2764, "Device in"=w2763) -> ("error out"=w2759:errorcluster, "Device out"=w2762:refnum<class "Channel.lvclass">)  [unwired: 7 in]
          n1058 = call-dynamic "Write cmd.vi"("error in (no error)"=w2759, "cmd"="SET CTRLINTE S4GUI", "Device in"=w2762) -> ("error out"=w2769:errorcluster, "Device out"=w2770:refnum<class "Channel.lvclass">)  [unwired: 7 in]
          n1059 = Increment(x=w2767) -> (x+1=w2768:i32)
        }
        frame 315 {
          n1060 = call "Verify Timer.vi"("error in (no error)"=w2779, "State Machine in"=w2777) -> ("error out"=w2778:errorcluster, "timeout"=w2774:bool, "State Machine out"=w2781:refnum<class "State Machine.lvclass">)  [unwired: 7 in]
          n1061 = call-dynamic "Write State Machine.vi"("error in (no error)"=w2778, "State Machine.lvclass"=w2781, "Device in"=w2780) -> ("error out"=w2775:errorcluster, "Device out"=w2776:refnum<class "Channel.lvclass">)  [unwired: 7 in]
          n1062 = call-dynamic "Read resp.vi"("error in (no error)"=w2775, "Device in"=w2776) -> ("error out"=w2782:errorcluster, "resp"=w2785:string, "Device out"=w2783:refnum<class "Channel.lvclass">)  [unwired: 7 in]
          n1063 = Equal?(x=w2785, y="DONE") -> (x = y?=w2772:bool)
          n1064 = case shown="False" w2774 {
            tunnel: [w2787 0] -> w2771
            tunnel: w2773 -> [w2788 _]
            tunnel: w2772 -> [w2786 _]
            frame False {
              n1065 = case shown="True" w2786 {
                tunnel: w2788 -> [w2789 w2791]
                tunnel: [w2789 w2790] -> w2787
                frame False {
                }
                frame True {
                  n1066 = Increment(x=w2791) -> (x+1=w2790:i32)
                }
              }
            }
            frame True {
            }
          }
        }
        frame 316 {
          # "Carrega timeout de 50 ciclos\npara resposta do ACS"
          n1067 = call-dynamic "Write Timer.vi"("error in (no error)"=w2801, "Timer"=u32 50, "State Machine in"=w2800) -> ("error out"=w2803:errorcluster, "State Machine out"=w2805:refnum<class "State Machine.lvclass">)  [unwired: 7 in]
          n1068 = call-dynamic "Write State Machine.vi"("error in (no error)"=w2803, "State Machine.lvclass"=w2805, "Device in"=w2802) -> ("error out"=w2795:errorcluster, "Device out"=w2794:refnum<class "Channel.lvclass">)  [unwired: 7 in]
          n1069 = Unbundle By Name(w2794) -> ("rotator"=w2793:dbl)
          n1070 = Number To Fractional String(number=w2793) -> (F-format string=w2797:string)  [unwired: 3 in]
          n1071 = Concatenate Strings("SET INSTROT " ("cmd"), w2797) -> (w2796:string)
          n1072 = call-dynamic "Write cmd.vi"("error in (no error)"=w2795, "cmd"=w2796, "Device in"=w2794) -> ("error out"=w2807:errorcluster, "Device out"=w2808:refnum<class "Channel.lvclass">)  [unwired: 7 in]
          n1073 = Increment(x=w2799) -> (x+1=w2806:i32)
        }
        frame 317 {
          n1074 = call "Verify Timer.vi"("error in (no error)"=w2813, "State Machine in"=w2814) -> ("error out"=w2818:errorcluster, "timeout"=w2810:bool, "State Machine out"=w2819:refnum<class "State Machine.lvclass">)  [unwired: 7 in]
          n1075 = call-dynamic "Write State Machine.vi"("error in (no error)"=w2818, "State Machine.lvclass"=w2819, "Device in"=w2817) -> ("error out"=w2815:errorcluster, "Device out"=w2816:refnum<class "Channel.lvclass">)  [unwired: 7 in]
          n1076 = call-dynamic "Read resp.vi"("error in (no error)"=w2815, "Device in"=w2816) -> ("error out"=w2820:errorcluster, "resp"=w2823:string, "Device out"=w2821:refnum<class "Channel.lvclass">)  [unwired: 7 in]
          n1077 = Equal?(x=w2823, y="DONE") -> (x = y?=w2809:bool)
          n1078 = case shown="False" w2810 {
            tunnel: [w2825 0] -> w2812
            tunnel: w2811 -> [w2826 _]
            tunnel: w2809 -> [w2824 _]
            frame False {
              n1079 = case shown="True" w2824 {
                tunnel: [w2827 w2828] -> w2825
                tunnel: w2826 -> [w2827 w2829]
                frame False {
                }
                frame True {
                  n1080 = Increment(x=w2829) -> (x+1=w2828:i32)
                }
              }
            }
            frame True {
            }
          }
        }
        frame 318 {
          # "Carrega timeout de 50 ciclos\npara resposta do ACS"
          n1081 = call-dynamic "Write Timer.vi"("error in (no error)"=w2838, "Timer"=u32 50, "State Machine in"=w2837) -> ("error out"=w2840:errorcluster, "State Machine out"=w2842:refnum<class "State Machine.lvclass">)  [unwired: 7 in]
          n1082 = call-dynamic "Write State Machine.vi"("error in (no error)"=w2840, "State Machine.lvclass"=w2842, "Device in"=w2839) -> ("error out"=w2833:errorcluster, "Device out"=w2832:refnum<class "Channel.lvclass">)  [unwired: 7 in]
          n1083 = Unbundle By Name(w2832) -> ("TCS mode"=w2831:string)
          n1084 = Concatenate Strings("SET TCSMODE " ("cmd"), w2831) -> (w2834:string)
          n1085 = call-dynamic "Write cmd.vi"("error in (no error)"=w2833, "cmd"=w2834, "Device in"=w2832) -> ("error out"=w2844:errorcluster, "Device out"=w2845:refnum<class "Channel.lvclass">)  [unwired: 7 in]
          n1086 = Increment(x=w2836) -> (x+1=w2843:i32)
        }
        frame 319 {
          n1087 = call "Verify Timer.vi"("error in (no error)"=w2850, "State Machine in"=w2851) -> ("error out"=w2855:errorcluster, "timeout"=w2847:bool, "State Machine out"=w2856:refnum<class "State Machine.lvclass">)  [unwired: 7 in]
          n1088 = call-dynamic "Write State Machine.vi"("error in (no error)"=w2855, "State Machine.lvclass"=w2856, "Device in"=w2854) -> ("error out"=w2852:errorcluster, "Device out"=w2853:refnum<class "Channel.lvclass">)  [unwired: 7 in]
          n1089 = call-dynamic "Read resp.vi"("error in (no error)"=w2852, "Device in"=w2853) -> ("error out"=w2857:errorcluster, "resp"=w2860:string, "Device out"=w2858:refnum<class "Channel.lvclass">)  [unwired: 7 in]
          n1090 = Equal?(x=w2860, y="DONE") -> (x = y?=w2846:bool)
          n1091 = case shown="True" w2847 {
            tunnel: [w2862 0] -> w2849
            tunnel: w2848 -> [w2863 _]
            tunnel: w2846 -> [w2861 _]
            frame False {
              n1092 = case shown="False" w2861 {
                tunnel: [w2864 w2865] -> w2862
                tunnel: w2863 -> [w2864 w2866]
                frame False {
                }
                frame True {
                  n1093 = Increment(x=w2866) -> (x+1=w2865:i32)
                }
              }
            }
            frame True {
            }
          }
        }
        frame 320 {
          # "Carrega timeout de 50 ciclos\npara resposta do ACS"
          n1094 = call-dynamic "Write Timer.vi"("error in (no error)"=w2875, "Timer"=u32 50, "State Machine in"=w2874) -> ("error out"=w2877:errorcluster, "State Machine out"=w2879:refnum<class "State Machine.lvclass">)  [unwired: 7 in]
          n1095 = call-dynamic "Write State Machine.vi"("error in (no error)"=w2877, "State Machine.lvclass"=w2879, "Device in"=w2876) -> ("error out"=w2870:errorcluster, "Device out"=w2869:refnum<class "Channel.lvclass">)  [unwired: 7 in]
          n1096 = Unbundle By Name(w2869) -> ("ICS mode"=w2868:string)
          n1097 = Concatenate Strings("SET ICSMODE " ("cmd"), w2868) -> (w2871:string)
          n1098 = call-dynamic "Write cmd.vi"("error in (no error)"=w2870, "cmd"=w2871, "Device in"=w2869) -> ("error out"=w2881:errorcluster, "Device out"=w2882:refnum<class "Channel.lvclass">)  [unwired: 7 in]
          n1099 = Increment(x=w2873) -> (x+1=w2880:i32)
        }
        frame 321 {
          n1100 = call "Verify Timer.vi"("error in (no error)"=w2887, "State Machine in"=w2888) -> ("error out"=w2892:errorcluster, "timeout"=w2886:bool, "State Machine out"=w2893:refnum<class "State Machine.lvclass">)  [unwired: 7 in]
          n1101 = call-dynamic "Write State Machine.vi"("error in (no error)"=w2892, "State Machine.lvclass"=w2893, "Device in"=w2891) -> ("error out"=w2889:errorcluster, "Device out"=w2890:refnum<class "Channel.lvclass">)  [unwired: 7 in]
          n1102 = call-dynamic "Read resp.vi"("error in (no error)"=w2889, "Device in"=w2890) -> ("error out"=w2894:errorcluster, "resp"=w2897:string, "Device out"=w2895:refnum<class "Channel.lvclass">)  [unwired: 7 in]
          n1103 = Equal?(x=w2897, y="DONE") -> (x = y?=w2884:bool)
          n1104 = case shown="True" w2886 {
            tunnel: [w2899 w2905] -> w2883
            tunnel: w2885 -> [w2900 _]
            tunnel: w2884 -> [w2898 _]
            frame False {
              n1105 = case shown="True" w2898 {
                tunnel: [w2901 w2902] -> w2899
                tunnel: w2900 -> [w2901 _]
                frame False {
                }
                frame True {
                  n1106 = disable-structure shown="Enabled" {
                    disable-tunnel: [0 ("State") 40] -> w2902
                    frame Disabled {
                    }
                    frame Enabled {
                      # "Configura\nExpMode"
                    }
                  }
                }
              }
            }
            frame True {
              n1107 = disable-structure shown="Enabled" {
                disable-tunnel: [0 40] -> w2905
                frame Enabled {
                }
                frame Disabled {
                  # "Configura\nExpMode"
                }
              }
            }
          }
        }
      }
      n1108 = call-dynamic "Read State Machine.vi"("error in (no error)"=w7, "Device in"=w14) -> ("error out"=w10:errorcluster, "State Machine.lvclass"=w13:refnum<class "State Machine.lvclass">, "Device out"=w12:refnum<class "Channel.lvclass">)  [unwired: 7 in]
      n1109 = call "Next State.vi"("error in (no error)"=w10, "New_State"=w8, "State Machine in"=w13) -> ("error out"=w9:errorcluster, "State Machine out"=w15:refnum<class "State Machine.lvclass">)  [unwired: 7 in]
      n1110 = call-dynamic "Write State Machine.vi"("error in (no error)"=w9, "State Machine.lvclass"=w15, "Device in"=w12) -> ("error out"=w6:errorcluster, "Device out"=w11:refnum<class "Channel.lvclass">)  [unwired: 7 in]
    }
    frame Error {
    }
  }
  "error out" <- w3
  "Channel out" <- w1
